vi "Digilens IPLC UI.vi"() -> ()   [LabVIEW 2022 SP3, in "TopLevel.lvclass"]
uses:
  TopLevel.lvclass
  IO/Typedefs/Pre Purge Parameters.ctl
  Motor Controller/Typedefs/API Command Cluster.ctl
  Motor Controller/Typedefs/API Command Enum.ctl
  Motor Controller/Typedefs/SetExplicitMessage API Data.ctl
  Motor Controller/Typedefs/Motor Controller Parameter-Set.ctl
  Motor Controller/Typedefs/Motor Controller Parameter-Get.ctl
  Typedefs/API Command Enum.ctl
  IO/Typedefs/ICP2-DO Channel Names.ctl
  IO/Typedefs/ICP1-D0 Channel Names.ctl
  Typedefs/API Command Cluster.ctl
  GIS Printer/Typedefs/PrintCmdParameters--Cluster.ctl
  GIS Printer/Typedefs/IdlePrintCmdParameters--Cluster.ctl
  IO/Typedefs/ICP1-AO Channel Names.ctl
  IO/Typedefs/ICP2-AO Channel Names.ctl
  IO/IO.lvclass
  GIS Printer/GIS Printer.lvclass
  Motor Controller/Motor Controller.lvclass
  Motor Controller/Typedefs/Status.ctl
  Typedefs/Motor Controller Config Data.ctl
  Motor Controller/Typedefs/Stage Move Data.ctl
  Motor Controller/Typedefs/Batch Index Speed Data.ctl
  Motor Controller/Typedefs/Move Status.ctl
  Typedefs/Digilens Config Cluster.ctl
  IO/Typedefs/IO Config Data.ctl
  IO/Typedefs/DCON_DeviceConfig--Cluster.ctl
  IO/Typedefs/Channel Data.ctl
  GIS Printer/Typedefs/PrinterConfiguration--Cluster.ctl
  DAQWFE/LV_Source/Subsystems/DAQ/DataTypes/TD DAQ Settings--cluster.ctl
  DAQWFE/LV_Source/Subsystems/DAQ/DataTypes/TD DI Instrument Settings--cluster.ctl
  DAQWFE/LV_Source/Subsystems/DAQ/DataTypes/TD AI Instrument Settings--cluster.ctl
  DAQWFE/LV_Source/Subsystems/DAQ/DataTypes/TD AI InstSettings--cluster.ctl
  DAQWFE/LV_Source/Subsystems/DAQ/Process/ProcessSupport/TD SimAI Ranges--cluster.ctl
  IO/Typedefs/Status Cluster.ctl
  IO/Typedefs/ICP2-DI Channel Names.ctl
  IO/Typedefs/ICP1-AI Channel Names.ctl
  Motor Controller/Typedefs/Status_TopLevel--Cluster.ctl
  IO/Typedefs/Device Names.ctl
  IO/Typedefs/DCON Action Engine-States.ctl
  DAQWFE/LV_Source/Subsystems/DAQ/DAQ.lvclass
panel:
  in  "Exit":bool
  in  "update":bool
  out "H 6":dbl
  out "H 5":dbl
  out "H 4":dbl
  out "H 3":dbl
  out "H 2":dbl
  out "H1":dbl
  in  "Tab Control":T1(tab)
  out "Print #":i32=1 min=1 step=1
  in  "HomeOnComplete":bool
  out "Stage Busy Printer":bool caption="Busy"
  in  "PH6-Prime":bool
  in  "PH5-Prime":bool
  in  "PH4-Prime":bool
  in  "PH3-Prime":bool
  in  "PH2-Prime":bool
  in  "PH1-Prime":bool
  in  "Abort":bool
  in  "Print Passes":i32=1 min=1 step=1
  in  "Home 2":bool
  in  "TCP Commands & Responses":i32(listbox)
  in  "Print":bool
  in  "Command File Path":path
  in  "Jog (+) 2":bool
  in  "Jog (-) 2":bool
  in  "Idle Intervals (s)":dbl=0.1
  in  "IdlePrint":bool
  in  "Head1 2":bool
  in  "Head2 2":bool
  in  "Head3 2":bool
  in  "Head4 2":bool
  in  "Head5 2":bool
  in  "Head6 2":bool
  in  "Enable PH1 Heat":bool
  in  "Enable PH2 Heat":bool
  in  "Enable PH3 Heat":bool
  in  "Enable PH4 Heat":bool
  in  "Enable PH5 Heat":bool
  in  "Enable PH6 Heat":bool
  in  "10Pass":bool
  in  "5Pass":bool
  in  "Enable Disable With DO":bool
  in  "Stage Abort":bool
  in  "ClearStageAlarm":bool
  out "Stage Busy (Stage)":bool caption="Stage Busy"
  in  "Print Speed":i32
  in  "Print (+)":bool
  in  "Print (-)":bool
  out "Status/Error :":string
  in  "Acceleration":dbl
  in  "Jog Speed":i32
  in  "Jog (+)":bool
  in  "Jog (-)":bool
  in  "Go":bool
  in  "Accel":dbl
  in  "Speed":i32
  in  "GoTo":i32
  out "Pulse/mm":dbl
  out "Position":dbl
  out "Enabled":bool
  in  "Enable Disable":bool
  in  "Head6":bool
  in  "Head5":bool
  in  "Head4":bool
  in  "Head3":bool
  in  "Head2":bool
  in  "Head1":bool
  in  "Home":bool
  in  "Laminate":bool
  in  "Load":bool
  in  "Read Status":bool
  out "Stage Busy (Moves)":bool caption="Stage Busy"
  out "Status":string
  in  "Stage Move Status":i32(listbox)
  in  "Start":bool
  in  "Stage Recipe XML File Path":path
  out "PrePrgPrint #":i32=1 min=1 step=1
  in  "PPDuration (s)":dbl=3.0
  in  "Pre Purge PH Ch-6 Parameters":T2={"GIS File Path"=path "", "Duration (s)"=0.1, "No. of Repeats"=1}
  in  "Pre Purge PH Ch-5 Parameters":T2={"GIS File Path"=path "", "Duration (s)"=0.1, "No. of Repeats"=1}
  in  "Pre Purge PH Ch-3 Parameters":T2={"GIS File Path"=path "", "Duration (s)"=0.1, "No. of Repeats"=1}
  in  "Pre Purge PH Ch-4 Parameters":T2={"GIS File Path"=path "", "Duration (s)"=0.1, "No. of Repeats"=1}
  in  "Pre Purge PH Ch-2 Parameters":T2={"GIS File Path"=path "", "Duration (s)"=0.1, "No. of Repeats"=1}
  in  "Pre Purge PH Ch-1 Parameters":T2={"GIS File Path"=path "", "Duration (s)"=0.1, "No. of Repeats"=1}
  in  "Pre Purge PH Ch-1":bool
  in  "Pre Purge PH Ch-2":bool
  in  "Pre Purge PH Ch-3":bool
  in  "Pre Purge PH Ch-4":bool
  in  "Pre Purge PH Ch-5":bool
  in  "Pre Purge PH Ch-6":bool
  out "Purge PH Ch-1":bool
  in  "Purge PH Ch-2":bool
  in  "Purge PH Ch-3":bool
  in  "Purge PH Ch-4":bool
  in  "Purge PH Ch-5":bool
  in  "Purge PH Ch-6":bool
  in  "Duration (s)":dbl=3.0
  in  "Jog (-) 3":bool
  in  "Jog (+) 3":bool
  in  "Head6 3":bool
  in  "Head5 3":bool
  in  "Head4 3":bool
  in  "Head3 3":bool
  in  "Head2 3":bool
  in  "Head1 3":bool
  in  "Home 3":bool
  in  "Spit 6":bool
  in  "Spit 5":bool
  in  "Spit 4":bool
  in  "Spit 3":bool
  in  "Spit 2":bool
  in  "Spit 1":bool
  in  "Spit 6 LOV":u16(ring)
  in  "Spit 5 LOV":u16(ring)
  in  "Spit 4 LOV":u16(ring)
  in  "Spit 3 LOV":u16(ring)
  in  "Spit 2 LOV":u16(ring)
  in  "Spit 1 LOV":u16(ring)
  out "Res 6 Meniscus":dbl
  out "Res 5 Meniscus":dbl
  out "Res 4 Meniscus":dbl
  out "Res 3 Meniscus":dbl
  out "Res 2 Meniscus":dbl
  out "Res 1 Meniscus":dbl
  in  "Res 6 Recirculate":dbl
  in  "Res 5 Recirculate":dbl
  in  "Res 4 Recirculate":dbl
  in  "Res 3 Recirculate":dbl
  in  "Res 2 Recirculate":dbl
  in  "Res 1 Recirculate":dbl
  in  "Res 6 Enabled":bool
  in  "Res 5 Enabled":bool
  in  "Res 4 Enabled":bool
  in  "Res 3 Enabled":bool
  in  "Res 2 Enabled":bool
  in  "Res 1 Enabled":bool
  in  "Head 6 Set":bool
  in  "Head 6 Set Temp":dbl
  out "Head 6 Act Temp":dbl
  in  "Head 5 Set":bool
  in  "Head 5 Set Temp":dbl
  out "Head 5 Act Temp":dbl
  in  "Head 4 Set":bool
  in  "Head 4 Set Temp":dbl
  out "Head 4 Act Temp":dbl
  in  "Head 3 Set":bool
  in  "Head 3 Set Temp":dbl
  out "Head 3 Act Temp":dbl
  in  "Head 2 Set":bool
  in  "Head 2 Set Temp":dbl
  out "Head 2 Act Temp":dbl
  in  "Head 1 Set":bool
  in  "Head 1 Set Temp":dbl
  out "Head 1 Act Temp":dbl
  in  "Head 6 Material":u16(ring) items=["none", "113A.3", "507.2-1", "109G"]
  in  "Head 5 Material":u16(ring) items=["none", "113A.3", "507.2-1", "109G"]
  in  "Head 4 Material":u16(ring) items=["none", "113A.3", "507.2-1", "109G"]
  in  "Head 3 Material":u16(ring) items=["none", "113A.3", "507.2-1", "109G"]
  in  "Head 2 Material":u16(ring) items=["none", "113A.3", "507.2-1", "109G"]
  in  "Enable Ink Ch-6":bool
  in  "Enable Ink Ch-5":bool
  in  "Enable Ink Ch-4":bool
  in  "Enable Ink Ch-3":bool
  in  "Enable Ink Ch-2":bool
  in  "Enable Ink Ch-1":bool
  in  "Head 1 Material":u16(ring) items=["none", "113A.3", "507.2-1", "109G"]
  out "SW - COVER INPUT SIDE (M)":bool
  out "SW - COVER OUTPUT SIDE (M)":bool
  out "Purge Valve Open - R6 Status":bool
  out "Purge Valve Open - R5 Status":bool
  out "Purge Valve Open - R4 Status":bool
  out "Purge Valve Open - R3 Status":bool
  out "Purge Valve Open - R2 Status":bool
  out "Purge Valve Open - R1 Status":bool
  out "Meniscus Pressure Reg PWR - R6 Status":bool
  out "Meniscus Pressure Reg PWR - R5 Status":bool
  out "Meniscus Pressure Reg PWR - R4 Status":bool
  out "Meniscus Pressure Reg PWR - R3 Status":bool
  out "Meniscus Pressure Reg PWR - R2 Status":bool
  out "Meniscus Pressure Reg PWR - R1 Status":bool
  out "Recirc Pump On - R6 Status":bool
  out "Recirc Pump On - R5 Status":bool
  out "Recirc Pump On - R4 Status":bool
  out "Recirc Pump On - R3 Status":bool
  out "Recirc Pump On - R2 Status":bool
  out "Recirc Pump On - R1 Status":bool
  out "SW_LED - Ink Valve - R6 Status":bool
  out "SW_LED - Ink Valve - R5 Status":bool
  out "SW_LED - Ink Valve - R4 Status":bool
  out "SW_LED - Ink Valve - R3 Status":bool
  out "SW_LED - Ink Valve - R2 Status":bool
  out "SW_LED - Ink Valve - R1 Status":bool
  out "Ink Flow Valve Open - R5 Status":bool
  out "Ink Flow Valve Open - R4 Status":bool
  out "Ink Flow Valve Open - R3 Status":bool
  out "Ink Flow Valve Open - R2 Status":bool
  out "Ink Flow Valve Open - R1 Status":bool
  out "Meniscus Valve Open - R6 Status":bool
  out "Meniscus Valve Open - R5 Status":bool
  out "Meniscus Valve Open - R4 Status":bool
  out "Meniscus Valve Open - R3 Status":bool
  out "Ink Flow Valve Open - R6 Status":bool
  out "Meniscus Valve Open - R2 Status":bool
  out "Meniscus Valve Open - R1 Status":bool
  in  "Purge Valve Open - R6":bool
  in  "Purge Valve Open - R5":bool
  in  "Purge Valve Open - R4":bool
  in  "Purge Valve Open - R3":bool
  in  "Purge Valve Open - R2":bool
  in  "Purge Valve Open - R1":bool
  in  "Meniscus Pressure Reg PWR - R6":bool
  in  "Meniscus Pressure Reg PWR - R5":bool
  in  "Meniscus Pressure Reg PWR - R4":bool
  in  "Meniscus Pressure Reg PWR - R3":bool
  in  "Meniscus Pressure Reg PWR - R2":bool
  in  "Meniscus Pressure Reg PWR - R1":bool
  in  "Recirc Pump On - R6":bool
  in  "Recirc Pump On - R5":bool
  in  "Recirc Pump On - R4":bool
  in  "Recirc Pump On - R3":bool
  in  "Recirc Pump On - R2":bool
  in  "Recirc Pump On - R1":bool
  in  "SW_LED - Ink Valve - R6":bool
  in  "SW_LED - Ink Valve - R5":bool
  in  "SW_LED - Ink Valve - R4":bool
  in  "SW_LED - Ink Valve - R3":bool
  in  "SW_LED - Ink Valve - R2":bool
  in  "SW_LED - Ink Valve - R1":bool
  in  "Ink Flow Valve Open - R6":bool
  in  "Ink Flow Valve Open - R5":bool
  in  "Ink Flow Valve Open - R4":bool
  in  "Ink Flow Valve Open - R3":bool
  in  "Ink Flow Valve Open - R2":bool
  in  "Ink Flow Valve Open - R1":bool
  in  "Meniscus Valve Open - R6":bool
  in  "Meniscus Valve Open - R5":bool
  in  "Meniscus Valve Open - R4":bool
  in  "Meniscus Valve Open - R3":bool
  in  "Meniscus Valve Open - R2":bool
  out "SW - Purge - R6":bool
  out "SW - Purge - R5":bool
  out "SW - Purge - R4":bool
  out "SW - Purge - R3":bool
  out "SW - Purge - R1":bool
  out "SW - Purge - R2":bool
  out "SW - COVER OUTPUT SIDE":bool
  out "SW - COVER INPUT SIDE":bool
  out "SW - Ink Valve - R6":bool
  out "SW - Ink Valve - R5":bool
  out "SW - Ink Valve - R4":bool
  out "SW - Ink Valve - R3":bool
  out "SW - Ink Valve - R1":bool
  out "SW - Ink Valve - R2":bool
  in  "Meniscus Valve Open - R1":bool
  out "Recirc Pump Flow Set - R6 Status":dbl
  out "Recirc Pump Flow Set - R5 Status":dbl
  out "Recirc Pump Flow Set - R4 Status":dbl
  out "Recirc Pump Flow Set - R3 Status":dbl
  out "Recirc Pump Flow Set - R2 Status":dbl
  out "Recirc Pump Flow Set - R1 Status":dbl
  out "Meniscus Pressure Set - R6 Status":dbl
  out "Meniscus Pressure Set - R5 Status":dbl
  out "Meniscus Pressure Set - R4 Status":dbl
  out "Meniscus Pressure Set - R3 Status":dbl
  out "Meniscus Pressure Set - R2 Status":dbl
  out "Meniscus Pressure Set - R1 Status":dbl
  in  "Recirc Pump Flow Set - R6 Set":bool
  in  "Recirc Pump Flow Set - R5 Set":bool
  in  "Recirc Pump Flow Set - R4 Set":bool
  in  "Recirc Pump Flow Set - R3 Set":bool
  in  "Recirc Pump Flow Set - R2 Set":bool
  in  "Recirc Pump Flow Set - R1 Set":bool
  in  "Recirc Pump Flow Set - R6":dbl
  in  "Recirc Pump Flow Set - R5":dbl
  in  "Recirc Pump Flow Set - R4":dbl
  in  "Recirc Pump Flow Set - R3":dbl
  in  "Recirc Pump Flow Set - R2":dbl
  in  "Recirc Pump Flow Set - R1":dbl
  in  "Meniscus Pressure Set - R6-Set":bool
  in  "Meniscus Pressure Set - R5-Set":bool
  in  "Meniscus Pressure Set - R4-Set":bool
  in  "Meniscus Pressure Set - R3-Set":bool
  in  "Meniscus Pressure Set - R2-Set":bool
  in  "Meniscus Pressure Set - R1-Set":bool
  in  "Meniscus Pressure Set - R6":dbl
  in  "Meniscus Pressure Set - R5":dbl
  in  "Meniscus Pressure Set - R4":dbl
  in  "Meniscus Pressure Set - R3":dbl
  in  "Meniscus Pressure Set - R2":dbl
  in  "Meniscus Pressure Set - R1":dbl
  out "Meniscus Pressure Read - R6":dbl
  out "Meniscus Pressure Read - R5":dbl
  out "Meniscus Pressure Read - R4":dbl
  out "Meniscus Pressure Read - R3":dbl
  out "Meniscus Pressure Read - R2":dbl
  out "Meniscus Pressure Read - R1":dbl
  out "TopLevel Out":refnum<class "TopLevel.lvclass">
  in  "TopLevel In":refnum<class "TopLevel.lvclass">
  # "PrePrint"
  # "Move to Position"
  # "Prepurge Script File Path"
  # "Repeat Interval (s)"
  # "Repeats"
  # "Purge"
  # "1"
  # "2"
  # "3"
  # "4"
  # "5"
  # "6"
  # "Covered"
  # "Head Temp"
  # "Reservoir"
  # "Head"
  # "En"
  # "Material"
  # "Actual"
  # "Set"
  # "Recirculate"
  # "Meniscus"
  # "Spit"
  # "1"
  # "1"
  # "1"
  # "1"
  # "1"
  # "2"
  # "2"
  # "2"
  # "2"
  # "2"
  # "3"
  # "3"
  # "3"
  # "3"
  # "3"
  # "4"
  # "4"
  # "4"
  # "4"
  # "4"
  # "5"
  # "5"
  # "5"
  # "5"
  # "5"
  # "6"
  # "6"
  # "6"
  # "6"
  # "6"
  # "ICP2-DI"
  # "ICP2-DO"
  # "ICP1-DO"
  # "ICP1-AI"
  # "ICP1-AO"
  # "ICP2-AO"
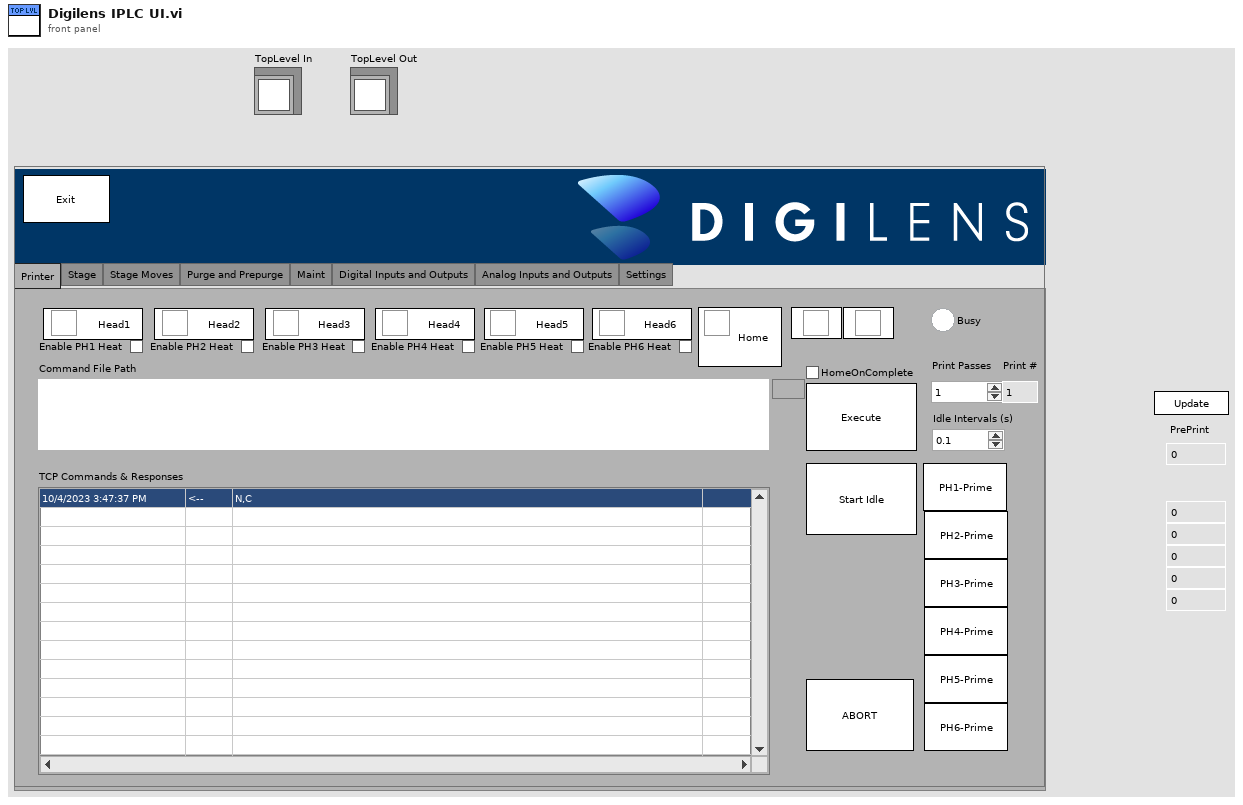
[diagram p1: front panel]
types:
  T1 = enum32{"Printer", "Stage", "Stage Moves", "Purge and Prepurge", "Maint", "Digital Inputs and Outputs", "Analog Inputs and Outputs", "Settings"}
  T2 = typedef "TopLevel.lvclass/Pre Purge Parameters.ctl" = cluster{"GIS File Path":path, "Duration (s)":dbl, "No. of Repeats":i32}
  T3 = typedef "Motor Controller.lvclass/SetExplicitMessage API Data.ctl" = cluster{"Motor Controller Parameter":T4, "value":i32}
  T4 = typedef "Motor Controller.lvclass/Motor Controller Parameter-Set.ctl" = enum16{"Print Speed", "Jog Speed", "PR Path", "Enable Servo", "Disable Servo", "Move Stage to Under PH1", "Move Stage to Under PH2", "Move Stage to Under PH3", "Move Stage to Under PH4", "Move Stage to Under PH5", "Move Stage to Under PH6", "Home Stage", "Return Stage to 0", "Print Stage", "Write Speed", "Write Index", "Stop Stage"}
  T5 = typedef "Motor Controller.lvclass/API Command Enum.ctl" = enum16{"GetExplicitMessage", "SetExplicitMessage", "Execute Stage Move Recipe", "Read Stage Move Recipe", "Abort"}
  T6 = typedef "Motor Controller.lvclass/API Command Cluster.ctl" = cluster{"Command":T5, "Arguments":string, "Data":variant}
  T7 = typedef "Motor Controller.lvclass/Motor Controller Parameter-Get.ctl" = enum16{"Print Speed", "Jog Speed", "PR Path", "Servo Enabled?", "AlarmCodes"}
  T8 = typedef "TopLevel.lvclass/API Command Enum.ctl" = enum16{"Execute Printer Commands", "Pre Purge", "Enable Ink Ch-1", "Enable Ink Ch-2", "Enable Ink Ch-3", "Enable Ink Ch-4", "Enable Ink Ch-5", "Enable Ink Ch-6", "Disable Ink Ch-1", "Disable Ink Ch-2", "Disable Ink Ch-3", "Disable Ink Ch-4", "Disable Ink Ch-5", "Disable Ink Ch-6", "ExecuteIdlePrintCycle", "StopIdlePrintCycle", "Abort", "LoadDLP2GUIConfig", "SaveDLP2GUIConfig", "PrimingMode", "SetHeadTemperature", "EnableHead", "EnableHeadHeat", "SetSystemMode", "HeadPrint", "AbortAll", "Send Printer String", "WriteInitXML"}
  T9 = typedef "IO.lvclass/ICP2-DO Channel Names.ctl" = enum16{"None", "Meniscus Valve Open - R1", "Meniscus Valve Open - R2", "Meniscus Valve Open - R3", "Meniscus Valve Open - R4", "Meniscus Valve Open - R5", "Meniscus Valve Open - R6", "Ink Flow Valve Open - R1", "Ink Flow Valve Open - R2", "Ink Flow Valve Open - R3", "Ink Flow Valve Open - R4", "Ink Flow Valve Open - R5", "Ink Flow Valve Open - R6", "SW_LED - Ink Valve - R1", "SW_LED - Ink Valve - R2", "SW_LED - Ink Valve - R3", "Recirc Pump On - R1", "Recirc Pump On - R2", "Recirc Pump On - R3", "Recirc Pump On - R4", "Recirc Pump On - R5", "Recirc Pump On - R6", "SW_LED - Ink Valve - R4", "SW_LED - Ink Valve - R5", "SW_LED - Ink Valve - R6"}
  T10 = typedef "IO.lvclass/ICP1-D0 Channel Names.ctl" = enum16{"None", "Meniscus Pressure Reg PWR - R1", "Meniscus Pressure Reg PWR - R2", "Meniscus Pressure Reg PWR - R3", "Meniscus Pressure Reg PWR - R4", "Meniscus Pressure Reg PWR - R5", "Meniscus Pressure Reg PWR - R6", "Clear Stage Alarm", "Servo ON", "Purge Valve Open - R1", "Purge Valve Open - R2", "Purge Valve Open - R3", "Purge Valve Open - R4", "Purge Valve Open - R5", "Purge Valve Open - R6"}
  T11 = typedef "PrintCmdParameters--Cluster.ctl" = cluster{"Command File Path":path, "No. of Print Repeats":i32, "HomeOnComplete":bool}
  T12 = typedef "TopLevel.lvclass/API Command Cluster.ctl" = cluster{"Command":T8, "Arguments":string, "Data":variant}
  T13 = typedef "IdlePrintCmdParameters--Cluster.ctl" = cluster{"Command File Path":path, "IdleMode":bool, "IdleCycleInterval(s)":dbl}
  T14 = typedef "IO.lvclass/ICP1-AO Channel Names.ctl" = enum16{"None", "Meniscus Pressure Set - R1", "Meniscus Pressure Set - R2", "Meniscus Pressure Set - R3", "Meniscus Pressure Set - R4", "Meniscus Pressure Set - R5", "Meniscus Pressure Set - R6", "Meniscus Vac Pump Speed"}
  T15 = typedef "IO.lvclass/ICP2-AO Channel Names.ctl" = enum16{"None", "Recirc Pump Flow Set - R1", "Recirc Pump Flow Set - R2", "Recirc Pump Flow Set - R3", "Recirc Pump Flow Set - R4", "Recirc Pump Flow Set - R5", "Recirc Pump Flow Set - R6"}
  T16 = enum32{"invalid app kind", "Development System", "Run Time System", "Student Edition", "Embedded LabVIEW", "Evaluation", "Custom"}
  T17 = typedef "Motor Controller.lvclass/Status.ctl" = cluster{"Motor Controller Config Data":T18, "Motor Controller Data":cluster{"Enabled?":bool}, "Stage Move":T19, "Stage Busy?":bool}
  T18 = typedef "Motor Controller.lvclass/Motor Controller Config Data.ctl" = cluster{"Motor IP Addresss":string, "Current Position":i32, "Pulse_Per_mm":i32, "PrePrint":dbl[], "Load Position_mm":i32, "Laminate Position_mm":i32}
  T19 = typedef "Motor Controller.lvclass/Stage Move Data.ctl" = cluster{"Current Step":string, "Move Data":T20[]}
  T20 = typedef "Motor Controller.lvclass/Batch Index Speed Data.ctl" = cluster{"Batch & Cycle":string, "Move":cluster{"Index_mm":i32, "Speed_mm_s":i32}, "Status":T21}
  T21 = typedef "Motor Controller.lvclass/Move Status.ctl" = enum16{"Pending", "In Progress", "Completed"}
  T22 = enum8{"Enabled", "Disabled", "Disabled and Grayed Out"}
  T23 = enum32{"Invalid", "Standard", "Closed", "Hidden", "Minimized", "Maximized"}
  T24 = typedef "DCON Action Engine-States.ctl" = enum16{"Open", "Close", "Set DO Value", "Get Digital Status", "Get Data", "Get AI Status", "Set AO Value", "Get AO Status"}
  T25 = typedef "IO.lvclass/Device Names.ctl" = enum16{"ICP1-DO", "ICP2-DI", "ICP2-DO", "ICP1-AI", "ICP1-AO", "ICP2-AO"}
  T26 = typedef "TopLevel.lvclass/Digilens Config Cluster.ctl" = cluster{"Motion Controller":T18, "IO Config":T27, "PrinterConfiguration":T30, "DAQ Settings":T31}
  T27 = typedef "IO.lvclass/IO Config Data.ctl" = cluster{"DAQDevices":T28[], "DI Channels":T29[], "DO Channels":T29[], "Material Names":string[], "AI Channels":T29[], "AO Channels":T29[]}
  T28 = typedef "IO.lvclass/DCON_DeviceConfig--Cluster.ctl" = cluster{"COM":string, "DeviceName":string, "BaudRate":u32, "Number of Channels":i32, "DeviceAddress":i32, "Enable":bool}
  T29 = typedef "IO.lvclass/Channel Data.ctl" = cluster{"Channel Name":string, "Device Name":string, "Channel No":string}
  T30 = typedef "GIS Printer.lvclass/PrinterConfiguration--Cluster.ctl" = cluster{"IPAddress":string, "Move Stage on RTP Command?":bool, "Stage Move Position":string, "PH1-Prime Path":path, "PH2-Prime Path":path, "PH3-Prime Path":path, "PH4-Prime Path":path, "PH5-Prime Path":path, "PH6-Prime Path":path, "PrintScriptsFolder":path, "PurgeScriptsFolder":path, "StageScriptsFolder":path, "PH1-HeatOn Path":path, "PH2-HeatOn Path":path, "PH3-HeatOn Path":path, "PH4-HeatOn Path":path, "PH5-HeatOn Path":path, "PH6-HeatOn Path":path, "PH1-HeatOff Path":path, "PH2-HeatOff Path":path, "PH3-HeatOff Path":path, "PH4-HeatOff Path":path, "PH5-HeatOff Path":path, "PH6-HeatOff Path":path}
  T31 = typedef "DAQ.lvclass/TD DAQ Settings--cluster.ctl" = cluster{"Simulate DAQ":bool, "DI Settings":T32[], "AI Settings":T33[], "Relay IONames":string[], "AO IONames":string[], "AO NChan SingleTask":bool}
  T32 = typedef "DAQ.lvclass/TD DI Instrument Settings--cluster.ctl" = cluster{"Disable":bool, "DI TaskName":string, "DI RefreshIntv":i32}
  T33 = typedef "DAQ.lvclass/TD AI Instrument Settings--cluster.ctl" = cluster{"Disable":bool, "AI TaskName":string, "AI InstSettings":T34, "SimAI Ranges":T35}
  T34 = typedef "DAQ.lvclass/TD AI InstSettings--cluster.ctl" = cluster{"DaqRate":dbl, "NumSamples":i32}
  T35 = typedef "DAQ.lvclass/TD SimAI Ranges--cluster.ctl" = cluster{"lo":dbl, "hi":dbl}
  T36 = cluster{"Core":cluster{"Current VI Reference":refnum<vi>, "Close Panel on Exit?":bool}, "IO":refnum<class "IO.lvclass">, "GIS Printer":refnum<class "GIS Printer.lvclass">, "Motor Controller":refnum<class "Motor Controller.lvclass">, "Methods:Accessors:Digilens Config":T26, "Status":T17, "Exit Event":refnum<user-event>, "Purge\\PrePurge Channel Name":T10, "Pre Purge Parameters":T2, "API Command":T8, "TopLevel out":refnum<class "TopLevel.lvclass">}
  T37 = cluster{"Current VI Reference":refnum<vi>, "Close Panel on Exit?":bool}
  T38 = typedef "TopLevel.lvclass/UserEvents.ctl" = cluster{"API Incoming Event":refnum<user-event>, "API Executed Event":refnum<user-event>, "API Return Event":refnum<user-event>, "Exit Event":refnum<user-event>, "StatusChanged":refnum<user-event>, "DLP GUI Config Changed":refnum<user-event>, "AppEvent":refnum<user-event>, "Login Event":refnum<user-event>, "HeadPrimeStatusEvent":refnum<user-event>}
  T39 = typedef "Motor Controller.lvclass/UserEvents.ctl" = cluster{"API Incoming Event":refnum<user-event>, "API Executed Event":refnum<user-event>, "API Return Event":refnum<user-event>, "Status Changed Event":refnum<user-event>, "StopEvent":refnum<user-event>}
  T40 = typedef "IO.lvclass/UserEvents.ctl" = cluster{"API Incoming Event":refnum<user-event>, "API Executed Event":refnum<user-event>, "API Return Event":refnum<user-event>, "Status Changed Event":refnum<user-event>}
  T41 = typedef "GIS Printer.lvclass/UserEvents.ctl" = cluster{"API Incoming Event":refnum<user-event>, "API Executed Event":refnum<user-event>, "API Return Event":refnum<user-event>, "Status Changed Event":refnum<user-event>, "Abort":refnum<user-event>, "stop process":refnum<user-event>, "GISPollStatus":refnum<user-event>, "GISHeadStatus":refnum<user-event>, "Error Event":refnum<user-event>}
  T42 = typedef "IO.lvclass/DCON Private Data.ctl" = cluster{"DeviceName":string, "Number of Channels":i32, "COM":refnum<visa-resource-name>, "Status String":string, "Input String":string, "Value ":i32, "Digital Bits Value":bool[], "Analog Values":dbl[], "DeviceAddress":i32, "Enable":bool}
  T43 = typedef "IO.lvclass/ICP2-DI Channel Names.ctl" = enum16{"None", "SW - Ink Valve - R1", "SW - Ink Valve - R2", "SW - Ink Valve - R3", "SW - Ink Valve - R4", "SW - Ink Valve - R5", "SW - Ink Valve - R6", "SW - COVER INPUT SIDE", "SW - COVER OUTPUT SIDE", "SW - Purge - R1", "SW - Purge - R2", "SW - Purge - R3", "SW - Purge - R4", "SW - Purge - R5", "SW - Purge - R6"}
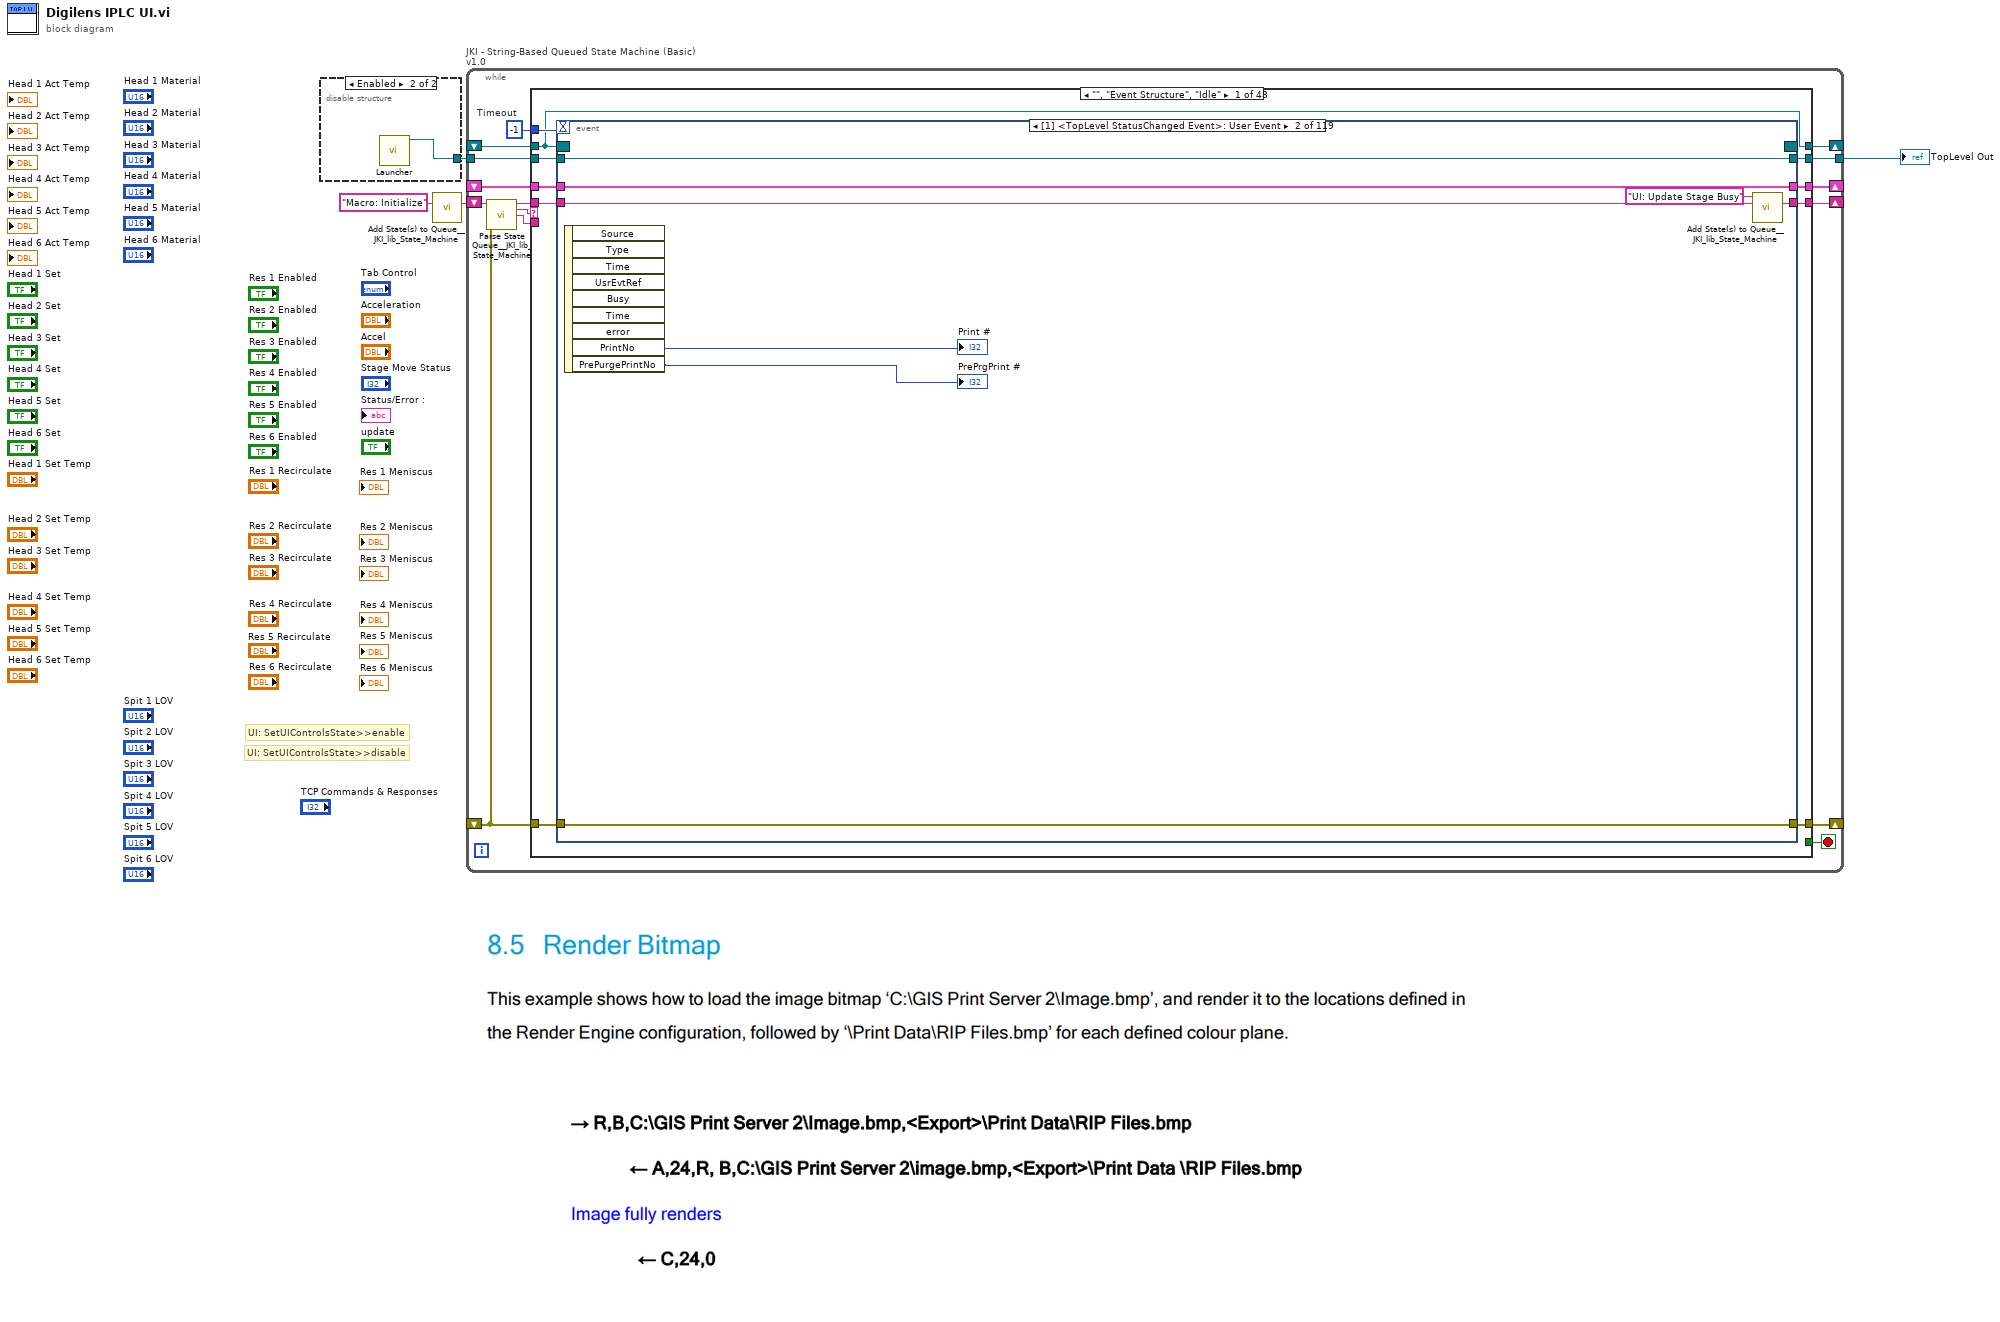
[diagram p0: block diagram]
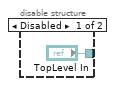
[diagram p2: hidden frame]
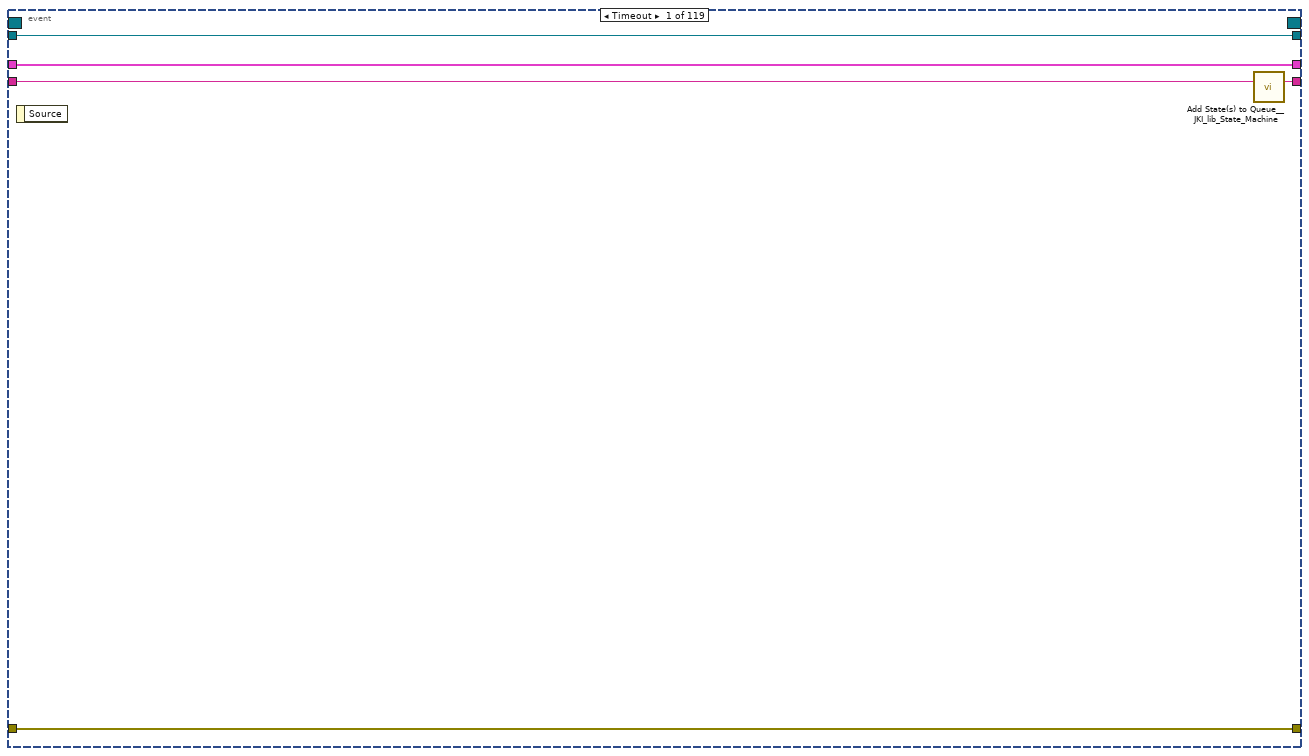
[diagram p3: hidden frame]
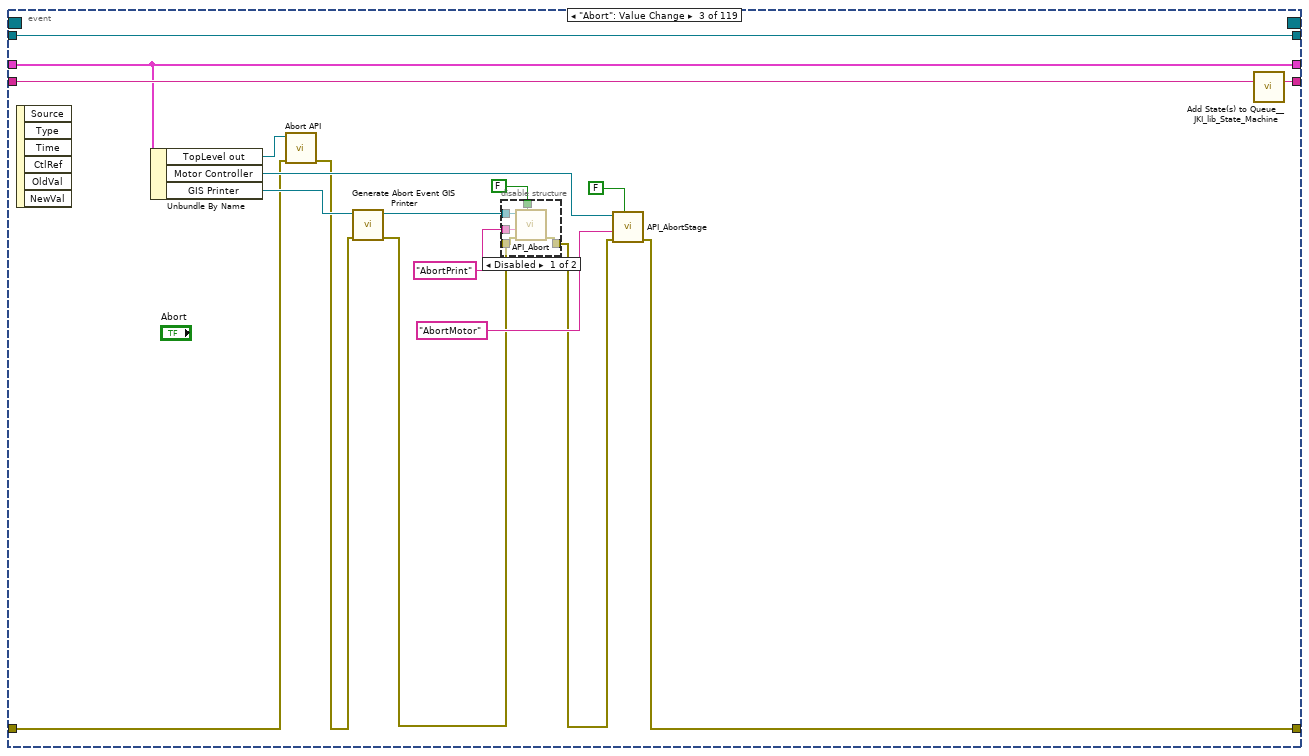
[diagram p4: hidden frame]
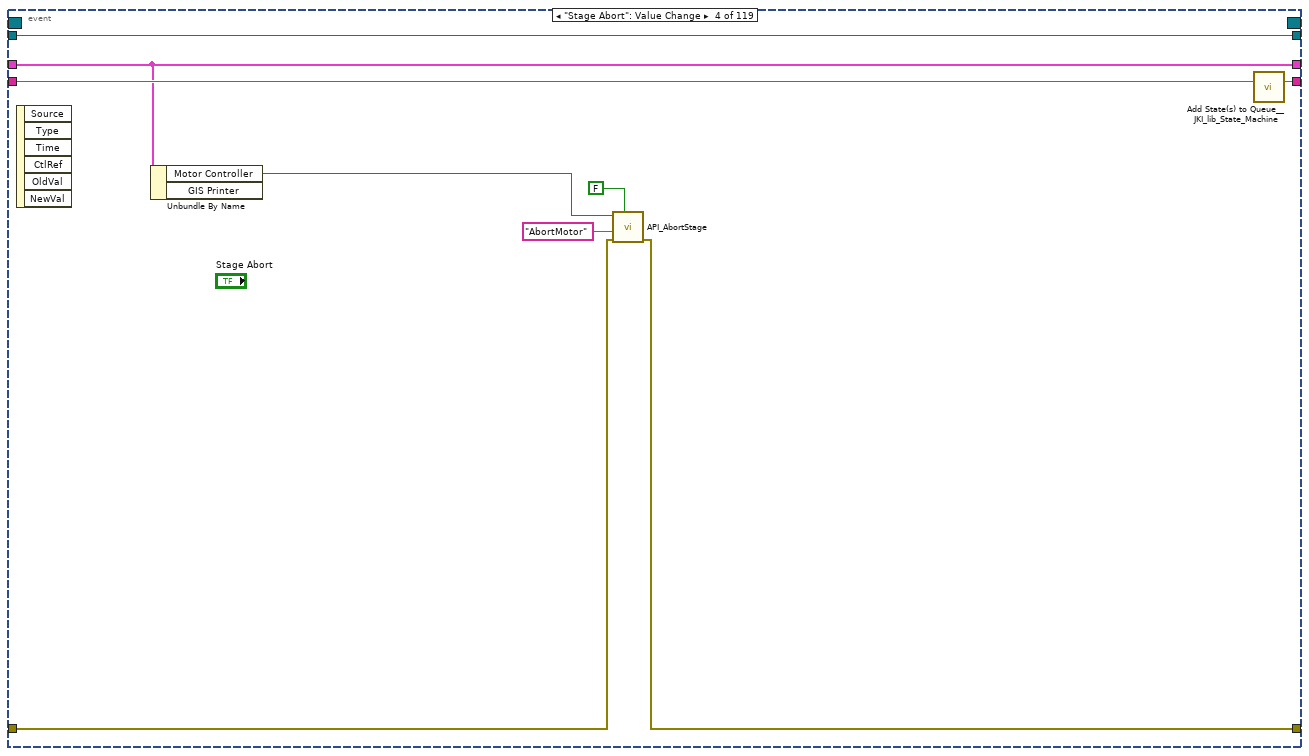
[diagram p6: hidden frame]
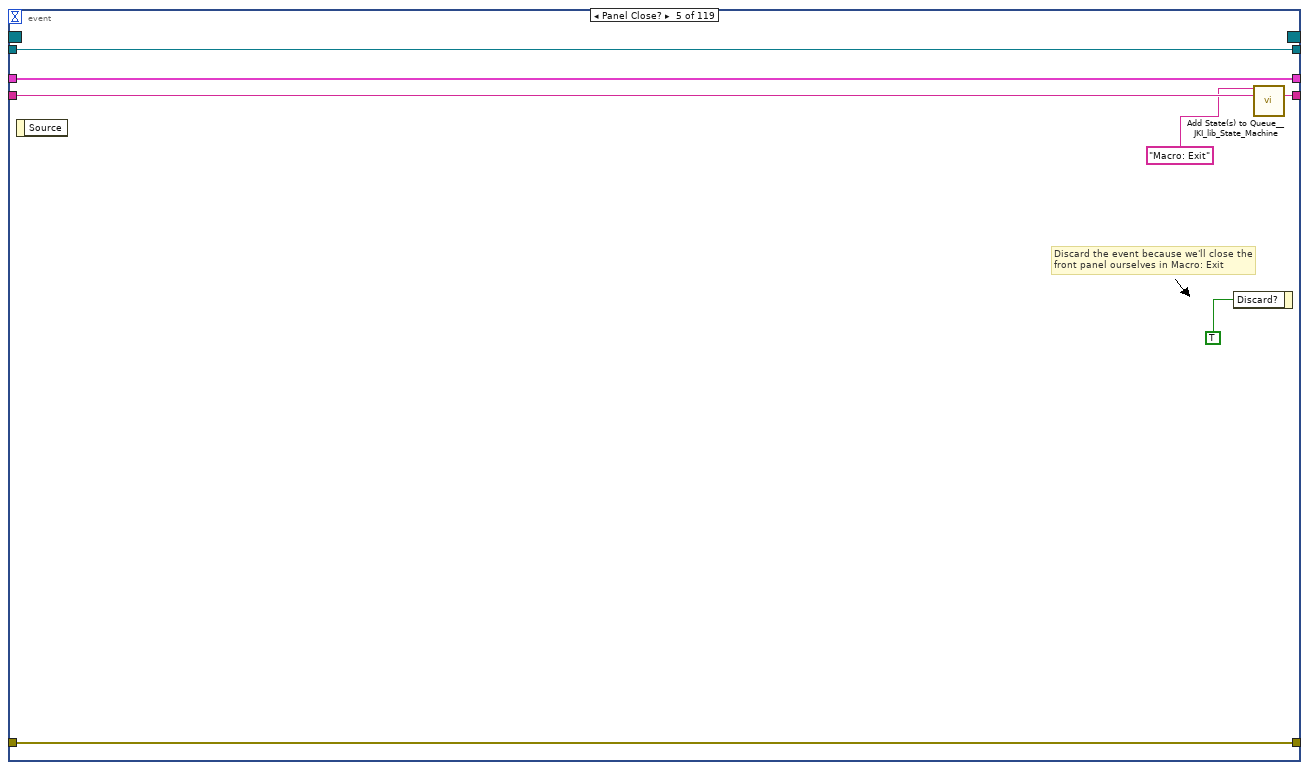
[diagram p7: hidden frame]
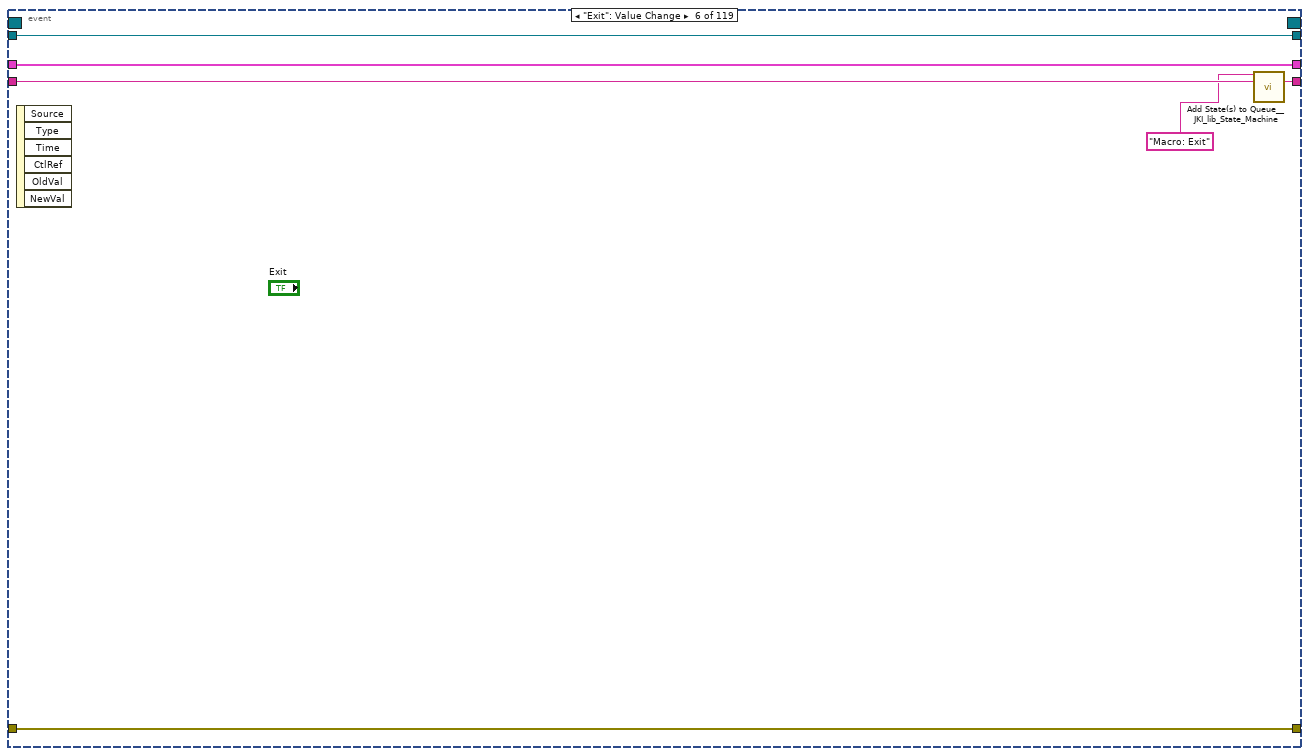
[diagram p8: hidden frame]
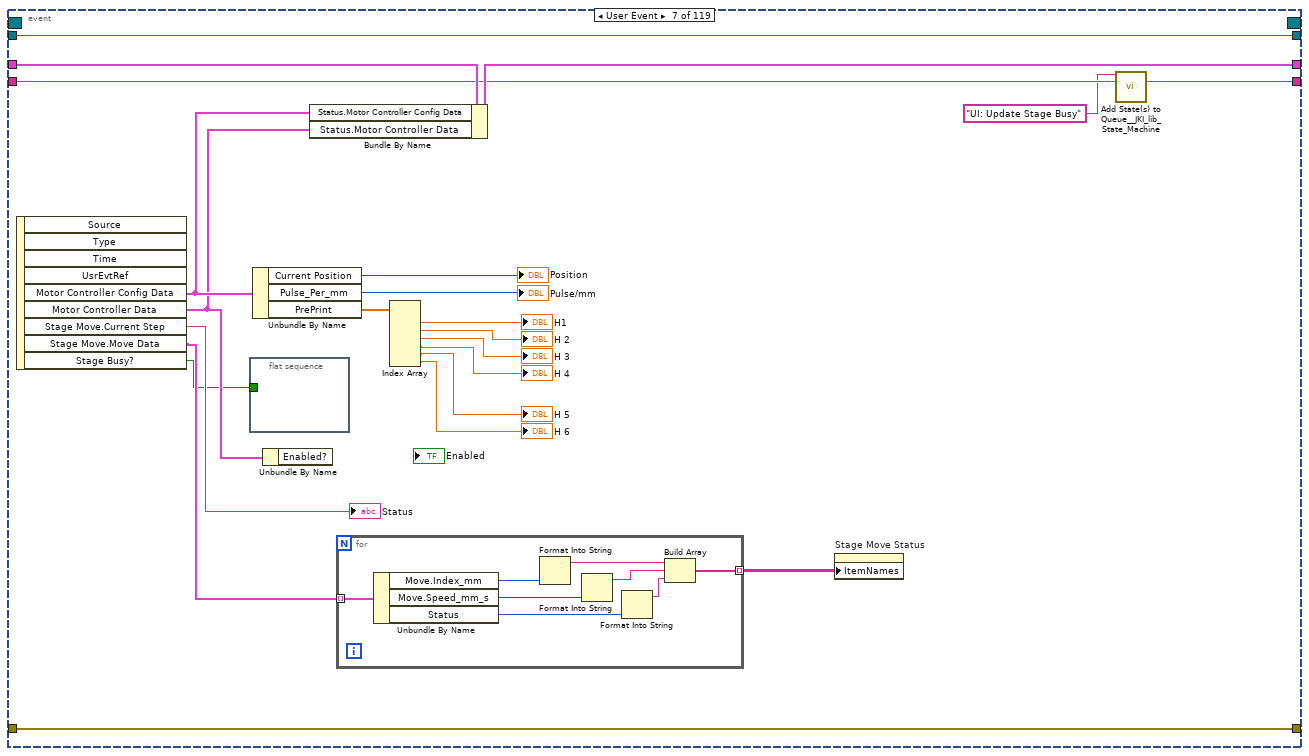
[diagram p9: hidden frame]
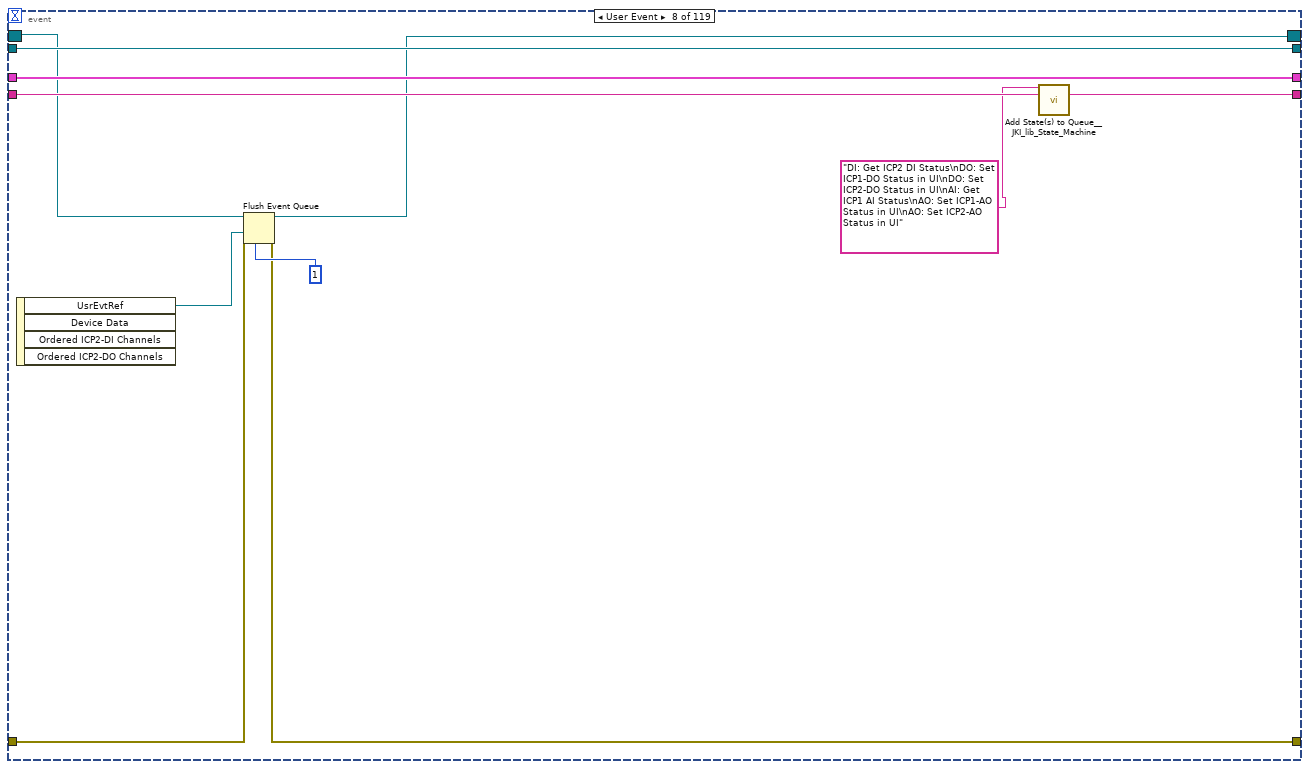
[diagram p10: hidden frame]
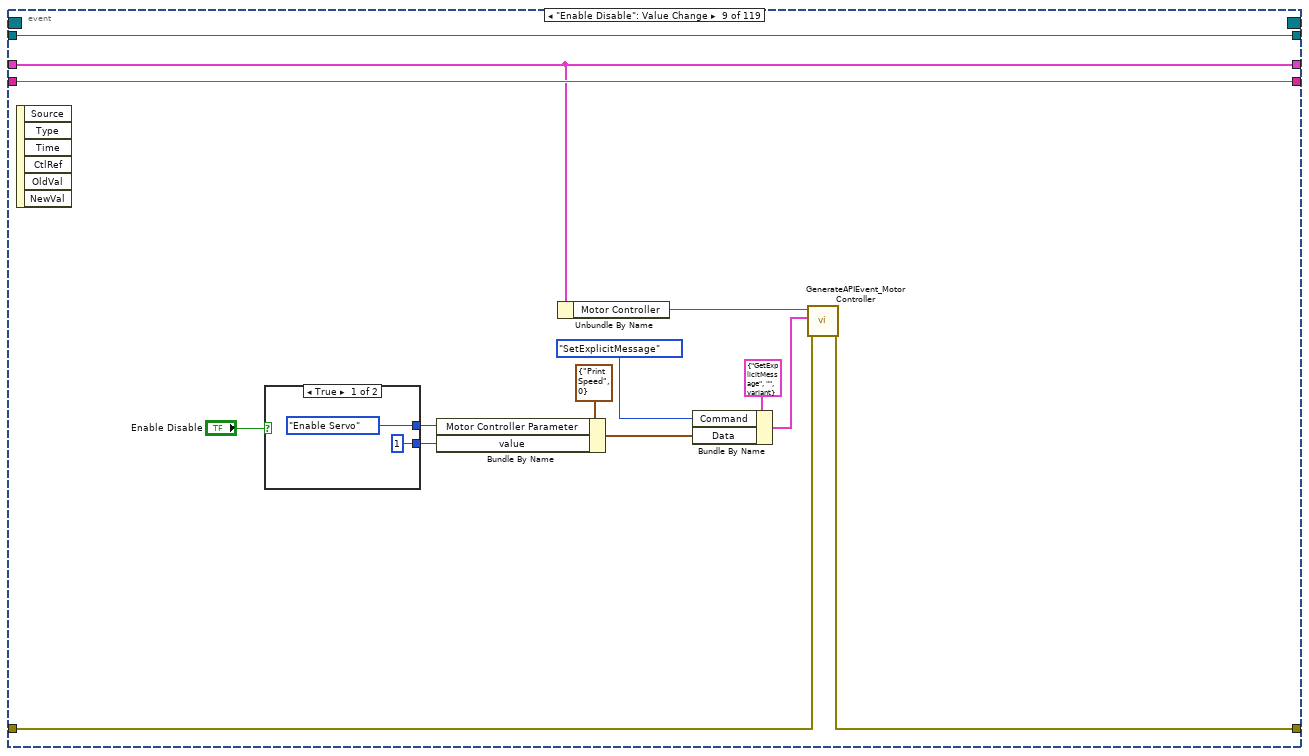
[diagram p11: hidden frame]
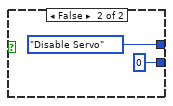
[diagram p12: hidden frame]
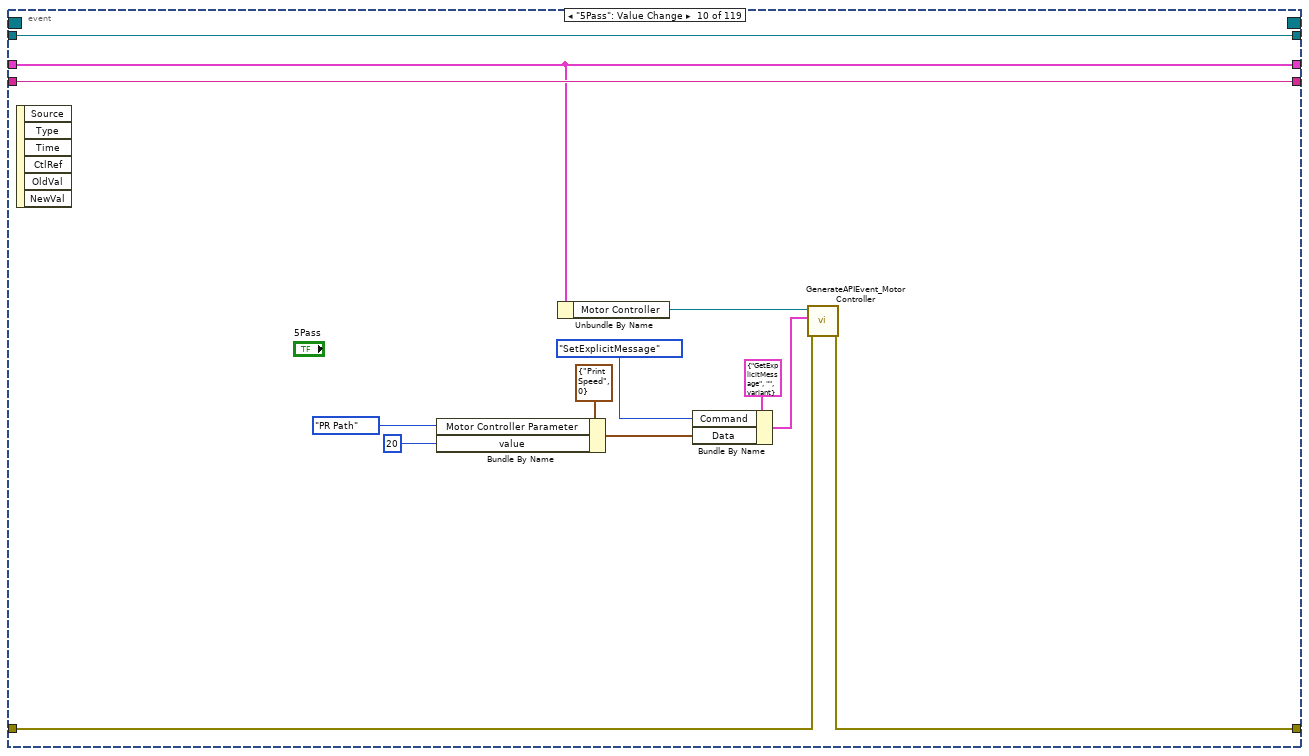
[diagram p13: hidden frame]
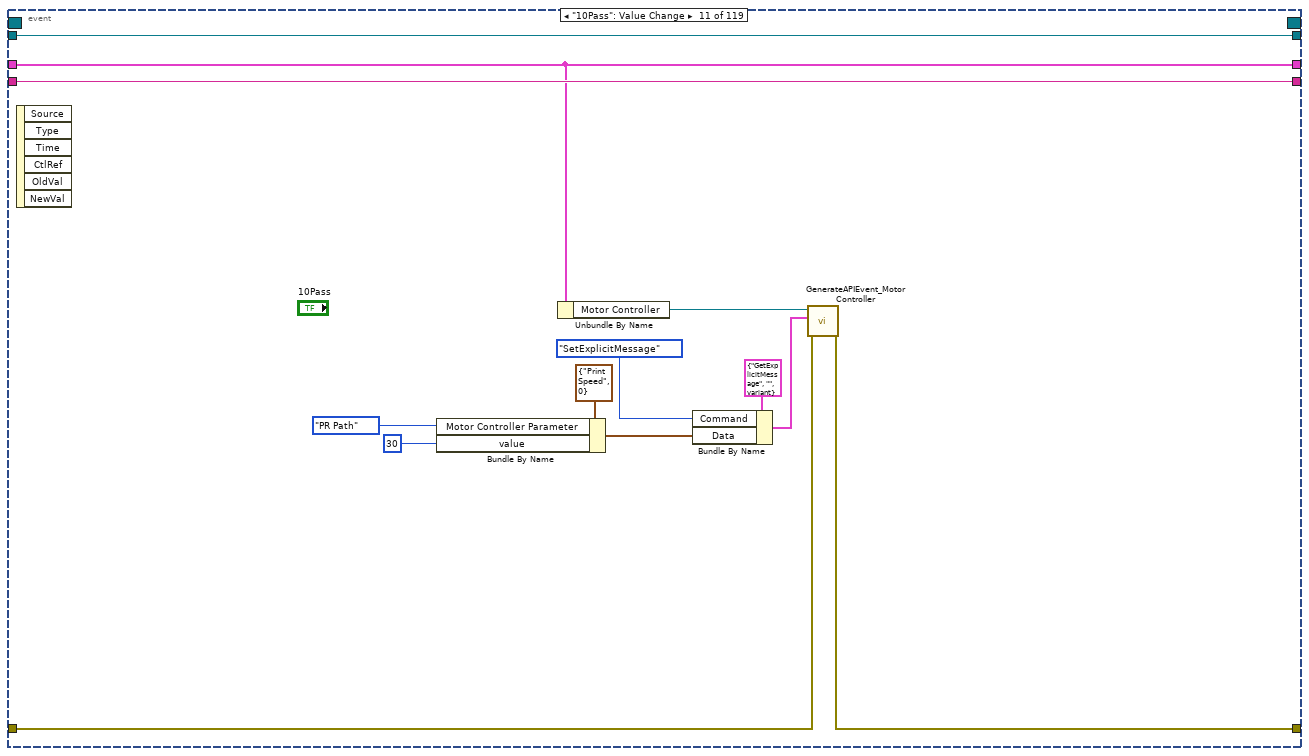
[diagram p14: hidden frame]
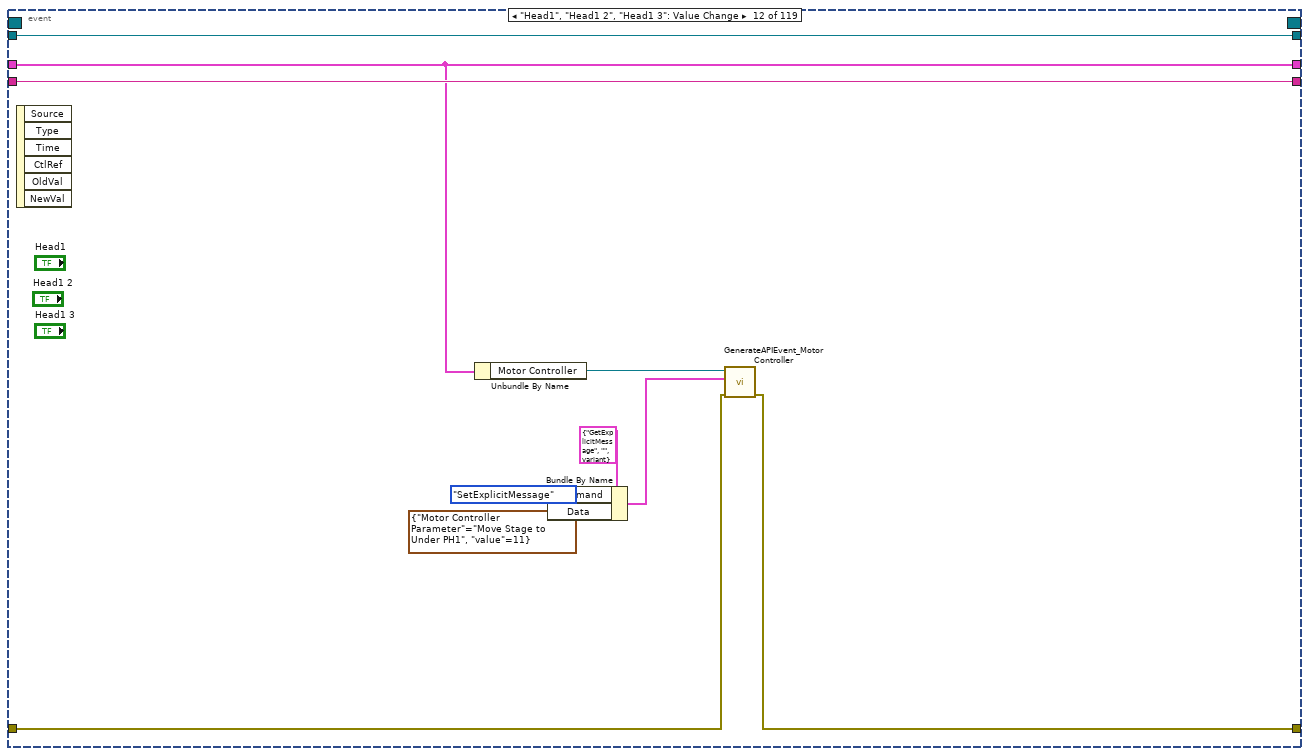
[diagram p15: hidden frame]
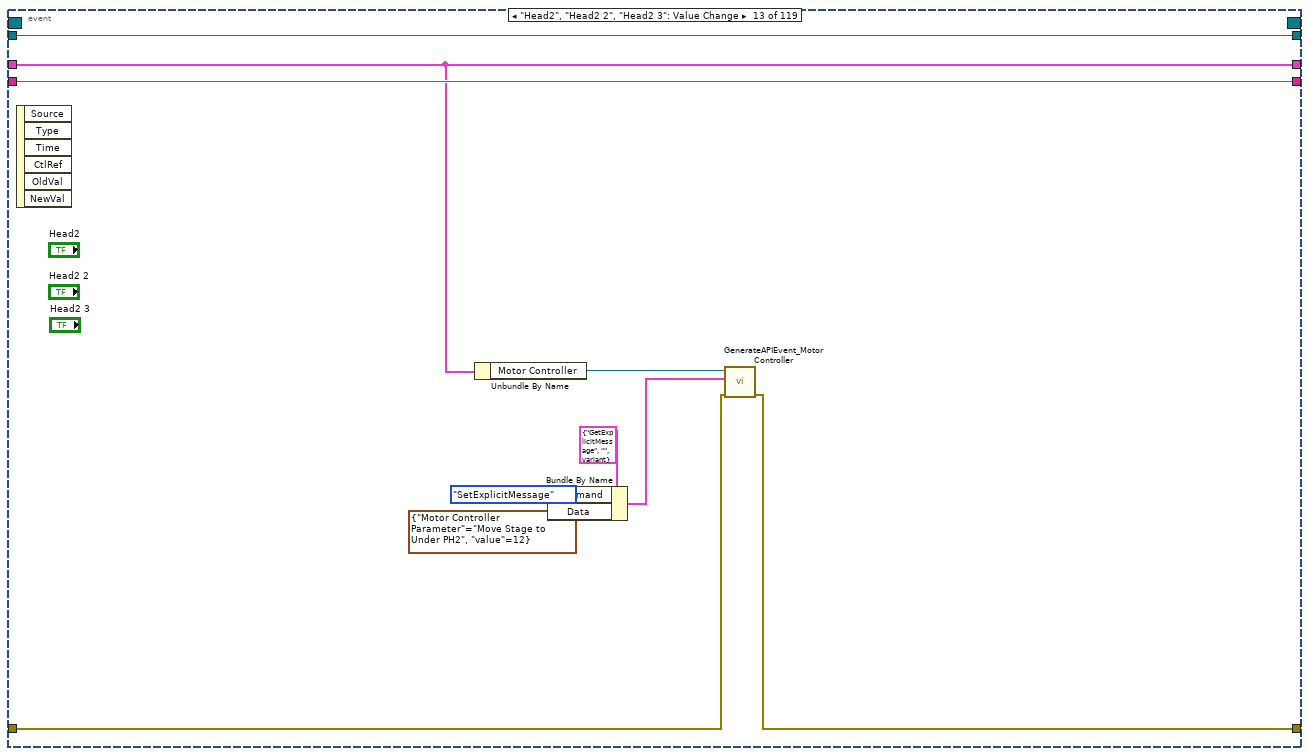
[diagram p16: hidden frame]
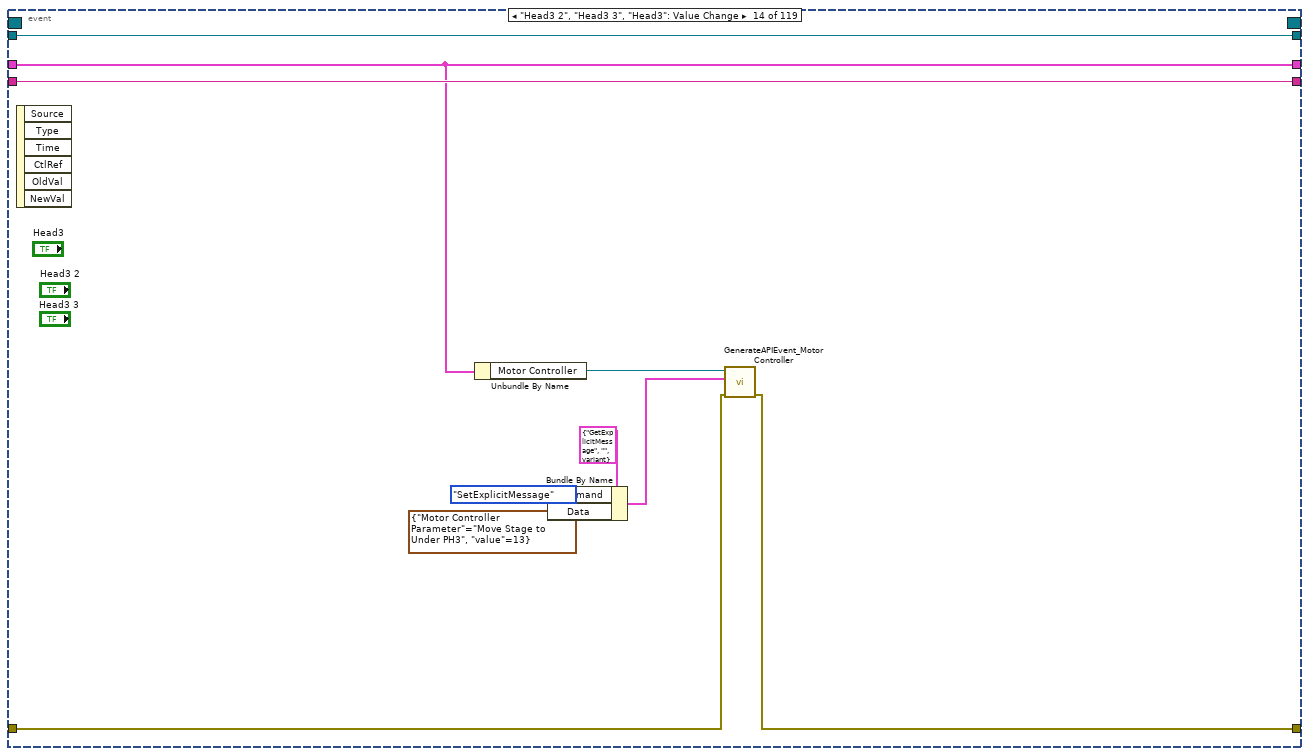
[diagram p17: hidden frame]
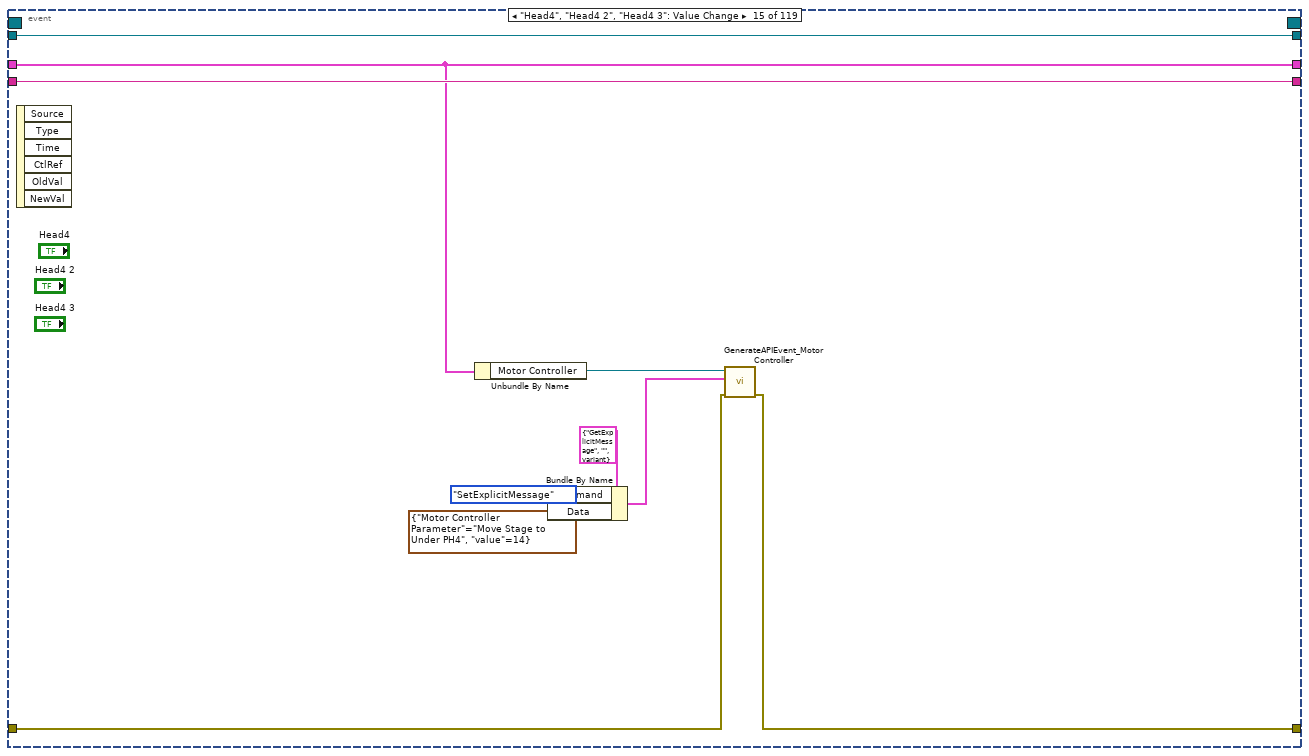
[diagram p18: hidden frame]
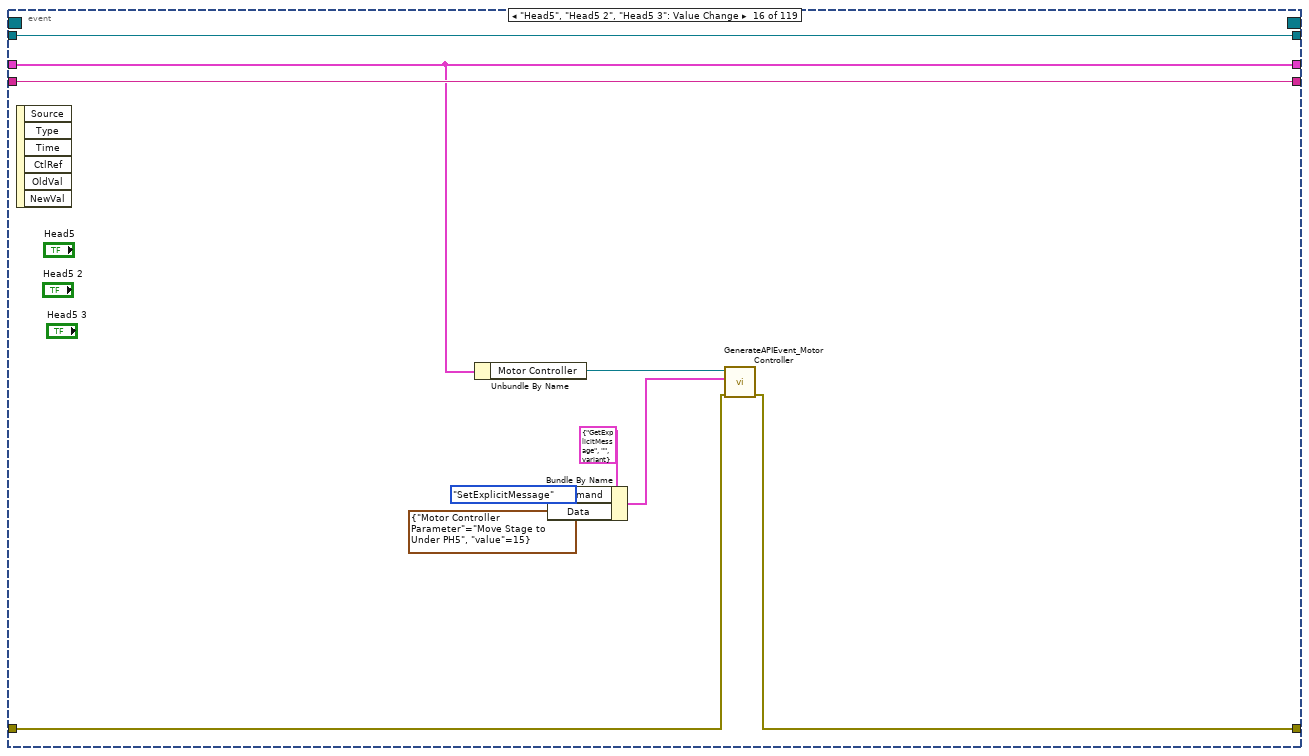
[diagram p19: hidden frame]
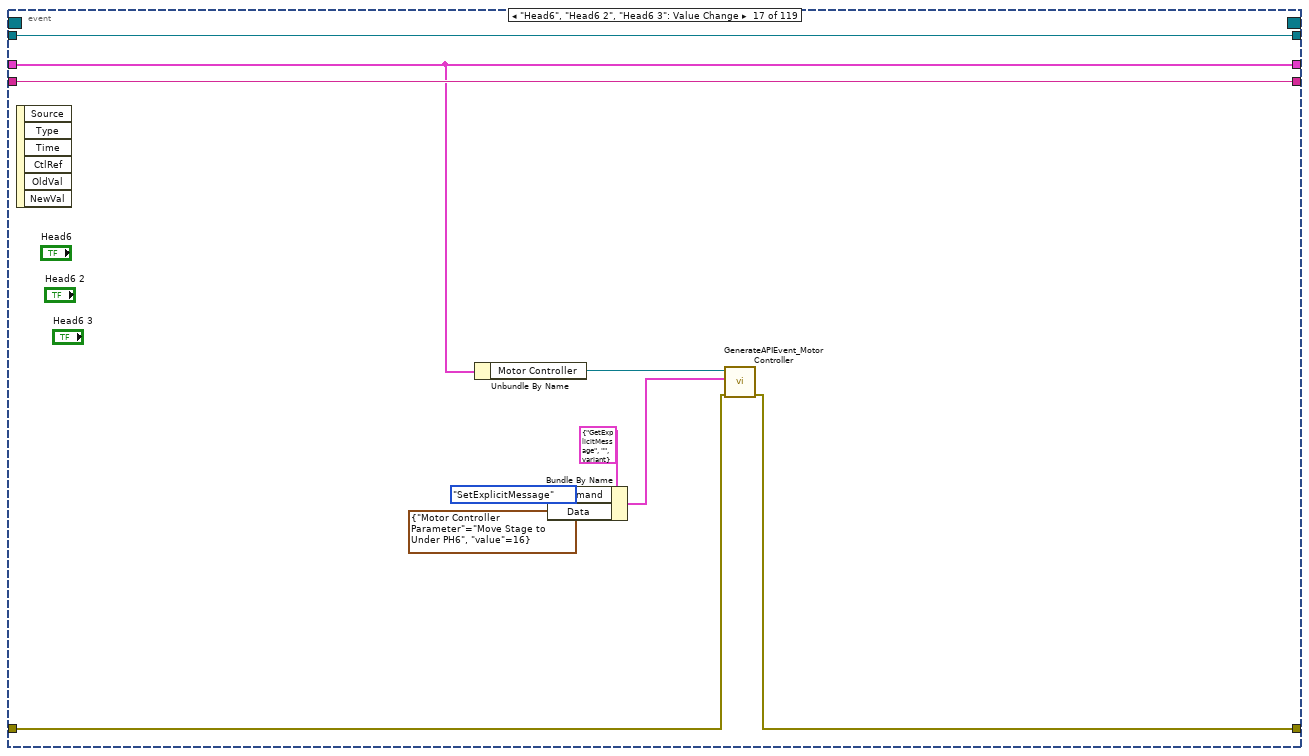
[diagram p20: hidden frame]
diagram:
  # "UI: SetUIControlsState>>disable"
  # "UI: SetUIControlsState>>enable"
  n1 = disable-structure shown="Enabled" {
    disable-tunnel: ["TopLevel In" w6] -> w2
    frame Disabled {
    }
    frame Enabled {
      n2 = call "Launcher.vi"() -> ("TopLevel out"=w6:refnum<class "TopLevel.lvclass">)  [unwired: 10 in, 1 out]
    }
  }
  n3 = call <vilib>:"Add State(s) to Queue__JKI_lib_State_Machine.vi"("State(s) in (\"\")"="Macro: Initialize") -> ("States Out"=w4:string)  [unwired: 14 in]
  n4 = while "JKI - String-Based Queued State Machine (Basic) v1.0" {
    shift-right: [w14] -> _
    shift-left: _ -> [w13]
    shift-right: [w17] -> _
    shift-left: _ -> [w11]
    shift-right: [w16] -> _
    shift-left: w4 -> [w18]
    tunnel: w2 -> [w10]
    tunnel: [w9] -> w1
    shift-right: [w8] -> _
    shift-left: _ -> [w7]
    stop <- w15 stop-if-true
    w12 = -1  # Timeout
    n5 = call <vilib>:"Parse State Queue__JKI_lib_State_Machine.vi"("State Queue"=w18, "Error In (no error)"=w11) -> ("Remaining States"=w20:string, "Current State"=w21:string, "Arguments"=w19:string)  [unwired: 11 in]
    n6 = case shown="\"\", \"Event Structure\", \"Idle\"" w21 {
      selector: w21 -> [_ _ w1324 _ _ _ _ _ _ _ _ _ _ _ _ _ _ _ _ _ _ _ _ _ _ _ _ _ _ _ _ _ _ _ _ _ _ _ _ _ _ _ _]
      tunnel: w20 -> [w31 w1321 w1328 w1348 w1356 w1363 w1369 w1395 w1403 w1409 w1431 w1457 w1465 w1478 w1515 w1521 w1528 w1544 w1549 w1576 w1582 w1587 w1601 w1603 w1618 w1630 w1658 w1687 w1722 w1733 w1755 w1777 w1793 w1804 w1832 w1872 w1894 w1910 w1921 w1925 w1938 w1942 w1953]
      tunnel: w19 -> [_ _ _ _ _ _ _ _ _ _ w1423 _ w1460 w1472 _ _ _ _ _ _ _ _ _ _ _ _ _ _ _ _ _ _ _ _ _ _ _ _ _ _ _ _ _]
      tunnel: w13 -> [w29 w1318 w1326 w1339 w1353 w1361 w1366 _ w1398 w1406 w1426 w1448 w1463 w1474 w1512 w1518 w1525 w1532 w1547 w1572 w1581 w1585 w1589 w1607 w1612 w1632 w1660 w1690 w1721 w1735 w1757 w1779 w1792 w1806 w1834 w1874 w1896 w1909 w1918 w1924 w1936 w1941 w1945]
      tunnel: [w28 w1319 w1330 w1345 errorcluster {"status"=FALSE, "code"=0, "source"=""} ("error out") w1360 w1367 w1377 w1399 w1407 w1429 w1453 w1461 w1475 w1508 w1519 w1526 w1531 w1548 w1554 w1578 w1586 w1588 w1604 w1609 w1631 w1659 w1689 w1723 w1734 w1756 w1778 w1794 w1805 w1833 w1873 w1895 w1911 w1916 w1926 w1933 w1943 w1949] -> w17
      tunnel: w11 -> [w27 w1319 w1329 w1345 w1352 w1360 w1367 w1376 w1400 w1407 w1429 w1452 w1462 w1476 w1502 w1519 w1526 w1530 w1548 w1571 w1577 w1586 w1591 w1604 w1608 w1624 w1655 w1681 w1723 w1730 w1749 w1771 w1794 w1799 w1827 w1867 w1889 w1911 w1915 w1926 w1932 w1943 w1948]
      tunnel: [w30 w1320 w1327 w1347 w1355 w1362 w1368 w1394 w1402 w1408 w1430 w1457 w1464 w1477 w1515 w1520 w1527 w1543 w1549 w1576 w1582 w1587 w1601 w1603 w1618 w1630 w1658 w1687 w1722 w1733 w1755 w1777 w1793 w1804 w1832 w1872 w1894 w1910 w1921 w1925 w1938 w1942 w1953] -> w16
      tunnel: [_ _ _ _ _ TRUE _ _ _ _ _ _ _ _ _ _ _ _ _ _ _ _ _ _ _ _ _ _ _ _ _ _ _ _ _ _ _ _ _ _ _ _ _] -> w15
      tunnel: [w26 w1318 w1326 w1346 w1353 w1361 w1366 w1393 w1398 w1406 w1426 w1448 w1463 w1474 w1512 w1518 w1525 w1532 w1547 w1572 w1581 w1585 w1589 w1607 w1612 w1632 w1660 w1690 w1721 w1735 w1757 w1779 w1792 w1806 w1834 w1874 w1896 w1909 w1918 w1924 w1936 w1941 w1945] -> w14
      tunnel: w12 -> [w25 _ _ _ _ _ _ _ _ _ _ _ _ _ _ _ _ _ _ _ _ _ _ _ _ _ _ _ _ _ _ _ _ _ _ _ _ _ _ _ _ _ _]
      tunnel: w10 -> [w24 w1317 w1323 w1336 w1350 w1358 w1365 w1391 w1397 w1405 w1428 w1456 w1459 w1471 w1514 w1517 w1523 w1535 w1546 w1575 w1580 w1584 w1592 w1606 w1620 w1634 w1662 w1692 w1720 w1737 w1759 w1781 w1791 w1808 w1836 w1876 w1898 w1908 w1920 w1923 w1934 w1940 w1950]
      tunnel: [w23 w1317 w1323 w1336 w1350 w1358 w1365 w1391 w1397 w1405 w1428 w1456 w1459 w1471 w1514 w1517 w1523 w1535 w1546 w1575 w1580 w1584 w1592 w1606 w1620 w1634 w1662 w1692 w1720 w1737 w1759 w1781 w1791 w1808 w1836 w1876 w1898 w1908 w1920 w1923 w1935 w1940 w1951] -> w9
      tunnel: [w22 w1316 w1322 w1335 w1349 w1357 w1364 w1381 w1396 w1404 w1427 w1455 w1458 w1470 w1513 w1516 w1522 w1536 w1545 w1570 w1579 w1583 w1600 w1605 w1619 w1633 w1661 w1691 w1719 w1736 w1758 w1780 w1790 w1807 w1835 w1875 w1897 w1907 w1919 w1922 w1937 w1939 w1952] -> w8
      tunnel: w7 -> [w22 w1316 w1322 w1335 w1349 w1357 w1364 w1381 w1396 w1404 w1427 w1455 w1458 w1470 w1513 w1516 w1522 w1536 w1545 _ w1579 w1583 w1600 w1605 w1619 w1633 w1661 w1691 w1719 w1736 w1758 w1780 w1790 w1807 w1835 w1875 w1897 w1907 w1919 w1922 w1937 w1939 w1952]
      frame "", "Event Structure", "Idle" {
        n7 = event shown="[1] <TopLevel StatusChanged Event>: User Event" {
          selector: w22 -> [_ _ _ _ _ _ _ w126 _ _ _ _ _ _ _ _ _ _ _ _ _ _ _ _ _ _ _ _ _ _ _ _ _ _ _ _ _ _ _ _ _ _ _ _ _ _ _ _ _ _ _ _ _ _ _ _ _ _ _ _ _ _ _ _ _ _ _ _ _ _ _ _ _ _ _ _ _ _ _ _ _ _ _ _ _ _ _ _ _ _ _ _ _ _ _ _ _ _ _ _ _ _ _ _ _ _ _ _ _ _ _ _ _ _ _ _ _ _ _]
          dyn-events: [_ _ _ _ _ _ _ w123 _ _ _ _ _ _ _ _ _ _ _ _ _ _ _ _ _ _ _ _ _ _ _ _ _ _ _ _ _ _ _ _ _ _ _ _ _ _ _ _ _ _ _ _ _ _ _ _ _ _ _ _ _ _ _ _ _ _ _ _ _ _ _ _ _ _ _ _ _ _ _ _ _ _ _ _ _ _ _ _ _ _ _ _ _ _ _ _ _ _ _ _ _ _ _ _ _ _ _ _ _ _ _ _ _ _ _ _ _ _ _] -> _
          timeout: w25 -> [_ _ _ _ _ _ _ _ _ _ _ _ _ _ _ _ _ _ _ _ _ _ _ _ _ _ _ _ _ _ _ _ _ _ _ _ _ _ _ _ _ _ _ _ _ _ _ _ _ _ _ _ _ _ _ _ _ _ _ _ _ _ _ _ _ _ _ _ _ _ _ _ _ _ _ _ _ _ _ _ _ _ _ _ _ _ _ _ _ _ _ _ _ _ _ _ _ _ _ _ _ _ _ _ _ _ _ _ _ _ _ _ _ _ _ _ _ _ _]
          tunnel: w31 -> [w36 w44 w61 w76 w83 w89 w92 w127 w143 w160 w173 w184 w194 w204 w214 w224 w234 w242 w255 w261 w295 w330 w346 w353 w366 w387 w403 w413 w423 w441 w447 w458 w469 w480 w491 w502 w515 w523 w531 w539 w547 w555 w559 w567 w575 w583 w591 w599 w608 w617 w626 w635 w644 w653 w672 w674 w711 w727 w743 w759 w775 w791 w807 w820 w833 w846 w859 w872 w874 w889 w897 w905 w913 w921 w929 w937 w945 w953 w961 w969 w977 w985 w993 w1001 w1009 w1017 w1025 w1033 w1041 w1049 w1057 w1065 w1073 w1081 w1089 w1097 w1105 w1113 w1121 w1149 w1171 w1179 w1187 w1195 w1203 w1211 w1219 w1227 w1235 w1243 w1251 w1259 w1267 w1275 w1283 w1291 w1299 w1307 w1315]
          tunnel: [w35 w43 w60 w75 w82 w88 w93 w128 w143 w160 w173 w184 w194 w204 w214 w224 w234 w242 w255 w261 w295 w330 w346 w353 w366 w387 w403 w413 w423 w441 w448 w459 w470 w481 w492 w503 w515 w523 w531 w539 w547 w555 w560 w568 w576 w584 w592 w600 w609 w618 w627 w636 w645 w654 w672 w675 w711 w727 w743 w759 w775 w791 w807 w820 w833 w846 w859 w872 w875 w889 w897 w905 w913 w921 w929 w937 w945 w953 w961 w969 w977 w985 w993 w1001 w1009 w1017 w1025 w1033 w1041 w1049 w1057 w1065 w1073 w1081 w1089 w1097 w1105 w1113 w1121 w1149 w1171 w1179 w1187 w1195 w1203 w1211 w1219 w1227 w1235 w1243 w1251 w1259 w1267 w1275 w1283 w1291 w1299 w1307 w1315] -> w30
          tunnel: w29 -> [w33 w41 w58 w73 w78 w85 w110 w130 w142 w159 w172 w178 w188 w198 w208 w218 w228 w239 w249 w258 w290 w328 w344 w351 w364 w385 w401 w411 w421 w435 w451 w462 w473 w484 w495 w506 w513 w521 w529 w537 w545 w553 w562 w570 w578 w586 w594 w602 w612 w621 w630 w639 w648 w657 w660 w677 w700 w716 w732 w748 w764 w780 w796 w809 w822 w835 w848 w861 w880 w886 w894 w902 w910 w918 w926 w934 w942 w950 w958 w966 w974 w982 w990 w998 w1006 w1014 w1022 w1030 w1038 w1046 w1054 w1062 w1070 w1078 w1086 w1094 w1102 w1110 w1118 w1146 w1169 w1176 w1184 w1192 w1200 w1208 w1216 w1225 w1233 w1241 w1249 w1257 w1265 w1273 w1281 w1289 w1297 w1305 w1313]
          tunnel: [w34 w42 w51 w69 w77 w84 w111 w122 w140 w157 w170 w176 w186 w196 w206 w216 w226 w238 w248 w257 w262 w318 w332 w348 w355 w375 w389 w409 w419 w428 w450 w461 w472 w483 w494 w505 w510 w518 w526 w534 w542 w550 w561 w569 w577 w585 w593 w601 w610 w619 w628 w637 w646 w655 w669 w684 w708 w724 w740 w756 w772 w788 w804 w817 w830 w843 w856 w869 w878 w883 w892 w900 w908 w916 w924 w932 w940 w948 w956 w964 w972 w980 w988 w996 w1004 w1012 w1020 w1028 w1036 w1044 w1052 w1060 w1068 w1076 w1084 w1092 w1100 w1108 w1116 w1133 w1166 w1174 w1182 w1190 w1198 w1206 w1214 w1223 w1231 w1239 w1247 w1255 w1263 w1271 w1279 w1287 w1295 w1303 w1311] -> w28
          tunnel: w27 -> [w34 w42 w45 w68 w77 w84 w111 w121 w139 w156 w169 w175 w185 w195 w205 w215 w225 w237 w247 w256 w277 w312 w336 w349 w356 w368 w393 w408 w418 w434 w450 w461 w472 w483 w494 w505 w509 w517 w525 w533 w541 w549 w561 w569 w577 w585 w593 w601 w610 w619 w628 w637 w646 w655 w668 w683 w707 w723 w739 w755 w771 w787 w803 w816 w829 w842 w855 w868 w877 w882 w891 w899 w907 w915 w923 w931 w939 w947 w955 w963 w971 w979 w987 w995 w1003 w1011 w1019 w1027 w1035 w1043 w1051 w1059 w1067 w1075 w1083 w1091 w1099 w1107 w1115 w1123 w1165 w1173 w1181 w1189 w1197 w1205 w1213 w1222 w1230 w1238 w1246 w1254 w1262 w1270 w1278 w1286 w1294 w1302 w1310]
          tunnel: [w33 w41 w58 w73 w78 w85 w99 w130 w142 w159 w172 w178 w188 w198 w208 w218 w228 w239 w249 w258 w290 w328 w344 w351 w364 w385 w401 w411 w421 w435 w449 w460 w471 w482 w493 w504 w513 w521 w529 w537 w545 w553 w557 w565 w573 w581 w589 w597 w606 w615 w624 w633 w642 w651 w660 w677 w700 w716 w732 w748 w764 w780 w796 w809 w822 w835 w848 w861 w880 w886 w894 w902 w910 w918 w926 w934 w942 w950 w958 w966 w974 w982 w990 w998 w1006 w1014 w1022 w1030 w1038 w1046 w1054 w1062 w1070 w1078 w1086 w1094 w1102 w1110 w1118 w1146 w1169 w1176 w1184 w1192 w1200 w1208 w1216 w1225 w1233 w1241 w1249 w1257 w1265 w1273 w1281 w1289 w1297 w1305 w1313] -> w26
          tunnel: w24 -> [w32 w40 w59 w74 w79 w86 w109 w129 w144 w161 w174 w183 w193 w203 w213 w223 w233 w241 w254 w260 w294 w329 w345 w352 w365 w386 w402 w412 w422 w440 w452 w463 w474 w485 w496 w507 w514 w522 w530 w538 w546 w554 w563 w571 w579 w587 w595 w603 w611 w620 w629 w638 w647 w656 w670 w685 w709 w725 w741 w757 w773 w789 w805 w818 w831 w844 w857 w870 w881 w887 w895 w903 w911 w919 w927 w935 w943 w951 w959 w967 w975 w983 w991 w999 w1007 w1015 w1023 w1031 w1039 w1047 w1055 w1063 w1071 w1079 w1087 w1095 w1103 w1111 w1119 w1147 w1170 w1177 w1185 w1193 w1201 w1209 w1217 w1226 w1234 w1242 w1250 w1258 w1266 w1274 w1282 w1290 w1298 w1306 w1314]
          tunnel: [w32 w40 w59 w74 w79 w86 w109 w129 w144 w161 w174 w183 w193 w203 w213 w223 w233 w241 w254 w260 w294 w329 w345 w352 w365 w386 w402 w412 w422 w440 w452 w463 w474 w485 w496 w507 w514 w522 w530 w538 w546 w554 w563 w571 w579 w587 w595 w603 w611 w620 w629 w638 w647 w656 w671 w686 w710 w726 w742 w758 w774 w790 w806 w819 w832 w845 w858 w871 w881 w887 w895 w903 w911 w919 w927 w935 w943 w951 w959 w967 w975 w983 w991 w999 w1007 w1015 w1023 w1031 w1039 w1047 w1055 w1063 w1071 w1079 w1087 w1095 w1103 w1111 w1119 w1147 w1170 w1177 w1185 w1193 w1201 w1209 w1217 w1226 w1234 w1242 w1250 w1258 w1266 w1274 w1282 w1290 w1298 w1306 w1314] -> w23
          event Timeout {
            n8 = event-data() -> ()  [unwired: 1 in, 1 out]
            n9 = call <vilib>:"Add State(s) to Queue__JKI_lib_State_Machine.vi"("State(s) in (\"\")"=w36) -> ("States Out"=w35:string)  [unwired: 14 in]
          }
          event User Event {
            n10 = event-data() -> ("PrintNo"=→"Print #":i32, "PrePurgePrintNo"=→"PrePrgPrint #":i32)  [unwired: 1 in, 7 out]
            n11 = call <vilib>:"Add State(s) to Queue__JKI_lib_State_Machine.vi"("State(s) in Front (\"\")"="UI: Update Stage Busy" ("State(s) in Front (\"\")"), "State(s) in (\"\")"=w44) -> ("States Out"=w43:string)  [unwired: 13 in]
          }
          event "Abort": Value Change {
            n12 = event-data() -> ()  [unwired: 1 in, 6 out]
            n13 = Unbundle By Name(w58) -> ("TopLevel out"=w47:refnum<class "TopLevel.lvclass">, "Motor Controller"=w55:refnum<class "Motor Controller.lvclass">, "GIS Printer"=w49:refnum<class "GIS Printer.lvclass">)
            n14 = call-dynamic "Abort API.vi"("error in (no error)"=w45, "TopLevel in"=w47) -> ("error out"=w46:errorcluster)  [unwired: 8 in, 1 out]
            n15 = call "Generate Abort Event GIS Printer.vi"("error in (no error)"=w46, "GIS Printer in"=w49) -> ("error out"=w50:errorcluster, "GIS Printer out"=w48:refnum<class "GIS Printer.lvclass">)  [unwired: 8 in]
            n16 = disable-structure shown="Disabled" {
              disable-tunnel: "AbortPrint" ("Task ID") -> [w66 _]
              disable-tunnel: FALSE ("Wait (F)") -> [w65 _]
              disable-tunnel: [w64 w67] -> w52
              disable-tunnel: w48 -> [w63 _]
              disable-tunnel: w50 -> [w62 w67]
              frame Disabled {
                n17 = call "API_Abort.vi"("Wait (F)"=w65, "error in (no error)"=w62, "Task ID"=w66, "GIS Printer in"=w63) -> ("error out"=w64:errorcluster)  [unwired: 5 in, 2 out]
              }
              frame Enabled {
              }
            }
            n18 = call "API_AbortStage.vi"("Wait (F)"=FALSE, "error in (no error)"=w52, "Task ID"="AbortMotor", "Motor Controller in"=w55) -> ("error out"=w51:errorcluster)  [unwired: 5 in, 2 out]
            n19 = call <vilib>:"Add State(s) to Queue__JKI_lib_State_Machine.vi"("State(s) in (\"\")"=w61) -> ("States Out"=w60:string)  [unwired: 14 in]
          }
          event "Stage Abort": Value Change {
            n20 = event-data() -> ()  [unwired: 1 in, 6 out]
            n21 = Unbundle By Name(w73) -> ("Motor Controller"=w72:refnum<class "Motor Controller.lvclass">)  [unwired: 1 out]
            n22 = call "API_AbortStage.vi"("Wait (F)"=FALSE, "error in (no error)"=w68, "Task ID"="AbortMotor", "Motor Controller in"=w72) -> ("error out"=w69:errorcluster)  [unwired: 5 in, 2 out]
            n23 = call <vilib>:"Add State(s) to Queue__JKI_lib_State_Machine.vi"("State(s) in (\"\")"=w76) -> ("States Out"=w75:string)  [unwired: 14 in]
          }
          event Panel Close? {
            # "Discard the event because we'll close the front panel ourselves in Macro: Exit"
            n24 = event-data() -> ()  [unwired: 1 in, 1 out]
            n25 = event-data("Discard?"=TRUE) -> ()  [unwired: 1 in, 1 out]
            n26 = call <vilib>:"Add State(s) to Queue__JKI_lib_State_Machine.vi"("State(s) in Front (\"\")"="Macro: Exit", "State(s) in (\"\")"=w83) -> ("States Out"=w82:string)  [unwired: 13 in]
          }
          event "Exit": Value Change {
            n27 = event-data() -> ()  [unwired: 1 in, 6 out]
            n28 = call <vilib>:"Add State(s) to Queue__JKI_lib_State_Machine.vi"("State(s) in Front (\"\")"="Macro: Exit", "State(s) in (\"\")"=w89) -> ("States Out"=w88:string)  [unwired: 13 in]
          }
          event User Event {
            n29 = event-data() -> ("Motor Controller Config Data"=w98:T18, "Motor Controller Data"=w97:cluster{"Enabled?":bool}, "Stage Move.Current Step"=→"Status":string, "Stage Move.Move Data"=w96:T20[], "Stage Busy?"=w90:bool)  [unwired: 1 in, 4 out]
            n30 = flat-sequence {
              tunnel: w90 -> [_]
              frame #0 {
              }
            }
            n31 = Unbundle By Name(w98) -> ("Current Position"=→"Position":i32, "Pulse_Per_mm"=→"Pulse/mm":i32, "PrePrint"=w106:dbl[])
            n32 = Unbundle By Name(w97) -> ()  [unwired: 1 out]
            n33 = Bundle By Name(cluster=w110, "Status.Motor Controller Config Data"=w98, "Status.Motor Controller Data"=w97) -> (w99:T36)
            n34 = for {
              tunnel: w96 -> [w119] mode=indexing
              tunnel: [w112] -> w94 mode=indexing
              n35 = Unbundle By Name(w119) -> ("Move.Index_mm"=w118:i32, "Move.Speed_mm_s"=w117:i32, "Status"=w114:T21)
              n36 = Format Into String(w118) -> (resulting string=w116:string)  [unwired: 3 in, 1 out]
              n37 = Format Into String(w117) -> (resulting string=w115:string)  [unwired: 3 in, 1 out]
              n38 = Format Into String(w114) -> (resulting string=w113:string)  [unwired: 3 in, 1 out]
              n39 = Build Array(w116, w115, w113) -> (w112:string[])
            }
            n40 = Index Array(array=w106) -> (element #1=→"H1":dbl, element #2=→"H 2":dbl, element #3=→"H 3":dbl, element #4=→"H 4":dbl, element #5=→"H 5":dbl, element #6=→"H 6":dbl)  [unwired: 6 in]
            n41 = property on="Stage Move Status" class="MCListbox (strict)"("ItemNames"=w94) -> ()  [unwired: 2 in, 2 out]
            n42 = call <vilib>:"Add State(s) to Queue__JKI_lib_State_Machine.vi"("State(s) in Front (\"\")"="UI: Update Stage Busy", "State(s) in (\"\")"=w92) -> ("States Out"=w93:string)  [unwired: 13 in]
          }
          event User Event {
            n43 = event-data() -> ("UsrEvtRef"=w125:refnum<user-event>)  [unwired: 1 in, 3 out]
            n44 = Flush Event Queue(0:w126, 2:w125, 3:w121, 5:1 ("keep most recent")) -> (8:w123:refnum<event-registration>, 11:w122:errorcluster)  [unwired: 2 in, 1 out]
            n45 = call <vilib>:"Add State(s) to Queue__JKI_lib_State_Machine.vi"("State(s) in Front (\"\")"="DI: Get ICP2 DI Status\nDO: Set ICP1-DO Status in UI\nDO: Set ICP2-DO Status in UI\nAI: Get ICP1 AI Status\nAO: Set ICP1-AO Status in UI\nAO: Set ICP2-AO Status in UI" ("State(s) in Front (\"\")"), "State(s) in (\"\")"=w127) -> ("States Out"=w128:string)  [unwired: 13 in]
          }
          event "Enable Disable": Value Change {
            n46 = event-data() -> ()  [unwired: 1 in, 6 out]
            n47 = case shown="True" "Enable Disable" {
              tunnel: [Motor_Controller_Parameter-Set."Enable Servo" ("Motor Controller Parameter") Motor_Controller_Parameter-Set."Disable Servo" ("Motor Controller Parameter")] -> w134
              tunnel: [1 ("value") 0 ("value")] -> w131
              frame True {
              }
              frame False {
              }
            }
            n48 = Bundle By Name(cluster=T3 {"Motor Controller Parameter"=enum."Print Speed", "value"=0} ("SetExplicitMessage API Data"), "Motor Controller Parameter"=w134, "value"=w131) -> (w133:T3)
            n49 = Unbundle By Name(w142) -> ("Motor Controller"=w141:refnum<class "Motor Controller.lvclass">)
            n50 = Bundle By Name(cluster=T6 {"Command"=enum."GetExplicitMessage", "Arguments"="", "Data"=variant} ("API Command Cluster"), "Command"=API_Command_Enum."SetExplicitMessage", "Data"=w133) -> (w132:T6)
            n51 = call-dynamic "GenerateAPIEvent_Motor Controller.vi"("error in (no error)"=w139, "API Command Cluster"=w132, "Motor Controller In"=w141) -> ("error out"=w140:errorcluster)  [unwired: 6 in, 2 out]
          }
          event "5Pass": Value Change {
            n52 = event-data() -> ()  [unwired: 1 in, 6 out]
            n53 = Bundle By Name(cluster=T3 {"Motor Controller Parameter"=enum."Print Speed", "value"=0} ("SetExplicitMessage API Data"), "Motor Controller Parameter"=Motor_Controller_Parameter-Set."PR Path", "value"=20) -> (w151:T3)
            n54 = Unbundle By Name(w159) -> ("Motor Controller"=w158:refnum<class "Motor Controller.lvclass">)
            n55 = Bundle By Name(cluster=T6 {"Command"=enum."GetExplicitMessage", "Arguments"="", "Data"=variant} ("API Command Cluster"), "Command"=API_Command_Enum."SetExplicitMessage", "Data"=w151) -> (w150:T6)
            n56 = call-dynamic "GenerateAPIEvent_Motor Controller.vi"("error in (no error)"=w156, "API Command Cluster"=w150, "Motor Controller In"=w158) -> ("error out"=w157:errorcluster)  [unwired: 6 in, 2 out]
          }
          event "10Pass": Value Change {
            n57 = event-data() -> ()  [unwired: 1 in, 6 out]
            n58 = Bundle By Name(cluster=T3 {"Motor Controller Parameter"=enum."Print Speed", "value"=0} ("SetExplicitMessage API Data"), "Motor Controller Parameter"=Motor_Controller_Parameter-Set."PR Path", "value"=30) -> (w164:T3)
            n59 = Unbundle By Name(w172) -> ("Motor Controller"=w171:refnum<class "Motor Controller.lvclass">)
            n60 = Bundle By Name(cluster=T6 {"Command"=enum."GetExplicitMessage", "Arguments"="", "Data"=variant} ("API Command Cluster"), "Command"=API_Command_Enum."SetExplicitMessage", "Data"=w164) -> (w163:T6)
            n61 = call-dynamic "GenerateAPIEvent_Motor Controller.vi"("error in (no error)"=w169, "API Command Cluster"=w163, "Motor Controller In"=w171) -> ("error out"=w170:errorcluster)  [unwired: 6 in, 2 out]
          }
          event "Head1", "Head1 2", "Head1 3": Value Change {
            n62 = event-data() -> ()  [unwired: 1 in, 6 out]
            n63 = Unbundle By Name(w178) -> ("Motor Controller"=w182:refnum<class "Motor Controller.lvclass">)
            n64 = Bundle By Name(cluster=T6 {"Command"=enum."GetExplicitMessage", "Arguments"="", "Data"=variant} ("API Command Cluster"), "Command"=API_Command_Enum."SetExplicitMessage", "Data"=T3 {"Motor Controller Parameter"=enum."Move Stage to Under PH1", "value"=11} ("SetExplicitMessage API Data")) -> (w179:T6)
            n65 = call-dynamic "GenerateAPIEvent_Motor Controller.vi"("error in (no error)"=w175, "API Command Cluster"=w179, "Motor Controller In"=w182) -> ("error out"=w176:errorcluster)  [unwired: 6 in, 2 out]
          }
          event "Head2", "Head2 2", "Head2 3": Value Change {
            n66 = event-data() -> ()  [unwired: 1 in, 6 out]
            n67 = Unbundle By Name(w188) -> ("Motor Controller"=w192:refnum<class "Motor Controller.lvclass">)
            n68 = Bundle By Name(cluster=T6 {"Command"=enum."GetExplicitMessage", "Arguments"="", "Data"=variant} ("API Command Cluster"), "Command"=API_Command_Enum."SetExplicitMessage", "Data"=T3 {"Motor Controller Parameter"=enum."Move Stage to Under PH2", "value"=12} ("SetExplicitMessage API Data")) -> (w189:T6)
            n69 = call-dynamic "GenerateAPIEvent_Motor Controller.vi"("error in (no error)"=w185, "API Command Cluster"=w189, "Motor Controller In"=w192) -> ("error out"=w186:errorcluster)  [unwired: 6 in, 2 out]
          }
          event "Head3 2", "Head3 3", "Head3": Value Change {
            n70 = event-data() -> ()  [unwired: 1 in, 6 out]
            n71 = Unbundle By Name(w198) -> ("Motor Controller"=w202:refnum<class "Motor Controller.lvclass">)
            n72 = Bundle By Name(cluster=T6 {"Command"=enum."GetExplicitMessage", "Arguments"="", "Data"=variant} ("API Command Cluster"), "Command"=API_Command_Enum."SetExplicitMessage", "Data"=T3 {"Motor Controller Parameter"=enum."Move Stage to Under PH3", "value"=13} ("SetExplicitMessage API Data")) -> (w199:T6)
            n73 = call-dynamic "GenerateAPIEvent_Motor Controller.vi"("error in (no error)"=w195, "API Command Cluster"=w199, "Motor Controller In"=w202) -> ("error out"=w196:errorcluster)  [unwired: 6 in, 2 out]
          }
          event "Head4", "Head4 2", "Head4 3": Value Change {
            n74 = event-data() -> ()  [unwired: 1 in, 6 out]
            n75 = Unbundle By Name(w208) -> ("Motor Controller"=w212:refnum<class "Motor Controller.lvclass">)
            n76 = Bundle By Name(cluster=T6 {"Command"=enum."GetExplicitMessage", "Arguments"="", "Data"=variant} ("API Command Cluster"), "Command"=API_Command_Enum."SetExplicitMessage", "Data"=T3 {"Motor Controller Parameter"=enum."Move Stage to Under PH4", "value"=14} ("SetExplicitMessage API Data")) -> (w209:T6)
            n77 = call-dynamic "GenerateAPIEvent_Motor Controller.vi"("error in (no error)"=w205, "API Command Cluster"=w209, "Motor Controller In"=w212) -> ("error out"=w206:errorcluster)  [unwired: 6 in, 2 out]
          }
          event "Head5", "Head5 2", "Head5 3": Value Change {
            n78 = event-data() -> ()  [unwired: 1 in, 6 out]
            n79 = Unbundle By Name(w218) -> ("Motor Controller"=w222:refnum<class "Motor Controller.lvclass">)
            n80 = Bundle By Name(cluster=T6 {"Command"=enum."GetExplicitMessage", "Arguments"="", "Data"=variant} ("API Command Cluster"), "Command"=API_Command_Enum."SetExplicitMessage", "Data"=T3 {"Motor Controller Parameter"=enum."Move Stage to Under PH5", "value"=15} ("SetExplicitMessage API Data")) -> (w219:T6)
            n81 = call-dynamic "GenerateAPIEvent_Motor Controller.vi"("error in (no error)"=w215, "API Command Cluster"=w219, "Motor Controller In"=w222) -> ("error out"=w216:errorcluster)  [unwired: 6 in, 2 out]
          }
          event "Head6", "Head6 2", "Head6 3": Value Change {
            n82 = event-data() -> ()  [unwired: 1 in, 6 out]
            n83 = Unbundle By Name(w228) -> ("Motor Controller"=w232:refnum<class "Motor Controller.lvclass">)
            n84 = Bundle By Name(cluster=T6 {"Command"=enum."GetExplicitMessage", "Arguments"="", "Data"=variant} ("API Command Cluster"), "Command"=API_Command_Enum."SetExplicitMessage", "Data"=T3 {"Motor Controller Parameter"=enum."Move Stage to Under PH6", "value"=16} ("SetExplicitMessage API Data")) -> (w229:T6)
            n85 = call-dynamic "GenerateAPIEvent_Motor Controller.vi"("error in (no error)"=w225, "API Command Cluster"=w229, "Motor Controller In"=w232) -> ("error out"=w226:errorcluster)  [unwired: 6 in, 2 out]
          }
          event "Home", "Home 2", "Home 3": Value Change {
            n86 = event-data() -> ()  [unwired: 1 in, 6 out]
            n87 = Unbundle By Name(w239) -> ("Motor Controller"=w240:refnum<class "Motor Controller.lvclass">)
            n88 = call "API_HomeStage.vi"("Timeout (ms)"=u32 600000, "Wait (F)"=FALSE, "error in (no error)"=w237, "Motor Controller in"=w240) -> ("error out"=w238:errorcluster)  [unwired: 5 in, 2 out]
          }
          event "Load": Value Change {
            n89 = event-data() -> ()  [unwired: 1 in, 6 out]
            n90 = Unbundle By Name(w249) -> ("Motor Controller"=w253:refnum<class "Motor Controller.lvclass">)  [unwired: 1 out]
            n91 = Bundle By Name(cluster=T3 {"Motor Controller Parameter"=enum."Write Speed", "value"=0} ("SetExplicitMessage API Data"), "Motor Controller Parameter"=Motor_Controller_Parameter-Set."Return Stage to 0", "value"=0) -> (w244:T3)
            n92 = Bundle By Name(cluster=T6 {"Command"=enum."GetExplicitMessage", "Arguments"="", "Data"=variant} ("API Command Cluster"), "Command"=API_Command_Enum."SetExplicitMessage", "Data"=w244) -> (w250:T6)
            n93 = call-dynamic "GenerateAPIEvent_Motor Controller.vi"("error in (no error)"=w247, "API Command Cluster"=w250, "Motor Controller In"=w253) -> ("error out"=w248:errorcluster)  [unwired: 6 in, 2 out]
          }
          event "Laminate": Value Change {
            n94 = event-data() -> ()  [unwired: 1 in, 6 out]
            n95 = Unbundle By Name(w258) -> ("Motor Controller"=w259:refnum<class "Motor Controller.lvclass">)  [unwired: 1 out]
            n96 = call "Laminate API.vi"("error in (no error)"=w256, "Motor Controller in"=w259) -> ("error out"=w257:errorcluster)  [unwired: 7 in, 2 out]
          }
          event "Go": Value Change {
            # "Conversion done in SendLVEthIP_ExplicitMessage.vi"
            n97 = event-data() -> ()  [unwired: 1 in, 6 out]
            n98 = Unbundle By Name(w290) -> ("Motor Controller"=w280:refnum<class "Motor Controller.lvclass">)
            n99 = disable-structure shown="Enabled" {
              disable-tunnel: "Speed" -> [w304 w309]
              disable-tunnel: [w303 w309] -> w274
              frame Disabled {
                n100 = Multiply(x=w304, y=60 ("x")) -> (x*y=w308:i32)
                n101 = Divide(x=w308, y=12.7) -> (x/y=w306:dbl)
                n102 = To Long Integer(number=w306) -> (32bit integer=w303:i32)
              }
              frame Enabled {
              }
            }
            n103 = local write "Go"(FALSE ("Go To")) -> ()
            n104 = Bundle By Name(cluster=T3 {"Motor Controller Parameter"=enum."Write Speed", "value"=0} ("SetExplicitMessage API Data"), "Motor Controller Parameter"=Motor_Controller_Parameter-Set."Write Speed", "value"=w274) -> (w286:T3)
            n105 = Bundle By Name(cluster=T6 {"Command"=enum."GetExplicitMessage", "Arguments"="", "Data"=variant} ("API Command Cluster"), "Command"=API_Command_Enum."SetExplicitMessage", "Data"=w286) -> (w283:T6)
            n106 = disable-structure shown="Disabled" {
              disable-tunnel: [w298 w302] -> w273
              disable-tunnel: "GoTo" -> [w296 w302]
              frame Disabled {
                n107 = Divide(x=w296, y=12.7) -> (x/y=w301:dbl)
                n108 = Multiply(x=w301, y=100000.0 ("x")) -> (x*y=w299:dbl)
                n109 = To Long Integer(number=w299) -> (32bit integer=w298:i32)
              }
              frame Enabled {
              }
            }
            n110 = call-dynamic "GenerateAPIEvent_Motor Controller.vi"("error in (no error)"=w277, "API Command Cluster"=w283, "Motor Controller In"=w280) -> ("error out"=w278:errorcluster, "Motor Controller out"=w279:refnum<class "Motor Controller.lvclass">)  [unwired: 6 in, 1 out]
            n111 = Bundle By Name(cluster=T3 {"Motor Controller Parameter"=enum."Write Speed", "value"=0} ("SetExplicitMessage API Data"), "Motor Controller Parameter"=Motor_Controller_Parameter-Set."Write Index", "value"=w273) -> (w287:T3)
            n112 = Bundle By Name(cluster=T3 {"Motor Controller Parameter"=enum."Write Speed", "value"=0} ("SetExplicitMessage API Data"), "Motor Controller Parameter"=Motor_Controller_Parameter-Set."PR Path", "value"=10) -> (w271:T3)
            n113 = Bundle By Name(cluster=T6 {"Command"=enum."GetExplicitMessage", "Arguments"="", "Data"=variant} ("API Command Cluster"), "Command"=API_Command_Enum."SetExplicitMessage", "Data"=w287) -> (w291:T6)
            n114 = call-dynamic "GenerateAPIEvent_Motor Controller.vi"("error in (no error)"=w278, "API Command Cluster"=w291, "Motor Controller In"=w279) -> ("error out"=w263:errorcluster, "Motor Controller out"=w264:refnum<class "Motor Controller.lvclass">)  [unwired: 6 in, 1 out]
            n115 = Bundle By Name(cluster=T6 {"Command"=enum."GetExplicitMessage", "Arguments"="", "Data"=variant} ("API Command Cluster"), "Command"=API_Command_Enum."SetExplicitMessage", "Data"=w271) -> (w268:T6)
            n116 = call-dynamic "GenerateAPIEvent_Motor Controller.vi"("error in (no error)"=w263, "API Command Cluster"=w268, "Motor Controller In"=w264) -> ("error out"=w262:errorcluster)  [unwired: 6 in, 2 out]
          }
          event "Jog (+)", "Jog (+) 2", "Jog (+) 3": Value Change {
            n117 = event-data() -> ("NewVal"=w310:bool)  [unwired: 1 in, 5 out]
            n118 = Unbundle By Name(w328) -> ("Motor Controller"=w317:refnum<class "Motor Controller.lvclass">)
            n119 = property on="Jog Speed" class="DigNum (strict)"(error in=w312) -> (error out=w313:errorcluster, "Value"=w311:i32)  [unwired: 1 in, 1 out]
            n120 = Select(t=4998, s=w310, f=0) -> (s? t:f=w319:i32)
            n121 = call "SetJogSpeed.vi"("Timeout (ms)"=u32 1000, "error in (no error)"=w313, "Jog Speed"=w311, "Motor Controller in"=w317) -> ("error out"=w314:errorcluster, "Motor Controller out"=w316:refnum<class "Motor Controller.lvclass">)  [unwired: 6 in]
            n122 = Bundle By Name(cluster=T3 {"Motor Controller Parameter"=enum."Write Speed", "value"=0} ("SetExplicitMessage API Data"), "Motor Controller Parameter"=Motor_Controller_Parameter-Set."Jog Speed", "value"=w319) -> (w327:T3)
            n123 = Bundle By Name(cluster=T6 {"Command"=enum."GetExplicitMessage", "Arguments"="", "Data"=variant} ("API Command Cluster"), "Command"=API_Command_Enum."SetExplicitMessage", "Data"=w327) -> (w324:T6)
            n124 = call-dynamic "GenerateAPIEvent_Motor Controller.vi"("error in (no error)"=w314, "API Command Cluster"=w324, "Motor Controller In"=w316) -> ("error out"=w318:errorcluster)  [unwired: 6 in, 2 out]
          }
          event "Print (+)": Value Change {
            n125 = event-data() -> ()  [unwired: 1 in, 6 out]
            n126 = Select(t=4998, s="Print (+)", f=0) -> (s? t:f=w333:i32)
            n127 = Unbundle By Name(w344) -> ("Motor Controller"=w337:refnum<class "Motor Controller.lvclass">)
            n128 = Bundle By Name(cluster=T3 {"Motor Controller Parameter"=enum."Write Speed", "value"=0} ("SetExplicitMessage API Data"), "Motor Controller Parameter"=Motor_Controller_Parameter-Set."Write Speed", "value"=w333) -> (w343:T3)
            n129 = local write "Print Speed"(w333) -> ()
            n130 = Bundle By Name(cluster=T6 {"Command"=enum."GetExplicitMessage", "Arguments"="", "Data"=variant} ("API Command Cluster"), "Command"=API_Command_Enum."SetExplicitMessage", "Data"=w343) -> (w340:T6)
            n131 = call-dynamic "GenerateAPIEvent_Motor Controller.vi"("error in (no error)"=w336, "API Command Cluster"=w340, "Motor Controller In"=w337) -> ("error out"=w332:errorcluster)  [unwired: 6 in, 2 out]
          }
          event "Jog Speed": Value Change {
            n132 = event-data() -> ()  [unwired: 1 in, 6 out]
            n133 = Unbundle By Name(w351) -> ("Motor Controller"=w350:refnum<class "Motor Controller.lvclass">)
            n134 = call "SetJogSpeed.vi"("error in (no error)"=w349, "Jog Speed"="Jog Speed", "Motor Controller in"=w350) -> ("error out"=w348:errorcluster)  [unwired: 7 in, 1 out]
          }
          event "Print Speed": Value Change {
            n135 = event-data() -> ()  [unwired: 1 in, 6 out]
            n136 = Unbundle By Name(w364) -> ("Motor Controller"=w357:refnum<class "Motor Controller.lvclass">)
            n137 = Bundle By Name(cluster=T3 {"Motor Controller Parameter"=enum."Write Speed", "value"=0} ("SetExplicitMessage API Data"), "Motor Controller Parameter"=Motor_Controller_Parameter-Set."Write Speed", "value"="Print Speed") -> (w363:T3)
            n138 = Bundle By Name(cluster=T6 {"Command"=enum."GetExplicitMessage", "Arguments"="", "Data"=variant} ("API Command Cluster"), "Command"=API_Command_Enum."SetExplicitMessage", "Data"=w363) -> (w360:T6)
            n139 = call-dynamic "GenerateAPIEvent_Motor Controller.vi"("error in (no error)"=w356, "API Command Cluster"=w360, "Motor Controller In"=w357) -> ("error out"=w355:errorcluster)  [unwired: 6 in, 2 out]
          }
          event "Jog (-)", "Jog (-) 2", "Jog (-) 3": Value Change {
            n140 = event-data() -> ("NewVal"=w367:bool)  [unwired: 1 in, 5 out]
            n141 = property on="Jog Speed" class="DigNum (strict)"(error in=w368) -> (error out=w374:errorcluster, "Value"=w373:i32)  [unwired: 1 in, 1 out]
            n142 = Unbundle By Name(w385) -> ("Motor Controller"=w371:refnum<class "Motor Controller.lvclass">)
            n143 = Select(t=4999, s=w367, f=0) -> (s? t:f=w376:i32)
            n144 = call "SetJogSpeed.vi"("Timeout (ms)"=u32 1000, "error in (no error)"=w374, "Jog Speed"=w373, "Motor Controller in"=w371) -> ("error out"=w369:errorcluster, "Motor Controller out"=w370:refnum<class "Motor Controller.lvclass">)  [unwired: 6 in]
            n145 = Bundle By Name(cluster=T3 {"Motor Controller Parameter"=enum."Write Speed", "value"=0} ("SetExplicitMessage API Data"), "Motor Controller Parameter"=Motor_Controller_Parameter-Set."Jog Speed", "value"=w376) -> (w384:T3)
            n146 = Bundle By Name(cluster=T6 {"Command"=enum."GetExplicitMessage", "Arguments"="", "Data"=variant} ("API Command Cluster"), "Command"=API_Command_Enum."SetExplicitMessage", "Data"=w384) -> (w381:T6)
            n147 = call-dynamic "GenerateAPIEvent_Motor Controller.vi"("error in (no error)"=w369, "API Command Cluster"=w381, "Motor Controller In"=w370) -> ("error out"=w375:errorcluster)  [unwired: 6 in, 2 out]
          }
          event "Print (-)": Value Change {
            n148 = event-data() -> ()  [unwired: 1 in, 6 out]
            n149 = Select(t=4999, s="Print (-)", f=0) -> (s? t:f=w390:i32)
            n150 = Unbundle By Name(w401) -> ("Motor Controller"=w394:refnum<class "Motor Controller.lvclass">)
            n151 = local write "Print Speed"(w390) -> ()
            n152 = Bundle By Name(cluster=T3 {"Motor Controller Parameter"=enum."Write Speed", "value"=0} ("SetExplicitMessage API Data"), "Motor Controller Parameter"=Motor_Controller_Parameter-Set."Write Speed", "value"=w390) -> (w400:T3)
            n153 = Bundle By Name(cluster=T6 {"Command"=enum."GetExplicitMessage", "Arguments"="", "Data"=variant} ("API Command Cluster"), "Command"=API_Command_Enum."SetExplicitMessage", "Data"=w400) -> (w397:T6)
            n154 = call-dynamic "GenerateAPIEvent_Motor Controller.vi"("error in (no error)"=w393, "API Command Cluster"=w397, "Motor Controller In"=w394) -> ("error out"=w389:errorcluster)  [unwired: 6 in, 2 out]
          }
          event "Start": Value Change {
            n155 = event-data() -> ()  [unwired: 1 in, 6 out]
            n156 = Unbundle By Name(w411) -> ("Motor Controller"=w410:refnum<class "Motor Controller.lvclass">)
            n157 = Bundle By Name(cluster=T6 {"Command"=enum."GetExplicitMessage", "Arguments"="", "Data"=variant} ("API Command Cluster"), "Command"=API_Command_Enum."Execute Stage Move Recipe", "Data"="Stage Recipe XML File Path") -> (w406:T6)
            n158 = call-dynamic "GenerateAPIEvent_Motor Controller.vi"("error in (no error)"=w408, "API Command Cluster"=w406, "Motor Controller In"=w410) -> ("error out"=w409:errorcluster)  [unwired: 6 in, 2 out]
          }
          event "Stage Recipe XML File Path": Value Change {
            n159 = event-data() -> ("NewVal"=w414:path)  [unwired: 1 in, 5 out]
            n160 = Unbundle By Name(w421) -> ("Motor Controller"=w420:refnum<class "Motor Controller.lvclass">)
            n161 = Bundle By Name(cluster=T6 {"Command"=enum."GetExplicitMessage", "Arguments"="", "Data"=variant} ("API Command Cluster"), "Command"=API_Command_Enum."Read Stage Move Recipe", "Data"=w414) -> (w416:T6)
            n162 = call-dynamic "GenerateAPIEvent_Motor Controller.vi"("error in (no error)"=w418, "API Command Cluster"=w416, "Motor Controller In"=w420) -> ("error out"=w419:errorcluster)  [unwired: 6 in, 2 out]
          }
          event "Read Status": Value Change {
            n163 = event-data() -> ()  [unwired: 1 in, 6 out]
            n164 = Unbundle By Name(w435) -> ("Motor Controller"=w439:refnum<class "Motor Controller.lvclass">)
            n165 = Bundle By Name(cluster=T6 {"Command"=enum."GetExplicitMessage", "Arguments"="", "Data"=variant} ("API Command Cluster"), "Command"=API_Command_Enum."GetExplicitMessage", "Data"=Motor_Controller_Parameter-Get."Servo Enabled?" ("Motor Controller Parameter-Get")) -> (w437:T6)
            n166 = call-dynamic "GenerateAPIEvent_Motor Controller.vi"("Timeout (ms)"=u32 3000, "Wait (F)"=TRUE, "error in (no error)"=w434, "API Command Cluster"=w437, "Motor Controller In"=w439) -> ("error out"=w429:errorcluster, "Return Value"=w431:variant)  [unwired: 4 in, 1 out]
            n167 = Variant To Data(error in=w429, type=u32 0, Variant=w431) -> (data=w427:u32, error out=w428:errorcluster)
            n168 = Equal?(x=w427, y=u32 1) -> (x = y?=w425:bool)
            n169 = local write "Enabled"(w425) -> ()
          }
          event "Enable Ink Ch-1": Value Change {
            n170 = event-data() -> ()  [unwired: 1 in, 6 out]
            n171 = Select(t=API_Command_Enum."Enable Ink Ch-1" ("API Command"), s="Enable Ink Ch-1", f=API_Command_Enum."Disable Ink Ch-1" ("API Command")) -> (s? t:f=w442:T8)
            n172 = Bundle By Name(cluster=w451, "API Command"=w442) -> (w449:T36)
            n173 = call <vilib>:"Add State(s) to Queue__JKI_lib_State_Machine.vi"("State(s) in Front (\"\")"="Ink: Send Enable Command" ("State(s) in Front (\"\")"), "State(s) in (\"\")"=w447) -> ("States Out"=w448:string)  [unwired: 13 in]
          }
          event "Enable Ink Ch-2": Value Change {
            n174 = event-data() -> ()  [unwired: 1 in, 6 out]
            n175 = Select(t=API_Command_Enum."Enable Ink Ch-2" ("API Command"), s="Enable Ink Ch-2", f=API_Command_Enum."Disable Ink Ch-2" ("API Command")) -> (s? t:f=w453:T8)
            n176 = Bundle By Name(cluster=w462, "API Command"=w453) -> (w460:T36)
            n177 = call <vilib>:"Add State(s) to Queue__JKI_lib_State_Machine.vi"("State(s) in Front (\"\")"="Ink: Send Enable Command" ("State(s) in Front (\"\")"), "State(s) in (\"\")"=w458) -> ("States Out"=w459:string)  [unwired: 13 in]
          }
          event "Enable Ink Ch-3": Value Change {
            n178 = event-data() -> ()  [unwired: 1 in, 6 out]
            n179 = Select(t=API_Command_Enum."Enable Ink Ch-3" ("API Command"), s="Enable Ink Ch-3", f=API_Command_Enum."Disable Ink Ch-3" ("API Command")) -> (s? t:f=w464:T8)
            n180 = Bundle By Name(cluster=w473, "API Command"=w464) -> (w471:T36)
            n181 = call <vilib>:"Add State(s) to Queue__JKI_lib_State_Machine.vi"("State(s) in Front (\"\")"="Ink: Send Enable Command" ("State(s) in Front (\"\")"), "State(s) in (\"\")"=w469) -> ("States Out"=w470:string)  [unwired: 13 in]
          }
          event "Enable Ink Ch-4": Value Change {
            n182 = event-data() -> ()  [unwired: 1 in, 6 out]
            n183 = Select(t=API_Command_Enum."Enable Ink Ch-4" ("API Command"), s="Enable Ink Ch-4", f=API_Command_Enum."Disable Ink Ch-4" ("API Command")) -> (s? t:f=w476:T8)
            n184 = Bundle By Name(cluster=w484, "API Command"=w476) -> (w482:T36)
            n185 = call <vilib>:"Add State(s) to Queue__JKI_lib_State_Machine.vi"("State(s) in Front (\"\")"="Ink: Send Enable Command" ("State(s) in Front (\"\")"), "State(s) in (\"\")"=w480) -> ("States Out"=w481:string)  [unwired: 13 in]
          }
          event "Enable Ink Ch-5": Value Change {
            n186 = event-data() -> ()  [unwired: 1 in, 6 out]
            n187 = Select(t=API_Command_Enum."Enable Ink Ch-5" ("API Command"), s="Enable Ink Ch-5", f=API_Command_Enum."Disable Ink Ch-5" ("API Command")) -> (s? t:f=w487:T8)
            n188 = Bundle By Name(cluster=w495, "API Command"=w487) -> (w493:T36)
            n189 = call <vilib>:"Add State(s) to Queue__JKI_lib_State_Machine.vi"("State(s) in Front (\"\")"="Ink: Send Enable Command" ("State(s) in Front (\"\")"), "State(s) in (\"\")"=w491) -> ("States Out"=w492:string)  [unwired: 13 in]
          }
          event "Enable Ink Ch-6": Value Change {
            n190 = event-data() -> ()  [unwired: 1 in, 6 out]
            n191 = Select(t=API_Command_Enum."Enable Ink Ch-6" ("API Command"), s="Enable Ink Ch-6", f=API_Command_Enum."Disable Ink Ch-6" ("API Command")) -> (s? t:f=w498:T8)
            n192 = Bundle By Name(cluster=w506, "API Command"=w498) -> (w504:T36)
            n193 = call <vilib>:"Add State(s) to Queue__JKI_lib_State_Machine.vi"("State(s) in Front (\"\")"="Ink: Send Channel Command" ("State(s) in Front (\"\")"), "State(s) in (\"\")"=w502) -> ("States Out"=w503:string)  [unwired: 13 in]
          }
          event "Spit 1": Value Change {
            n194 = event-data() -> ()  [unwired: 1 in, 6 out]
            n195 = Unbundle By Name(w513) -> ("IO"=w512:refnum<class "IO.lvclass">)
            n196 = call-dynamic "Set ICP2-DO Changed bit.vi"("error in (no error)"=w509, "Value"="Spit 1", "DO Channel"=ICP2-DO_Channel_Names."Meniscus Valve Open - R6", "IO in"=w512) -> ("error out"=w510:errorcluster)  [unwired: 6 in, 1 out]
          }
          event "Spit 2": Value Change {
            n197 = event-data() -> ()  [unwired: 1 in, 6 out]
            n198 = Unbundle By Name(w521) -> ("IO"=w520:refnum<class "IO.lvclass">)
            n199 = call-dynamic "Set ICP2-DO Changed bit.vi"("error in (no error)"=w517, "Value"="Spit 2", "DO Channel"=ICP2-DO_Channel_Names."Ink Flow Valve Open - R1", "IO in"=w520) -> ("error out"=w518:errorcluster)  [unwired: 6 in, 1 out]
          }
          event "Spit 3": Value Change {
            n200 = event-data() -> ()  [unwired: 1 in, 6 out]
            n201 = Unbundle By Name(w529) -> ("IO"=w528:refnum<class "IO.lvclass">)
            n202 = call-dynamic "Set ICP2-DO Changed bit.vi"("error in (no error)"=w525, "Value"="Spit 3", "DO Channel"=ICP2-DO_Channel_Names."Ink Flow Valve Open - R2", "IO in"=w528) -> ("error out"=w526:errorcluster)  [unwired: 6 in, 1 out]
          }
          event "Spit 4": Value Change {
            n203 = event-data() -> ()  [unwired: 1 in, 6 out]
            n204 = Unbundle By Name(w537) -> ("IO"=w536:refnum<class "IO.lvclass">)
            n205 = call-dynamic "Set ICP2-DO Changed bit.vi"("error in (no error)"=w533, "Value"="Spit 4", "DO Channel"=ICP2-DO_Channel_Names."Ink Flow Valve Open - R3", "IO in"=w536) -> ("error out"=w534:errorcluster)  [unwired: 6 in, 1 out]
          }
          event "Spit 5": Value Change {
            n206 = event-data() -> ()  [unwired: 1 in, 6 out]
            n207 = Unbundle By Name(w545) -> ("IO"=w544:refnum<class "IO.lvclass">)
            n208 = call-dynamic "Set ICP2-DO Changed bit.vi"("error in (no error)"=w541, "Value"="Spit 5", "DO Channel"=ICP2-DO_Channel_Names."Ink Flow Valve Open - R4", "IO in"=w544) -> ("error out"=w542:errorcluster)  [unwired: 6 in, 1 out]
          }
          event "Spit 6": Value Change {
            n209 = event-data() -> ()  [unwired: 1 in, 6 out]
            n210 = Unbundle By Name(w553) -> ("IO"=w552:refnum<class "IO.lvclass">)
            n211 = call-dynamic "Set ICP2-DO Changed bit.vi"("error in (no error)"=w549, "Value"="Spit 6", "DO Channel"=ICP2-DO_Channel_Names."Ink Flow Valve Open - R5", "IO in"=w552) -> ("error out"=w550:errorcluster)  [unwired: 6 in, 1 out]
          }
          event "Purge PH Ch-1": Value Change {
            n212 = event-data() -> ()  [unwired: 1 in, 6 out]
            n213 = Bundle By Name(cluster=w562, "Purge\\PrePurge Channel Name"=ICP1-D0_Channel_Names."Purge Valve Open - R1" ("Purge Channel Name")) -> (w557:T36)
            n214 = call <vilib>:"Add State(s) to Queue__JKI_lib_State_Machine.vi"("State(s) in Front (\"\")"="Purge: Send API" ("State(s) in Front (\"\")"), "State(s) in (\"\")"=w559) -> ("States Out"=w560:string)  [unwired: 13 in]
          }
          event "Purge PH Ch-2": Value Change {
            n215 = event-data() -> ()  [unwired: 1 in, 6 out]
            n216 = Bundle By Name(cluster=w570, "Purge\\PrePurge Channel Name"=ICP1-D0_Channel_Names."Purge Valve Open - R2" ("Purge Channel Name")) -> (w565:T36)
            n217 = call <vilib>:"Add State(s) to Queue__JKI_lib_State_Machine.vi"("State(s) in Front (\"\")"="Purge: Send API" ("State(s) in Front (\"\")"), "State(s) in (\"\")"=w567) -> ("States Out"=w568:string)  [unwired: 13 in]
          }
          event "Purge PH Ch-3": Value Change {
            n218 = event-data() -> ()  [unwired: 1 in, 6 out]
            n219 = Bundle By Name(cluster=w578, "Purge\\PrePurge Channel Name"=ICP1-D0_Channel_Names."Purge Valve Open - R3" ("Purge Channel Name")) -> (w573:T36)
            n220 = call <vilib>:"Add State(s) to Queue__JKI_lib_State_Machine.vi"("State(s) in Front (\"\")"="Purge: Send API" ("State(s) in Front (\"\")"), "State(s) in (\"\")"=w575) -> ("States Out"=w576:string)  [unwired: 13 in]
          }
          event "Purge PH Ch-4": Value Change {
            n221 = event-data() -> ()  [unwired: 1 in, 6 out]
            n222 = Bundle By Name(cluster=w586, "Purge\\PrePurge Channel Name"=ICP1-D0_Channel_Names."Purge Valve Open - R4" ("Purge Channel Name")) -> (w581:T36)
            n223 = call <vilib>:"Add State(s) to Queue__JKI_lib_State_Machine.vi"("State(s) in Front (\"\")"="Purge: Send API" ("State(s) in Front (\"\")"), "State(s) in (\"\")"=w583) -> ("States Out"=w584:string)  [unwired: 13 in]
          }
          event "Purge PH Ch-5": Value Change {
            n224 = event-data() -> ()  [unwired: 1 in, 6 out]
            n225 = Bundle By Name(cluster=w594, "Purge\\PrePurge Channel Name"=ICP1-D0_Channel_Names."Purge Valve Open - R5" ("Purge Channel Name")) -> (w589:T36)
            n226 = call <vilib>:"Add State(s) to Queue__JKI_lib_State_Machine.vi"("State(s) in Front (\"\")"="Purge: Send API" ("State(s) in Front (\"\")"), "State(s) in (\"\")"=w591) -> ("States Out"=w592:string)  [unwired: 13 in]
          }
          event "Purge PH Ch-6": Value Change {
            n227 = event-data() -> ()  [unwired: 1 in, 6 out]
            n228 = Bundle By Name(cluster=w602, "Purge\\PrePurge Channel Name"=ICP1-D0_Channel_Names."Purge Valve Open - R6" ("Purge Channel Name")) -> (w597:T36)
            n229 = call <vilib>:"Add State(s) to Queue__JKI_lib_State_Machine.vi"("State(s) in Front (\"\")"="Purge: Send API" ("State(s) in Front (\"\")"), "State(s) in (\"\")"=w599) -> ("States Out"=w600:string)  [unwired: 13 in]
          }
          event "Pre Purge PH Ch-1": Value Change {
            n230 = event-data() -> ()  [unwired: 1 in, 6 out]
            n231 = Bundle By Name(cluster=w612, "Purge\\PrePurge Channel Name"=ICP1-D0_Channel_Names."Purge Valve Open - R1" ("Purge\\PrePurge Channel Name"), "Pre Purge Parameters"="Pre Purge PH Ch-1 Parameters") -> (w606:T36)
            n232 = call <vilib>:"Add State(s) to Queue__JKI_lib_State_Machine.vi"("State(s) in Front (\"\")"="  Pre Purge: Send API", "State(s) in (\"\")"=w608) -> ("States Out"=w609:string)  [unwired: 13 in]
          }
          event "Pre Purge PH Ch-2": Value Change {
            n233 = event-data() -> ()  [unwired: 1 in, 6 out]
            n234 = Bundle By Name(cluster=w621, "Purge\\PrePurge Channel Name"=ICP1-D0_Channel_Names."Purge Valve Open - R2" ("Purge\\PrePurge Channel Name"), "Pre Purge Parameters"="Pre Purge PH Ch-2 Parameters") -> (w615:T36)
            n235 = call <vilib>:"Add State(s) to Queue__JKI_lib_State_Machine.vi"("State(s) in Front (\"\")"="  Pre Purge: Send API", "State(s) in (\"\")"=w617) -> ("States Out"=w618:string)  [unwired: 13 in]
          }
          event "Pre Purge PH Ch-3": Value Change {
            n236 = event-data() -> ()  [unwired: 1 in, 6 out]
            n237 = Bundle By Name(cluster=w630, "Purge\\PrePurge Channel Name"=ICP1-D0_Channel_Names."Purge Valve Open - R3" ("Purge\\PrePurge Channel Name"), "Pre Purge Parameters"="Pre Purge PH Ch-3 Parameters") -> (w624:T36)
            n238 = call <vilib>:"Add State(s) to Queue__JKI_lib_State_Machine.vi"("State(s) in Front (\"\")"="  Pre Purge: Send API", "State(s) in (\"\")"=w626) -> ("States Out"=w627:string)  [unwired: 13 in]
          }
          event "Pre Purge PH Ch-4": Value Change {
            n239 = event-data() -> ()  [unwired: 1 in, 6 out]
            n240 = Bundle By Name(cluster=w639, "Purge\\PrePurge Channel Name"=ICP1-D0_Channel_Names."Purge Valve Open - R4" ("Purge\\PrePurge Channel Name"), "Pre Purge Parameters"="Pre Purge PH Ch-4 Parameters") -> (w633:T36)
            n241 = call <vilib>:"Add State(s) to Queue__JKI_lib_State_Machine.vi"("State(s) in Front (\"\")"="  Pre Purge: Send API", "State(s) in (\"\")"=w635) -> ("States Out"=w636:string)  [unwired: 13 in]
          }
          event "Pre Purge PH Ch-5": Value Change {
            n242 = event-data() -> ()  [unwired: 1 in, 6 out]
            n243 = Bundle By Name(cluster=w648, "Purge\\PrePurge Channel Name"=ICP1-D0_Channel_Names."Purge Valve Open - R5" ("Purge\\PrePurge Channel Name"), "Pre Purge Parameters"="Pre Purge PH Ch-5 Parameters") -> (w642:T36)
            n244 = call <vilib>:"Add State(s) to Queue__JKI_lib_State_Machine.vi"("State(s) in Front (\"\")"="  Pre Purge: Send API", "State(s) in (\"\")"=w644) -> ("States Out"=w645:string)  [unwired: 13 in]
          }
          event "Pre Purge PH Ch-6": Value Change {
            n245 = event-data() -> ()  [unwired: 1 in, 6 out]
            n246 = Bundle By Name(cluster=w657, "Purge\\PrePurge Channel Name"=ICP1-D0_Channel_Names."Purge Valve Open - R6" ("Purge\\PrePurge Channel Name"), "Pre Purge Parameters"="Pre Purge PH Ch-6 Parameters") -> (w651:T36)
            n247 = call <vilib>:"Add State(s) to Queue__JKI_lib_State_Machine.vi"("State(s) in Front (\"\")"="  Pre Purge: Send API", "State(s) in (\"\")"=w653) -> ("States Out"=w654:string)  [unwired: 13 in]
          }
          event "Print": Value Change {
            n248 = event-data() -> ()  [unwired: 1 in, 6 out]
            n249 = Bundle By Name(cluster=T11 {"Command File Path"=path "", "No. of Print Repeats"=1, "HomeOnComplete"=FALSE}, "Command File Path"="Command File Path", "No. of Print Repeats"="Print Passes", "HomeOnComplete"="HomeOnComplete") -> (w662:T11)
            n250 = Bundle By Name(cluster=T12 {"Command"=enum."Execute Printer Commands", "Arguments"="", "Data"=variant} ("API Command Cluster"), "Command"=API_Command_Enum."Execute Printer Commands", "Data"=w662) -> (w666:T12)
            n251 = call-dynamic "GenerateAPIEvent_TopLevel.vi"("Wait (F)"=FALSE, "error in (no error)"=w668, "API Command Cluster"=w666, "TopLevel in"=w670) -> ("error out"=w669:errorcluster, "TopLevel out"=w671:refnum<class "TopLevel.lvclass">)  [unwired: 6 in]
          }
          event "IdlePrint": Value Change {
            n252 = event-data() -> ("NewVal"=w676:bool)  [unwired: 1 in, 5 out]
            n253 = case shown="True" w676 {
              tunnel: [API_Command_Enum."StopIdlePrintCycle" ("Command") API_Command_Enum."ExecuteIdlePrintCycle" ("Command")] -> w680
              tunnel: [w689 w697] -> w679
              tunnel: w676 -> [_ w694]
              tunnel: ["UI: SetUIControlsState>>enable" ("State(s) in Front (\"\")") "UI: SetUIControlsState>>disable" ("State(s) in Front (\"\")")] -> w673
              frame False {
                n254 = Bundle By Name(cluster=T13 {"Command File Path"=path "", "IdleMode"=FALSE, "IdleCycleInterval(s)"=0.0} ("Cluster"), "IdleMode"=FALSE) -> (w689:T13)
              }
              frame True {
                n255 = property on="Command File Path" class="Path"() -> ("Value"=w693:path)  [unwired: 2 in, 2 out]
                n256 = Bundle By Name(cluster=T13 {"Command File Path"=path "", "IdleMode"=FALSE, "IdleCycleInterval(s)"=0.0} ("Cluster"), "Command File Path"=w693, "IdleMode"=w694, "IdleCycleInterval(s)"="Idle Intervals (s)") -> (w697:T13)
              }
            }
            n257 = Bundle By Name(cluster=T12 {"Command"=enum."Execute Printer Commands", "Arguments"="", "Data"=variant} ("API Command Cluster"), "Command"=w680, "Data"=w679) -> (w681:T12)
            n258 = call-dynamic "GenerateAPIEvent_TopLevel.vi"("Wait (F)"=FALSE, "error in (no error)"=w683, "API Command Cluster"=w681, "TopLevel in"=w685) -> ("error out"=w684:errorcluster, "TopLevel out"=w686:refnum<class "TopLevel.lvclass">)  [unwired: 6 in]
            n259 = call <vilib>:"Add State(s) to Queue__JKI_lib_State_Machine.vi"("State(s) in Front (\"\")"=w673, "State(s) in (\"\")"=w674) -> ("States Out"=w675:string)  [unwired: 13 in]
          }
          event "PH1-Prime": Value Change {
            n260 = event-data() -> ()  [unwired: 1 in, 6 out]
            n261 = Unbundle By Name(w700) -> ("Methods:Accessors:Digilens Config.PrinterConfiguration.PH1-Prime Path"=w699:path)
            n262 = Bundle By Name(cluster=T11 {"Command File Path"=path "", "No. of Print Repeats"=1, "HomeOnComplete"=FALSE}, "Command File Path"=w699, "No. of Print Repeats"=1) -> (w702:T11)
            n263 = Bundle By Name(cluster=T12 {"Command"=enum."Execute Printer Commands", "Arguments"="", "Data"=variant} ("API Command Cluster"), "Command"=API_Command_Enum."Execute Printer Commands", "Data"=w702) -> (w705:T12)
            n264 = call-dynamic "GenerateAPIEvent_TopLevel.vi"("error in (no error)"=w707, "API Command Cluster"=w705, "TopLevel in"=w709) -> ("error out"=w708:errorcluster, "TopLevel out"=w710:refnum<class "TopLevel.lvclass">)  [unwired: 7 in]
          }
          event "Enable PH1 Heat": Value Change {
            n265 = event-data() -> ("NewVal"=w715:bool)  [unwired: 1 in, 5 out]
            n266 = Unbundle By Name(w716) -> ("Methods:Accessors:Digilens Config.PrinterConfiguration.PH1-HeatOn Path"=w713:path, "Methods:Accessors:Digilens Config.PrinterConfiguration.PH1-HeatOff Path"=w714:path)
            n267 = Select(t=w713, s=w715, f=w714) -> (s? t:f=w712:path)
            n268 = Bundle By Name(cluster=T11 {"Command File Path"=path "", "No. of Print Repeats"=1, "HomeOnComplete"=FALSE}, "Command File Path"=w712, "No. of Print Repeats"=1) -> (w718:T11)
            n269 = Bundle By Name(cluster=T12 {"Command"=enum."Execute Printer Commands", "Arguments"="", "Data"=variant} ("API Command Cluster"), "Command"=API_Command_Enum."Execute Printer Commands", "Data"=w718) -> (w721:T12)
            n270 = call-dynamic "GenerateAPIEvent_TopLevel.vi"("error in (no error)"=w723, "API Command Cluster"=w721, "TopLevel in"=w725) -> ("error out"=w724:errorcluster, "TopLevel out"=w726:refnum<class "TopLevel.lvclass">)  [unwired: 7 in]
          }
          event "Enable PH2 Heat": Value Change {
            n271 = event-data() -> ("NewVal"=w731:bool)  [unwired: 1 in, 5 out]
            n272 = Unbundle By Name(w732) -> ("Methods:Accessors:Digilens Config.PrinterConfiguration.PH2-HeatOn Path"=w729:path, "Methods:Accessors:Digilens Config.PrinterConfiguration.PH2-HeatOff Path"=w730:path)
            n273 = Select(t=w729, s=w731, f=w730) -> (s? t:f=w728:path)
            n274 = Bundle By Name(cluster=T11 {"Command File Path"=path "", "No. of Print Repeats"=1, "HomeOnComplete"=FALSE}, "Command File Path"=w728, "No. of Print Repeats"=1) -> (w734:T11)
            n275 = Bundle By Name(cluster=T12 {"Command"=enum."Execute Printer Commands", "Arguments"="", "Data"=variant} ("API Command Cluster"), "Command"=API_Command_Enum."Execute Printer Commands", "Data"=w734) -> (w737:T12)
            n276 = call-dynamic "GenerateAPIEvent_TopLevel.vi"("error in (no error)"=w739, "API Command Cluster"=w737, "TopLevel in"=w741) -> ("error out"=w740:errorcluster, "TopLevel out"=w742:refnum<class "TopLevel.lvclass">)  [unwired: 7 in]
          }
          event "Enable PH3 Heat": Value Change {
            n277 = event-data() -> ("NewVal"=w747:bool)  [unwired: 1 in, 5 out]
            n278 = Unbundle By Name(w748) -> ("Methods:Accessors:Digilens Config.PrinterConfiguration.PH3-HeatOn Path"=w745:path, "Methods:Accessors:Digilens Config.PrinterConfiguration.PH3-HeatOff Path"=w746:path)
            n279 = Select(t=w745, s=w747, f=w746) -> (s? t:f=w744:path)
            n280 = Bundle By Name(cluster=T11 {"Command File Path"=path "", "No. of Print Repeats"=1, "HomeOnComplete"=FALSE}, "Command File Path"=w744, "No. of Print Repeats"=1) -> (w750:T11)
            n281 = Bundle By Name(cluster=T12 {"Command"=enum."Execute Printer Commands", "Arguments"="", "Data"=variant} ("API Command Cluster"), "Command"=API_Command_Enum."Execute Printer Commands", "Data"=w750) -> (w753:T12)
            n282 = call-dynamic "GenerateAPIEvent_TopLevel.vi"("error in (no error)"=w755, "API Command Cluster"=w753, "TopLevel in"=w757) -> ("error out"=w756:errorcluster, "TopLevel out"=w758:refnum<class "TopLevel.lvclass">)  [unwired: 7 in]
          }
          event "Enable PH4 Heat": Value Change {
            n283 = event-data() -> ("NewVal"=w763:bool)  [unwired: 1 in, 5 out]
            n284 = Unbundle By Name(w764) -> ("Methods:Accessors:Digilens Config.PrinterConfiguration.PH4-HeatOn Path"=w761:path, "Methods:Accessors:Digilens Config.PrinterConfiguration.PH4-HeatOff Path"=w762:path)
            n285 = Select(t=w761, s=w763, f=w762) -> (s? t:f=w760:path)
            n286 = Bundle By Name(cluster=T11 {"Command File Path"=path "", "No. of Print Repeats"=1, "HomeOnComplete"=FALSE}, "Command File Path"=w760, "No. of Print Repeats"=1) -> (w766:T11)
            n287 = Bundle By Name(cluster=T12 {"Command"=enum."Execute Printer Commands", "Arguments"="", "Data"=variant} ("API Command Cluster"), "Command"=API_Command_Enum."Execute Printer Commands", "Data"=w766) -> (w769:T12)
            n288 = call-dynamic "GenerateAPIEvent_TopLevel.vi"("error in (no error)"=w771, "API Command Cluster"=w769, "TopLevel in"=w773) -> ("error out"=w772:errorcluster, "TopLevel out"=w774:refnum<class "TopLevel.lvclass">)  [unwired: 7 in]
          }
          event "Enable PH5 Heat": Value Change {
            n289 = event-data() -> ("NewVal"=w779:bool)  [unwired: 1 in, 5 out]
            n290 = Unbundle By Name(w780) -> ("Methods:Accessors:Digilens Config.PrinterConfiguration.PH5-HeatOn Path"=w777:path, "Methods:Accessors:Digilens Config.PrinterConfiguration.PH5-HeatOff Path"=w778:path)
            n291 = Select(t=w777, s=w779, f=w778) -> (s? t:f=w776:path)
            n292 = Bundle By Name(cluster=T11 {"Command File Path"=path "", "No. of Print Repeats"=1, "HomeOnComplete"=FALSE}, "Command File Path"=w776, "No. of Print Repeats"=1) -> (w782:T11)
            n293 = Bundle By Name(cluster=T12 {"Command"=enum."Execute Printer Commands", "Arguments"="", "Data"=variant} ("API Command Cluster"), "Command"=API_Command_Enum."Execute Printer Commands", "Data"=w782) -> (w785:T12)
            n294 = call-dynamic "GenerateAPIEvent_TopLevel.vi"("error in (no error)"=w787, "API Command Cluster"=w785, "TopLevel in"=w789) -> ("error out"=w788:errorcluster, "TopLevel out"=w790:refnum<class "TopLevel.lvclass">)  [unwired: 7 in]
          }
          event "Enable PH6 Heat": Value Change {
            n295 = event-data() -> ("NewVal"=w795:bool)  [unwired: 1 in, 5 out]
            n296 = Unbundle By Name(w796) -> ("Methods:Accessors:Digilens Config.PrinterConfiguration.PH6-HeatOn Path"=w793:path, "Methods:Accessors:Digilens Config.PrinterConfiguration.PH6-HeatOff Path"=w794:path)
            n297 = Select(t=w793, s=w795, f=w794) -> (s? t:f=w792:path)
            n298 = Bundle By Name(cluster=T11 {"Command File Path"=path "", "No. of Print Repeats"=1, "HomeOnComplete"=FALSE}, "Command File Path"=w792, "No. of Print Repeats"=1) -> (w798:T11)
            n299 = Bundle By Name(cluster=T12 {"Command"=enum."Execute Printer Commands", "Arguments"="", "Data"=variant} ("API Command Cluster"), "Command"=API_Command_Enum."Execute Printer Commands", "Data"=w798) -> (w801:T12)
            n300 = call-dynamic "GenerateAPIEvent_TopLevel.vi"("error in (no error)"=w803, "API Command Cluster"=w801, "TopLevel in"=w805) -> ("error out"=w804:errorcluster, "TopLevel out"=w806:refnum<class "TopLevel.lvclass">)  [unwired: 7 in]
          }
          event "PH2-Prime": Value Change {
            n301 = event-data() -> ()  [unwired: 1 in, 6 out]
            n302 = Unbundle By Name(w809) -> ("Methods:Accessors:Digilens Config.PrinterConfiguration.PH2-Prime Path"=w808:path)
            n303 = Bundle By Name(cluster=T11 {"Command File Path"=path "", "No. of Print Repeats"=1, "HomeOnComplete"=FALSE}, "Command File Path"=w808, "No. of Print Repeats"=1) -> (w811:T11)
            n304 = Bundle By Name(cluster=T12 {"Command"=enum."Execute Printer Commands", "Arguments"="", "Data"=variant} ("API Command Cluster"), "Command"=API_Command_Enum."Execute Printer Commands", "Data"=w811) -> (w814:T12)
            n305 = call-dynamic "GenerateAPIEvent_TopLevel.vi"("error in (no error)"=w816, "API Command Cluster"=w814, "TopLevel in"=w818) -> ("error out"=w817:errorcluster, "TopLevel out"=w819:refnum<class "TopLevel.lvclass">)  [unwired: 7 in]
          }
          event "PH3-Prime": Value Change {
            n306 = event-data() -> ()  [unwired: 1 in, 6 out]
            n307 = Unbundle By Name(w822) -> ("Methods:Accessors:Digilens Config.PrinterConfiguration.PH3-Prime Path"=w821:path)
            n308 = Bundle By Name(cluster=T11 {"Command File Path"=path "", "No. of Print Repeats"=1, "HomeOnComplete"=FALSE}, "Command File Path"=w821, "No. of Print Repeats"=1) -> (w824:T11)
            n309 = Bundle By Name(cluster=T12 {"Command"=enum."Execute Printer Commands", "Arguments"="", "Data"=variant} ("API Command Cluster"), "Command"=API_Command_Enum."Execute Printer Commands", "Data"=w824) -> (w827:T12)
            n310 = call-dynamic "GenerateAPIEvent_TopLevel.vi"("error in (no error)"=w829, "API Command Cluster"=w827, "TopLevel in"=w831) -> ("error out"=w830:errorcluster, "TopLevel out"=w832:refnum<class "TopLevel.lvclass">)  [unwired: 7 in]
          }
          event "PH4-Prime": Value Change {
            n311 = event-data() -> ()  [unwired: 1 in, 6 out]
            n312 = Unbundle By Name(w835) -> ("Methods:Accessors:Digilens Config.PrinterConfiguration.PH4-Prime Path"=w834:path)
            n313 = Bundle By Name(cluster=T11 {"Command File Path"=path "", "No. of Print Repeats"=1, "HomeOnComplete"=FALSE}, "Command File Path"=w834, "No. of Print Repeats"=1) -> (w837:T11)
            n314 = Bundle By Name(cluster=T12 {"Command"=enum."Execute Printer Commands", "Arguments"="", "Data"=variant} ("API Command Cluster"), "Command"=API_Command_Enum."Execute Printer Commands", "Data"=w837) -> (w840:T12)
            n315 = call-dynamic "GenerateAPIEvent_TopLevel.vi"("error in (no error)"=w842, "API Command Cluster"=w840, "TopLevel in"=w844) -> ("error out"=w843:errorcluster, "TopLevel out"=w845:refnum<class "TopLevel.lvclass">)  [unwired: 7 in]
          }
          event "PH5-Prime": Value Change {
            n316 = event-data() -> ()  [unwired: 1 in, 6 out]
            n317 = Unbundle By Name(w848) -> ("Methods:Accessors:Digilens Config.PrinterConfiguration.PH5-Prime Path"=w847:path)
            n318 = Bundle By Name(cluster=T11 {"Command File Path"=path "", "No. of Print Repeats"=1, "HomeOnComplete"=FALSE}, "Command File Path"=w847, "No. of Print Repeats"=1) -> (w850:T11)
            n319 = Bundle By Name(cluster=T12 {"Command"=enum."Execute Printer Commands", "Arguments"="", "Data"=variant} ("API Command Cluster"), "Command"=API_Command_Enum."Execute Printer Commands", "Data"=w850) -> (w853:T12)
            n320 = call-dynamic "GenerateAPIEvent_TopLevel.vi"("error in (no error)"=w855, "API Command Cluster"=w853, "TopLevel in"=w857) -> ("error out"=w856:errorcluster, "TopLevel out"=w858:refnum<class "TopLevel.lvclass">)  [unwired: 7 in]
          }
          event "PH6-Prime": Value Change {
            n321 = event-data() -> ()  [unwired: 1 in, 6 out]
            n322 = Unbundle By Name(w861) -> ("Methods:Accessors:Digilens Config.PrinterConfiguration.PH6-Prime Path"=w860:path)
            n323 = Bundle By Name(cluster=T11 {"Command File Path"=path "", "No. of Print Repeats"=1, "HomeOnComplete"=FALSE}, "Command File Path"=w860, "No. of Print Repeats"=1) -> (w863:T11)
            n324 = Bundle By Name(cluster=T12 {"Command"=enum."Execute Printer Commands", "Arguments"="", "Data"=variant} ("API Command Cluster"), "Command"=API_Command_Enum."Execute Printer Commands", "Data"=w863) -> (w866:T12)
            n325 = call-dynamic "GenerateAPIEvent_TopLevel.vi"("error in (no error)"=w868, "API Command Cluster"=w866, "TopLevel in"=w870) -> ("error out"=w869:errorcluster, "TopLevel out"=w871:refnum<class "TopLevel.lvclass">)  [unwired: 7 in]
          }
          event User Event {
            n326 = event-data() -> ()  [unwired: 1 in, 6 out]
            n327 = Unbundle By Name(w880) -> ("GIS Printer"=w879:refnum<class "GIS Printer.lvclass">)
            n328 = call-dynamic "GetTCPCommandsResponses_GIS Printer.vi"("error in (no error)"=w877, "gis in"=w879) -> ("error out"=w878:errorcluster, "TCP Commands & Responses"=w876:string[][])  [unwired: 7 in, 1 out]
            n329 = property on="TCP Commands & Responses" class="MCListbox (strict)"("ItemNames"=w876) -> ()  [unwired: 2 in, 2 out]
            n330 = call <vilib>:"Add State(s) to Queue__JKI_lib_State_Machine.vi"("State(s) in Front (\"\")"="UI: Update Stage Busy", "State(s) in (\"\")"=w874) -> ("States Out"=w875:string)  [unwired: 13 in]
          }
          event "Meniscus Valve Open - R1": Value Change {
            n331 = event-data() -> ()  [unwired: 1 in, 6 out]
            n332 = Unbundle By Name(w886) -> ("IO"=w885:refnum<class "IO.lvclass">)
            n333 = call-dynamic "Set ICP2-DO Changed bit.vi"("error in (no error)"=w882, "Value"="Meniscus Valve Open - R1", "DO Channel"=ICP2-DO_Channel_Names."Meniscus Valve Open - R1", "IO in"=w885) -> ("error out"=w883:errorcluster)  [unwired: 6 in, 1 out]
          }
          event "Meniscus Valve Open - R2": Value Change {
            n334 = event-data() -> ()  [unwired: 1 in, 6 out]
            n335 = Unbundle By Name(w894) -> ("IO"=w893:refnum<class "IO.lvclass">)
            n336 = call-dynamic "Set ICP2-DO Changed bit.vi"("error in (no error)"=w891, "Value"="Meniscus Valve Open - R2", "DO Channel"=ICP2-DO_Channel_Names."Meniscus Valve Open - R2", "IO in"=w893) -> ("error out"=w892:errorcluster)  [unwired: 6 in, 1 out]
          }
          event "Meniscus Valve Open - R3": Value Change {
            n337 = event-data() -> ()  [unwired: 1 in, 6 out]
            n338 = Unbundle By Name(w902) -> ("IO"=w901:refnum<class "IO.lvclass">)
            n339 = call-dynamic "Set ICP2-DO Changed bit.vi"("error in (no error)"=w899, "Value"="Meniscus Valve Open - R3", "DO Channel"=ICP2-DO_Channel_Names."Meniscus Valve Open - R3", "IO in"=w901) -> ("error out"=w900:errorcluster)  [unwired: 6 in, 1 out]
          }
          event "Meniscus Valve Open - R4": Value Change {
            n340 = event-data() -> ()  [unwired: 1 in, 6 out]
            n341 = Unbundle By Name(w910) -> ("IO"=w909:refnum<class "IO.lvclass">)
            n342 = call-dynamic "Set ICP2-DO Changed bit.vi"("error in (no error)"=w907, "Value"="Meniscus Valve Open - R4", "DO Channel"=ICP2-DO_Channel_Names."Meniscus Valve Open - R4", "IO in"=w909) -> ("error out"=w908:errorcluster)  [unwired: 6 in, 1 out]
          }
          event "Meniscus Valve Open - R5": Value Change {
            n343 = event-data() -> ()  [unwired: 1 in, 6 out]
            n344 = Unbundle By Name(w918) -> ("IO"=w917:refnum<class "IO.lvclass">)
            n345 = call-dynamic "Set ICP2-DO Changed bit.vi"("error in (no error)"=w915, "Value"="Meniscus Valve Open - R5", "DO Channel"=ICP2-DO_Channel_Names."Meniscus Valve Open - R5", "IO in"=w917) -> ("error out"=w916:errorcluster)  [unwired: 6 in, 1 out]
          }
          event "Meniscus Valve Open - R6": Value Change {
            n346 = event-data() -> ()  [unwired: 1 in, 6 out]
            n347 = Unbundle By Name(w926) -> ("IO"=w925:refnum<class "IO.lvclass">)
            n348 = call-dynamic "Set ICP2-DO Changed bit.vi"("error in (no error)"=w923, "Value"="Meniscus Valve Open - R6", "DO Channel"=ICP2-DO_Channel_Names."Meniscus Valve Open - R6", "IO in"=w925) -> ("error out"=w924:errorcluster)  [unwired: 6 in, 1 out]
          }
          event "Ink Flow Valve Open - R1": Value Change {
            n349 = event-data() -> ()  [unwired: 1 in, 6 out]
            n350 = Unbundle By Name(w934) -> ("IO"=w933:refnum<class "IO.lvclass">)
            n351 = call-dynamic "Set ICP2-DO Changed bit.vi"("error in (no error)"=w931, "Value"="Ink Flow Valve Open - R1", "DO Channel"=ICP2-DO_Channel_Names."Ink Flow Valve Open - R1", "IO in"=w933) -> ("error out"=w932:errorcluster)  [unwired: 6 in, 1 out]
          }
          event "Ink Flow Valve Open - R2": Value Change {
            n352 = event-data() -> ()  [unwired: 1 in, 6 out]
            n353 = Unbundle By Name(w942) -> ("IO"=w941:refnum<class "IO.lvclass">)
            n354 = call-dynamic "Set ICP2-DO Changed bit.vi"("error in (no error)"=w939, "Value"="Ink Flow Valve Open - R2", "DO Channel"=ICP2-DO_Channel_Names."Ink Flow Valve Open - R2", "IO in"=w941) -> ("error out"=w940:errorcluster)  [unwired: 6 in, 1 out]
          }
          event "Ink Flow Valve Open - R3": Value Change {
            n355 = event-data() -> ()  [unwired: 1 in, 6 out]
            n356 = Unbundle By Name(w950) -> ("IO"=w949:refnum<class "IO.lvclass">)
            n357 = call-dynamic "Set ICP2-DO Changed bit.vi"("error in (no error)"=w947, "Value"="Ink Flow Valve Open - R3", "DO Channel"=ICP2-DO_Channel_Names."Ink Flow Valve Open - R3", "IO in"=w949) -> ("error out"=w948:errorcluster)  [unwired: 6 in, 1 out]
          }
          event "Ink Flow Valve Open - R4": Value Change {
            n358 = event-data() -> ()  [unwired: 1 in, 6 out]
            n359 = Unbundle By Name(w958) -> ("IO"=w957:refnum<class "IO.lvclass">)
            n360 = call-dynamic "Set ICP2-DO Changed bit.vi"("error in (no error)"=w955, "Value"="Ink Flow Valve Open - R4", "DO Channel"=ICP2-DO_Channel_Names."Ink Flow Valve Open - R4", "IO in"=w957) -> ("error out"=w956:errorcluster)  [unwired: 6 in, 1 out]
          }
          event "Ink Flow Valve Open - R5": Value Change {
            n361 = event-data() -> ()  [unwired: 1 in, 6 out]
            n362 = Unbundle By Name(w966) -> ("IO"=w965:refnum<class "IO.lvclass">)
            n363 = call-dynamic "Set ICP2-DO Changed bit.vi"("error in (no error)"=w963, "Value"="Ink Flow Valve Open - R5", "DO Channel"=ICP2-DO_Channel_Names."Ink Flow Valve Open - R5", "IO in"=w965) -> ("error out"=w964:errorcluster)  [unwired: 6 in, 1 out]
          }
          event "Ink Flow Valve Open - R6": Value Change {
            n364 = event-data() -> ()  [unwired: 1 in, 6 out]
            n365 = Unbundle By Name(w974) -> ("IO"=w973:refnum<class "IO.lvclass">)
            n366 = call-dynamic "Set ICP2-DO Changed bit.vi"("error in (no error)"=w971, "Value"="Ink Flow Valve Open - R6", "DO Channel"=ICP2-DO_Channel_Names."Ink Flow Valve Open - R6", "IO in"=w973) -> ("error out"=w972:errorcluster)  [unwired: 6 in, 1 out]
          }
          event "SW_LED - Ink Valve - R1": Value Change {
            n367 = event-data() -> ()  [unwired: 1 in, 6 out]
            n368 = Unbundle By Name(w982) -> ("IO"=w981:refnum<class "IO.lvclass">)
            n369 = call-dynamic "Set ICP2-DO Changed bit.vi"("error in (no error)"=w979, "Value"="SW_LED - Ink Valve - R1", "DO Channel"=ICP2-DO_Channel_Names."SW_LED - Ink Valve - R1", "IO in"=w981) -> ("error out"=w980:errorcluster)  [unwired: 6 in, 1 out]
          }
          event "SW_LED - Ink Valve - R2": Value Change {
            n370 = event-data() -> ()  [unwired: 1 in, 6 out]
            n371 = Unbundle By Name(w990) -> ("IO"=w989:refnum<class "IO.lvclass">)
            n372 = call-dynamic "Set ICP2-DO Changed bit.vi"("error in (no error)"=w987, "Value"="SW_LED - Ink Valve - R2", "DO Channel"=ICP2-DO_Channel_Names."SW_LED - Ink Valve - R2", "IO in"=w989) -> ("error out"=w988:errorcluster)  [unwired: 6 in, 1 out]
          }
          event "SW_LED - Ink Valve - R3": Value Change {
            n373 = event-data() -> ()  [unwired: 1 in, 6 out]
            n374 = Unbundle By Name(w998) -> ("IO"=w997:refnum<class "IO.lvclass">)
            n375 = call-dynamic "Set ICP2-DO Changed bit.vi"("error in (no error)"=w995, "Value"="SW_LED - Ink Valve - R3", "DO Channel"=ICP2-DO_Channel_Names."SW_LED - Ink Valve - R3", "IO in"=w997) -> ("error out"=w996:errorcluster)  [unwired: 6 in, 1 out]
          }
          event "SW_LED - Ink Valve - R4": Value Change {
            n376 = event-data() -> ()  [unwired: 1 in, 6 out]
            n377 = Unbundle By Name(w1006) -> ("IO"=w1005:refnum<class "IO.lvclass">)
            n378 = call-dynamic "Set ICP2-DO Changed bit.vi"("error in (no error)"=w1003, "Value"="SW_LED - Ink Valve - R4", "DO Channel"=ICP2-DO_Channel_Names."SW_LED - Ink Valve - R4", "IO in"=w1005) -> ("error out"=w1004:errorcluster)  [unwired: 6 in, 1 out]
          }
          event "SW_LED - Ink Valve - R5": Value Change {
            n379 = event-data() -> ()  [unwired: 1 in, 6 out]
            n380 = Unbundle By Name(w1014) -> ("IO"=w1013:refnum<class "IO.lvclass">)
            n381 = call-dynamic "Set ICP2-DO Changed bit.vi"("error in (no error)"=w1011, "Value"="SW_LED - Ink Valve - R5", "DO Channel"=ICP2-DO_Channel_Names."SW_LED - Ink Valve - R5", "IO in"=w1013) -> ("error out"=w1012:errorcluster)  [unwired: 6 in, 1 out]
          }
          event "SW_LED - Ink Valve - R6": Value Change {
            n382 = event-data() -> ()  [unwired: 1 in, 6 out]
            n383 = Unbundle By Name(w1022) -> ("IO"=w1021:refnum<class "IO.lvclass">)
            n384 = call-dynamic "Set ICP2-DO Changed bit.vi"("error in (no error)"=w1019, "Value"="SW_LED - Ink Valve - R6", "DO Channel"=ICP2-DO_Channel_Names."SW_LED - Ink Valve - R6", "IO in"=w1021) -> ("error out"=w1020:errorcluster)  [unwired: 6 in, 1 out]
          }
          event "Recirc Pump On - R1": Value Change {
            n385 = event-data() -> ()  [unwired: 1 in, 6 out]
            n386 = Unbundle By Name(w1030) -> ("IO"=w1029:refnum<class "IO.lvclass">)
            n387 = call-dynamic "Set ICP2-DO Changed bit.vi"("error in (no error)"=w1027, "Value"="Recirc Pump On - R1", "DO Channel"=ICP2-DO_Channel_Names."Recirc Pump On - R1", "IO in"=w1029) -> ("error out"=w1028:errorcluster)  [unwired: 6 in, 1 out]
          }
          event "Recirc Pump On - R2": Value Change {
            n388 = event-data() -> ()  [unwired: 1 in, 6 out]
            n389 = Unbundle By Name(w1038) -> ("IO"=w1037:refnum<class "IO.lvclass">)
            n390 = call-dynamic "Set ICP2-DO Changed bit.vi"("error in (no error)"=w1035, "Value"="Recirc Pump On - R2", "DO Channel"=ICP2-DO_Channel_Names."Recirc Pump On - R2", "IO in"=w1037) -> ("error out"=w1036:errorcluster)  [unwired: 6 in, 1 out]
          }
          event "Recirc Pump On - R3": Value Change {
            n391 = event-data() -> ()  [unwired: 1 in, 6 out]
            n392 = Unbundle By Name(w1046) -> ("IO"=w1045:refnum<class "IO.lvclass">)
            n393 = call-dynamic "Set ICP2-DO Changed bit.vi"("error in (no error)"=w1043, "Value"="Recirc Pump On - R3", "DO Channel"=ICP2-DO_Channel_Names."Recirc Pump On - R3", "IO in"=w1045) -> ("error out"=w1044:errorcluster)  [unwired: 6 in, 1 out]
          }
          event "Recirc Pump On - R4": Value Change {
            n394 = event-data() -> ()  [unwired: 1 in, 6 out]
            n395 = Unbundle By Name(w1054) -> ("IO"=w1053:refnum<class "IO.lvclass">)
            n396 = call-dynamic "Set ICP2-DO Changed bit.vi"("error in (no error)"=w1051, "Value"="Recirc Pump On - R4", "DO Channel"=ICP2-DO_Channel_Names."Recirc Pump On - R4", "IO in"=w1053) -> ("error out"=w1052:errorcluster)  [unwired: 6 in, 1 out]
          }
          event "Recirc Pump On - R5": Value Change {
            n397 = event-data() -> ()  [unwired: 1 in, 6 out]
            n398 = Unbundle By Name(w1062) -> ("IO"=w1061:refnum<class "IO.lvclass">)
            n399 = call-dynamic "Set ICP2-DO Changed bit.vi"("error in (no error)"=w1059, "Value"="Recirc Pump On - R5", "DO Channel"=ICP2-DO_Channel_Names."Recirc Pump On - R5", "IO in"=w1061) -> ("error out"=w1060:errorcluster)  [unwired: 6 in, 1 out]
          }
          event "Recirc Pump On - R6": Value Change {
            n400 = event-data() -> ()  [unwired: 1 in, 6 out]
            n401 = Unbundle By Name(w1070) -> ("IO"=w1069:refnum<class "IO.lvclass">)
            n402 = call-dynamic "Set ICP2-DO Changed bit.vi"("error in (no error)"=w1067, "Value"="Recirc Pump On - R6", "DO Channel"=ICP2-DO_Channel_Names."Recirc Pump On - R6", "IO in"=w1069) -> ("error out"=w1068:errorcluster)  [unwired: 6 in, 1 out]
          }
          event "Meniscus Pressure Reg PWR - R1": Value Change {
            n403 = event-data() -> ()  [unwired: 1 in, 6 out]
            n404 = Unbundle By Name(w1078) -> ("IO"=w1077:refnum<class "IO.lvclass">)
            n405 = call-dynamic "Set ICP1-DO Changed bit.vi"("error in (no error)"=w1075, "Value"="Meniscus Pressure Reg PWR - R1", "DO Channel"=ICP1-D0_Channel_Names."Meniscus Pressure Reg PWR - R1", "IO in"=w1077) -> ("error out"=w1076:errorcluster)  [unwired: 6 in, 1 out]
          }
          event "Meniscus Pressure Reg PWR - R2": Value Change {
            n406 = event-data() -> ()  [unwired: 1 in, 6 out]
            n407 = Unbundle By Name(w1086) -> ("IO"=w1085:refnum<class "IO.lvclass">)
            n408 = call-dynamic "Set ICP1-DO Changed bit.vi"("error in (no error)"=w1083, "Value"="Meniscus Pressure Reg PWR - R2", "DO Channel"=ICP1-D0_Channel_Names."Meniscus Pressure Reg PWR - R2", "IO in"=w1085) -> ("error out"=w1084:errorcluster)  [unwired: 6 in, 1 out]
          }
          event "Meniscus Pressure Reg PWR - R3": Value Change {
            n409 = event-data() -> ()  [unwired: 1 in, 6 out]
            n410 = Unbundle By Name(w1094) -> ("IO"=w1093:refnum<class "IO.lvclass">)
            n411 = call-dynamic "Set ICP1-DO Changed bit.vi"("error in (no error)"=w1091, "Value"="Meniscus Pressure Reg PWR - R3", "DO Channel"=ICP1-D0_Channel_Names."Meniscus Pressure Reg PWR - R3", "IO in"=w1093) -> ("error out"=w1092:errorcluster)  [unwired: 6 in, 1 out]
          }
          event "Meniscus Pressure Reg PWR - R4": Value Change {
            n412 = event-data() -> ()  [unwired: 1 in, 6 out]
            n413 = Unbundle By Name(w1102) -> ("IO"=w1101:refnum<class "IO.lvclass">)
            n414 = call-dynamic "Set ICP1-DO Changed bit.vi"("error in (no error)"=w1099, "Value"="Meniscus Pressure Reg PWR - R4", "DO Channel"=ICP1-D0_Channel_Names."Meniscus Pressure Reg PWR - R4", "IO in"=w1101) -> ("error out"=w1100:errorcluster)  [unwired: 6 in, 1 out]
          }
          event "Meniscus Pressure Reg PWR - R5": Value Change {
            n415 = event-data() -> ()  [unwired: 1 in, 6 out]
            n416 = Unbundle By Name(w1110) -> ("IO"=w1109:refnum<class "IO.lvclass">)
            n417 = call-dynamic "Set ICP1-DO Changed bit.vi"("error in (no error)"=w1107, "Value"="Meniscus Pressure Reg PWR - R5", "DO Channel"=ICP1-D0_Channel_Names."Meniscus Pressure Reg PWR - R5", "IO in"=w1109) -> ("error out"=w1108:errorcluster)  [unwired: 6 in, 1 out]
          }
          event "Meniscus Pressure Reg PWR - R6": Value Change {
            n418 = event-data() -> ()  [unwired: 1 in, 6 out]
            n419 = Unbundle By Name(w1118) -> ("IO"=w1117:refnum<class "IO.lvclass">)
            n420 = call-dynamic "Set ICP1-DO Changed bit.vi"("error in (no error)"=w1115, "Value"="Meniscus Pressure Reg PWR - R6", "DO Channel"=ICP1-D0_Channel_Names."Meniscus Pressure Reg PWR - R6", "IO in"=w1117) -> ("error out"=w1116:errorcluster)  [unwired: 6 in, 1 out]
          }
          event "ClearStageAlarm": Value Change {
            n421 = event-data() -> ()  [unwired: 1 in, 6 out]
            n422 = Unbundle By Name(w1146) -> ("Motor Controller"=w1124:refnum<class "Motor Controller.lvclass">, "IO"=w1137:refnum<class "IO.lvclass">)
            n423 = call "API_AbortStage.vi"("Wait (F)"=FALSE, "error in (no error)"=w1123, "Task ID"="AbortMotor", "Motor Controller in"=w1124) -> ("error out"=w1122:errorcluster)  [unwired: 5 in, 2 out]
            n424 = disable-structure shown="Enabled" {
              disable-tunnel: w1137 -> [w1159 w1163]
              disable-tunnel: [w1158 w1163] -> w1136
              disable-tunnel: [w1157 w1162] -> w1132
              disable-tunnel: w1122 -> [w1156 w1162]
              frame Enabled {
                n425 = call-dynamic "Set ICP1-DO Changed bit.vi"("error in (no error)"=w1156, "Value"=FALSE, "DO Channel"=ICP1-D0_Channel_Names."Servo ON", "IO in"=w1159) -> ("error out"=w1157:errorcluster, "IO out"=w1158:refnum<class "IO.lvclass">)  [unwired: 6 in]
              }
              frame Disabled {
              }
            }
            n426 = call <userlib>:"Wait (ms)__ogtk.vi"("error in (no error)"=w1132, "milliseconds to wait"=u32 100) -> ("error out"=w1130:errorcluster)  [unwired: 8 in, 1 out]
            n427 = local write "ClearStageAlarm"(FALSE ("ClearStageAlarm")) -> ()
            n428 = call-dynamic "Set ICP1-DO Changed bit.vi"("Wait (F)"=TRUE, "error in (no error)"=w1130, "Value"=TRUE, "DO Channel"=ICP1-D0_Channel_Names."Clear Stage Alarm", "IO in"=w1136) -> ("error out"=w1139:errorcluster, "IO out"=w1142:refnum<class "IO.lvclass">)  [unwired: 5 in]
            n429 = call <userlib>:"Wait (ms)__ogtk.vi"("error in (no error)"=w1139, "milliseconds to wait"=u32 300) -> ("error out"=w1141:errorcluster)  [unwired: 8 in, 1 out]
            n430 = call-dynamic "Set ICP1-DO Changed bit.vi"("error in (no error)"=w1141, "Value"=FALSE, "DO Channel"=ICP1-D0_Channel_Names."Clear Stage Alarm", "IO in"=w1142) -> ("error out"=w1134:errorcluster, "IO out"=w1135:refnum<class "IO.lvclass">)  [unwired: 6 in]
            n431 = call <userlib>:"Wait (ms)__ogtk.vi"("error in (no error)"=w1134, "milliseconds to wait"=u32 100) -> ("error out"=w1128:errorcluster)  [unwired: 8 in, 1 out]
            n432 = disable-structure shown="Enabled" {
              disable-tunnel: w1135 -> [w1152 _]
              disable-tunnel: w1128 -> [w1151 w1155]
              disable-tunnel: [w1150 w1155] -> w1133
              frame Enabled {
                n433 = call-dynamic "Set ICP1-DO Changed bit.vi"("error in (no error)"=w1151, "Value"=TRUE, "DO Channel"=ICP1-D0_Channel_Names."Servo ON", "IO in"=w1152) -> ("error out"=w1150:errorcluster)  [unwired: 6 in, 1 out]
              }
              frame Disabled {
              }
            }
          }
          event "Enable Disable With DO": Value Change {
            n434 = event-data() -> ("NewVal"=w1164:bool)  [unwired: 1 in, 5 out]
            n435 = Unbundle By Name(w1169) -> ("IO"=w1167:refnum<class "IO.lvclass">)
            n436 = call-dynamic "Set ICP1-DO Changed bit.vi"("error in (no error)"=w1165, "Value"=w1164, "DO Channel"=ICP1-D0_Channel_Names."Servo ON", "IO in"=w1167) -> ("error out"=w1166:errorcluster)  [unwired: 6 in, 1 out]
          }
          event "Purge Valve Open - R1": Value Change {
            n437 = event-data() -> ()  [unwired: 1 in, 6 out]
            n438 = Unbundle By Name(w1176) -> ("IO"=w1175:refnum<class "IO.lvclass">)
            n439 = call-dynamic "Set ICP1-DO Changed bit.vi"("error in (no error)"=w1173, "Value"="Purge Valve Open - R1", "DO Channel"=ICP1-D0_Channel_Names."Purge Valve Open - R1", "IO in"=w1175) -> ("error out"=w1174:errorcluster)  [unwired: 6 in, 1 out]
          }
          event "Purge Valve Open - R2": Value Change {
            n440 = event-data() -> ()  [unwired: 1 in, 6 out]
            n441 = Unbundle By Name(w1184) -> ("IO"=w1183:refnum<class "IO.lvclass">)
            n442 = call-dynamic "Set ICP1-DO Changed bit.vi"("error in (no error)"=w1181, "Value"="Purge Valve Open - R2", "DO Channel"=ICP1-D0_Channel_Names."Purge Valve Open - R2", "IO in"=w1183) -> ("error out"=w1182:errorcluster)  [unwired: 6 in, 1 out]
          }
          event "Purge Valve Open - R3": Value Change {
            n443 = event-data() -> ()  [unwired: 1 in, 6 out]
            n444 = Unbundle By Name(w1192) -> ("IO"=w1191:refnum<class "IO.lvclass">)
            n445 = call-dynamic "Set ICP1-DO Changed bit.vi"("error in (no error)"=w1189, "Value"="Purge Valve Open - R3", "DO Channel"=ICP1-D0_Channel_Names."Purge Valve Open - R3", "IO in"=w1191) -> ("error out"=w1190:errorcluster)  [unwired: 6 in, 1 out]
          }
          event "Purge Valve Open - R4": Value Change {
            n446 = event-data() -> ()  [unwired: 1 in, 6 out]
            n447 = Unbundle By Name(w1200) -> ("IO"=w1199:refnum<class "IO.lvclass">)
            n448 = call-dynamic "Set ICP1-DO Changed bit.vi"("error in (no error)"=w1197, "Value"="Purge Valve Open - R4", "DO Channel"=ICP1-D0_Channel_Names."Purge Valve Open - R4", "IO in"=w1199) -> ("error out"=w1198:errorcluster)  [unwired: 6 in, 1 out]
          }
          event "Purge Valve Open - R5": Value Change {
            n449 = event-data() -> ()  [unwired: 1 in, 6 out]
            n450 = Unbundle By Name(w1208) -> ("IO"=w1207:refnum<class "IO.lvclass">)
            n451 = call-dynamic "Set ICP1-DO Changed bit.vi"("error in (no error)"=w1205, "Value"="Purge Valve Open - R5", "DO Channel"=ICP1-D0_Channel_Names."Purge Valve Open - R5", "IO in"=w1207) -> ("error out"=w1206:errorcluster)  [unwired: 6 in, 1 out]
          }
          event "Purge Valve Open - R6": Value Change {
            n452 = event-data() -> ()  [unwired: 1 in, 6 out]
            n453 = Unbundle By Name(w1216) -> ("IO"=w1215:refnum<class "IO.lvclass">)
            n454 = call-dynamic "Set ICP1-DO Changed bit.vi"("error in (no error)"=w1213, "Value"="Purge Valve Open - R6", "DO Channel"=ICP1-D0_Channel_Names."Purge Valve Open - R6", "IO in"=w1215) -> ("error out"=w1214:errorcluster)  [unwired: 6 in, 1 out]
          }
          event "Meniscus Pressure Set - R1-Set": Value Change {
            n455 = event-data() -> ()  [unwired: 1 in, 6 out]
            n456 = Unbundle By Name(w1225) -> ("IO"=w1224:refnum<class "IO.lvclass">)
            n457 = call-dynamic "Set ICP1-AO Changed Value.vi"("error in (no error)"=w1222, "Value"="Meniscus Pressure Set - R1", "AO Channel"=ICP1-AO_Channel_Names."Meniscus Pressure Set - R1", "IO in"=w1224) -> ("error out"=w1223:errorcluster)  [unwired: 6 in, 1 out]
          }
          event "Meniscus Pressure Set - R2-Set": Value Change {
            n458 = event-data() -> ()  [unwired: 1 in, 6 out]
            n459 = Unbundle By Name(w1233) -> ("IO"=w1232:refnum<class "IO.lvclass">)
            n460 = call-dynamic "Set ICP1-AO Changed Value.vi"("error in (no error)"=w1230, "Value"="Meniscus Pressure Set - R2", "AO Channel"=ICP1-AO_Channel_Names."Meniscus Pressure Set - R2", "IO in"=w1232) -> ("error out"=w1231:errorcluster)  [unwired: 6 in, 1 out]
          }
          event "Meniscus Pressure Set - R3-Set": Value Change {
            n461 = event-data() -> ()  [unwired: 1 in, 6 out]
            n462 = Unbundle By Name(w1241) -> ("IO"=w1240:refnum<class "IO.lvclass">)
            n463 = call-dynamic "Set ICP1-AO Changed Value.vi"("error in (no error)"=w1238, "Value"="Meniscus Pressure Set - R3", "AO Channel"=ICP1-AO_Channel_Names."Meniscus Pressure Set - R3", "IO in"=w1240) -> ("error out"=w1239:errorcluster)  [unwired: 6 in, 1 out]
          }
          event "Meniscus Pressure Set - R4-Set": Value Change {
            n464 = event-data() -> ()  [unwired: 1 in, 6 out]
            n465 = Unbundle By Name(w1249) -> ("IO"=w1248:refnum<class "IO.lvclass">)
            n466 = call-dynamic "Set ICP1-AO Changed Value.vi"("error in (no error)"=w1246, "Value"="Meniscus Pressure Set - R4", "AO Channel"=ICP1-AO_Channel_Names."Meniscus Pressure Set - R4", "IO in"=w1248) -> ("error out"=w1247:errorcluster)  [unwired: 6 in, 1 out]
          }
          event "Meniscus Pressure Set - R5-Set": Value Change {
            n467 = event-data() -> ()  [unwired: 1 in, 6 out]
            n468 = Unbundle By Name(w1257) -> ("IO"=w1256:refnum<class "IO.lvclass">)
            n469 = call-dynamic "Set ICP1-AO Changed Value.vi"("error in (no error)"=w1254, "Value"="Meniscus Pressure Set - R5", "AO Channel"=ICP1-AO_Channel_Names."Meniscus Pressure Set - R5", "IO in"=w1256) -> ("error out"=w1255:errorcluster)  [unwired: 6 in, 1 out]
          }
          event "Meniscus Pressure Set - R6-Set": Value Change {
            n470 = event-data() -> ()  [unwired: 1 in, 6 out]
            n471 = Unbundle By Name(w1265) -> ("IO"=w1264:refnum<class "IO.lvclass">)
            n472 = call-dynamic "Set ICP1-AO Changed Value.vi"("error in (no error)"=w1262, "Value"="Meniscus Pressure Set - R6", "AO Channel"=ICP1-AO_Channel_Names."Meniscus Pressure Set - R6", "IO in"=w1264) -> ("error out"=w1263:errorcluster)  [unwired: 6 in, 1 out]
          }
          event "Recirc Pump Flow Set - R1 Set": Value Change {
            n473 = event-data() -> ()  [unwired: 1 in, 6 out]
            n474 = Unbundle By Name(w1273) -> ("IO"=w1272:refnum<class "IO.lvclass">)
            n475 = call-dynamic "Set ICP2-AO Changed Value.vi"("error in (no error)"=w1270, "Value"="Recirc Pump Flow Set - R1", "AO Channel"=ICP2-AO_Channel_Names."Recirc Pump Flow Set - R1", "IO in"=w1272) -> ("error out"=w1271:errorcluster)  [unwired: 6 in, 1 out]
          }
          event "Recirc Pump Flow Set - R2 Set": Value Change {
            n476 = event-data() -> ()  [unwired: 1 in, 6 out]
            n477 = Unbundle By Name(w1281) -> ("IO"=w1280:refnum<class "IO.lvclass">)
            n478 = call-dynamic "Set ICP2-AO Changed Value.vi"("error in (no error)"=w1278, "Value"="Recirc Pump Flow Set - R2", "AO Channel"=ICP2-AO_Channel_Names."Recirc Pump Flow Set - R2", "IO in"=w1280) -> ("error out"=w1279:errorcluster)  [unwired: 6 in, 1 out]
          }
          event "Recirc Pump Flow Set - R3 Set": Value Change {
            n479 = event-data() -> ()  [unwired: 1 in, 6 out]
            n480 = Unbundle By Name(w1289) -> ("IO"=w1288:refnum<class "IO.lvclass">)
            n481 = call-dynamic "Set ICP2-AO Changed Value.vi"("error in (no error)"=w1286, "Value"="Recirc Pump Flow Set - R3", "AO Channel"=ICP2-AO_Channel_Names."Recirc Pump Flow Set - R3", "IO in"=w1288) -> ("error out"=w1287:errorcluster)  [unwired: 6 in, 1 out]
          }
          event "Recirc Pump Flow Set - R4 Set": Value Change {
            n482 = event-data() -> ()  [unwired: 1 in, 6 out]
            n483 = Unbundle By Name(w1297) -> ("IO"=w1296:refnum<class "IO.lvclass">)
            n484 = call-dynamic "Set ICP2-AO Changed Value.vi"("error in (no error)"=w1294, "Value"="Recirc Pump Flow Set - R4", "AO Channel"=ICP2-AO_Channel_Names."Recirc Pump Flow Set - R4", "IO in"=w1296) -> ("error out"=w1295:errorcluster)  [unwired: 6 in, 1 out]
          }
          event "Recirc Pump Flow Set - R5 Set": Value Change {
            n485 = event-data() -> ()  [unwired: 1 in, 6 out]
            n486 = Unbundle By Name(w1305) -> ("IO"=w1304:refnum<class "IO.lvclass">)
            n487 = call-dynamic "Set ICP2-AO Changed Value.vi"("error in (no error)"=w1302, "Value"="Recirc Pump Flow Set - R5", "AO Channel"=ICP2-AO_Channel_Names."Recirc Pump Flow Set - R5", "IO in"=w1304) -> ("error out"=w1303:errorcluster)  [unwired: 6 in, 1 out]
          }
          event "Recirc Pump Flow Set - R6 Set": Value Change {
            n488 = event-data() -> ()  [unwired: 1 in, 6 out]
            n489 = Unbundle By Name(w1313) -> ("IO"=w1312:refnum<class "IO.lvclass">)
            n490 = call-dynamic "Set ICP2-AO Changed Value.vi"("error in (no error)"=w1310, "Value"="Recirc Pump Flow Set - R6", "AO Channel"=ICP2-AO_Channel_Names."Recirc Pump Flow Set - R6", "IO in"=w1312) -> ("error out"=w1311:errorcluster)  [unwired: 6 in, 1 out]
          }
        }
      }
      frame "---------- Core ----------" {
        # "Do not put any code in this frame.\n(it is a separator no-op)"
        n491 = call <vilib>:"Add State(s) to Queue__JKI_lib_State_Machine.vi"("State(s) in (\"\")"=w1321) -> ("States Out"=w1320:string)  [unwired: 14 in]
      }
      frame Default {
        w1333 = 42 items=["No error", "Argument error", "Memory is full", "Out of zone", "End of file", "File already open", "Generic file I/O error", "File not found", "File permission error", "Disk is full", "Duplicate path", "Too many files open", "System feature not enabled", "Resource file not found", "Cannot add resource", "Resource not found", "Image not found", "Image memory error", "Pen does not exist", "Config type invalid", "Config token not found", "Config parse error", "Config memory error", "Bad external code format", "Bad external code offset", "External code not present", "Null window", "Destroy window error", "Null menu", "Print aborted", "Bad print record", "Print driver error", "Windows error during printing", "Memory error during printing", "Print dialog error", "Generic print error", "Invalid device refnum", "Device not found", "Device parameter error", "Device unit error", "Cannot open device", "Device call aborted", "Generic error", "Cancelled by user", "Object ID too low", "Object ID too high", "Object not in heap", "Unknown heap", "Unknown object (invalid DefProc)", "Unknown object (DefProc not in table)", "Message out of range", "Invalid (null) method", "Unknown message", "Manager call not supported", "Bad address", "Network operation in progress", "Network operation timed out", "Connection is busy", "Network attribute not supported", "Network error", "Address in use", "System out of memory", "Connection aborted", "Connection refused", "Not connected", "Already connected", "Connection closed", "Initialization error (interapplication manager)", "Bad occurrence", "Wait on unbound occurrence handler", "Occurrence queue overflow", "Datalog type conflict", "Unused", "Unrecognized type (interapplication manager)", "Memory corrupt", "Failed to make temporary DLL", "Old CIN version", "Drag socket not found", "Failed to load drop-object", "Failed to register OLE object", "Failed to release OLE object", "Format specifier type mismatch", "Unknown format specifier", "Too few format specifiers", "Too many format specifiers", "Scan failed", "Newer CIN version", "Error converting to variant", "Runtime menu error", "Password tampered", "Variant attribute not found", "Incompatible variant data type", "Event data is not available", "Event Store is not present", "Occurrence is not found", "Event Queue is not created", "Event info is not available", "Refnum passed is NULL", "Error retrieving Class GUID", "Error retrieving CoClass GUID", "Error retrieving TypeLib GUID.", "Bad built application magic bytes.", "Specific driver is different from the specific driver associated with the Logical Name.", "There is no session opened to the class driver.", "Max Error", "MAX - Error with config objects", "MAX - Error loading configuration", "MAX - Group not supported"]
        # "Current State"
        # "Do not delete, rename, or modify this frame.\n(this is used to capture unhandled states and typos)"
        # "Handle mistyped state name (developer tool)"
        n492 = Format Into String(format string="Software Exception: Unhandled State \"%s\"." ("message"), error in=w1329, w1324) -> (resulting string=w1332:string, error out=w1331:errorcluster)  [unwired: 1 in]
        n493 = call <vilib>:"Error Cluster From Error Code.vi"("show call chain? (False)"=TRUE, "error in (no error)"=w1331, "error message (\"\")"=w1332, "error code (0)"=w1333) -> ("error out"=w1330:errorcluster)  [unwired: 5 in]
        n494 = call <vilib>:"Add State(s) to Queue__JKI_lib_State_Machine.vi"("State(s) in (\"\")"=w1328) -> ("States Out"=w1327:string)  [unwired: 14 in]
      }
      frame "Initialize Core Data" {
        # "Do not delete, rename, or modify this frame.\n(this is used to determine panel behavior on exit)"
        # "originally closed?"
        # "exe?"
        # "If panel starts closed or is an EXE, then close it when we exit"
        n495 = property class="VI"() -> ("Front Panel.Open"=w1344:bool)  [unwired: 2 in, 2 out]
        n496 = property class="App"() -> ("App.Kind"=w1343:T16)  [unwired: 2 in, 2 out]
        n497 = control-ref of="Current VI Reference"() -> (w1337:refnum<vi>)
        n498 = Not(x=w1344) -> (.not. x?=w1341:bool)
        n499 = Equal?(x=w1343, y=T16."Run Time System" ("Application:Kind")) -> (x = y?=w1340:bool)
        n500 = Or(x=w1341, y=w1340) -> (x .or. y?=w1338:bool)
        n501 = Bundle By Name(cluster=w1339, "Core.Current VI Reference"=w1337, "Core.Close Panel on Exit?"=w1338) -> (w1346:T36)
        n502 = call <vilib>:"Add State(s) to Queue__JKI_lib_State_Machine.vi"("State(s) in (\"\")"=w1348) -> ("States Out"=w1347:string)  [unwired: 14 in]
      }
      frame "Error Handler" {
        # "Unhandled Error -- Display it"
        # "Handle any errors here.\nYou can also output any states to clean-up after errors occur"
        # "Clear error"
        n503 = call <vilib>:"General Error Handler.vi"("error in (no error)"=w1352) -> ()  [unwired: 10 in, 5 out]
        n504 = call <vilib>:"Add State(s) to Queue__JKI_lib_State_Machine.vi"("State(s) in Front (\"\")"="/* Post Error States", "State(s) in (\"\")"=w1356) -> ("States Out"=w1355:string)  [unwired: 13 in]
      }
      frame "Exit" {
        # "Do not put any code in this frame.\n(No errors that occur here will be handled.)"
        n505 = call <vilib>:"Add State(s) to Queue__JKI_lib_State_Machine.vi"("State(s) in (\"\")"=w1363) -> ("States Out"=w1362:string)  [unwired: 14 in]
      }
      frame "---------- Data ----------" {
        # "Do not put any code in this frame.\n(It is a separator no-op. You can make a copy of this frame to create a new Data frame)"
        n506 = call <vilib>:"Add State(s) to Queue__JKI_lib_State_Machine.vi"("State(s) in (\"\")"=w1369) -> ("States Out"=w1368:string)  [unwired: 14 in]
      }
      frame "Data: Initialize" {
        (unwired) T26 {"Motion Controller"={"Motor IP Addresss"="", "Current Position"=0, "Pulse_Per_mm"=0, "PrePrint"=[], "Load Position_mm"=0, "Laminate Position_mm"=0}, "IO Config"={"DAQDevices"=[], "DI Channels"=[], "DO Channels"=[], "Material Names"=[], "AI Channels"=[], "AO Channels"=[]}, "PrinterConfiguration"={"IPAddress"="", "Move Stage on RTP Command?"=FALSE, "Stage Move Position"="", "PH1-Prime Path"=path "", "PH2-Prime Path"=path "", "PH3-Prime Path"=path "", "PH4-Prime Path"=path "", "PH5-Prime Path"=path "", "PH6-Prime Path"=path "", "PrintScriptsFolder"=path "", "PurgeScriptsFolder"=path "", "StageScriptsFolder"=path "", "PH1-HeatOn Path"=path "", "PH2-HeatOn Path"=path "", "PH3-HeatOn Path"=path "", "PH4-HeatOn Path"=path "", "PH5-HeatOn Path"=path "", "PH6-HeatOn Path"=path "", "PH1-HeatOff Path"=path "", "PH2-HeatOff Path"=path "", "PH3-HeatOff Path"=path "", "PH4-HeatOff Path"=path "", "PH5-HeatOff Path"=path "", "PH6-HeatOff Path"=path ""}, "DAQ Settings"={"Simulate DAQ"=FALSE, "DI Settings"=[], "AI Settings"=[], "Relay IONames"=[], "AO IONames"=[], "AO NChan SingleTask"=FALSE}} ("Digilens Config")
        w1371 = API_Command_Enum."Execute Printer Commands"  # API Command
        w1372 = T2 {"GIS File Path"=path "", "Duration (s)"=0.1, "No. of Repeats"=1}  # Pre Purge Parameters
        w1373 = ICP1-D0_Channel_Names."None"  # Purge\PrePurge Channel Name
        w1382 = refnum<class "Motor Controller.lvclass"> refnum  # Motor Controller
        w1385 = refnum<class "GIS Printer.lvclass"> refnum  # GIS Printer
        w1387 = refnum<class "IO.lvclass"> refnum  # IO
        w1392 = T37 {"Current VI Reference"=refnum, "Close Panel on Exit?"=FALSE}  # Core
        n507 = property class="TopLevel.lvclass"(reference=w1391) -> (reference out=w1379:refnum<class "TopLevel.lvclass">, "Methods:Accessors:IO"=w1389:refnum<class "IO.lvclass">, "Methods:Accessors:GIS Printer"=w1390:refnum<class "GIS Printer.lvclass">, "Methods:Accessors:Motor Controller"=w1384:refnum<class "Motor Controller.lvclass">, "Methods:Accessors:Digilens Config"=w1374:T26)  [unwired: 1 in, 1 out]
        n508 = call-dynamic "GetEvents_TopLevel.vi"("error in (no error)"=w1376, "TopLevel in"=w1379) -> ("error out"=w1377:errorcluster, "UserEvents"=w1378:T38, "TopLevel out"=w1370:refnum<class "TopLevel.lvclass">)  [unwired: 7 in]
        n509 = Unbundle By Name(w1378) -> ("Exit Event"=w1375:refnum<user-event>)
        n510 = Coerce To Type(0:w1389, 1:w1387) -> (2:w1388:refnum<class "IO.lvclass">)
        n511 = Coerce To Type(0:w1390, 1:w1385) -> (2:w1386:refnum<class "GIS Printer.lvclass">)
        n512 = Coerce To Type(0:w1384, 1:w1382) -> (2:w1383:refnum<class "Motor Controller.lvclass">)
        n513 = Bundle("Core"=w1392, "IO"=w1388, "GIS Printer"=w1386, "Motor Controller"=w1383, "Methods:Accessors:Digilens Config"=w1374, "Status"=T17 {"Motor Controller Config Data"={"Motor IP Addresss"="", "Current Position"=0, "Pulse_Per_mm"=0, "PrePrint"=[], "Load Position_mm"=0, "Laminate Position_mm"=0}, "Motor Controller Data"={"Enabled?"=FALSE}, "Stage Move"={"Current Step"="", "Move Data"=[]}, "Stage Busy?"=FALSE}, "Exit Event"=w1375, "Purge\\PrePurge Channel Name"=w1373, "Pre Purge Parameters"=w1372, "API Command"=w1371, "TopLevel out"=w1370) -> (w1393:T36)  [unwired: 1 in]
        n514 = call <vilib>:"Add State(s) to Queue__JKI_lib_State_Machine.vi"("State(s) in (\"\")"=w1395) -> ("States Out"=w1394:string)  [unwired: 14 in]
      }
      frame "Data: Cleanup" {
        # "Cleanup any data and references, here.\n(this is called automatically, by the Macro: Exit)"
        n515 = Unbundle By Name(w1398) -> ("Core.Current VI Reference"=w1401:refnum<vi>)
        n516 = Close Reference(reference=w1401, error in (no error)=w1400) -> (error out=w1399:errorcluster)
        n517 = call <vilib>:"Add State(s) to Queue__JKI_lib_State_Machine.vi"("State(s) in (\"\")"=w1403) -> ("States Out"=w1402:string)  [unwired: 14 in]
      }
      frame "---------- UI ----------" {
        n518 = call <vilib>:"Add State(s) to Queue__JKI_lib_State_Machine.vi"("State(s) in (\"\")"=w1409) -> ("States Out"=w1408:string)  [unwired: 14 in]
      }
      frame "UI: SetUIControlsState" {
        n519 = Unbundle By Name(w1426) -> ()  [unwired: 1 out]
        n520 = control-ref of="This VI"() -> (w1425:refnum<vi>)
        n521 = To Lower Case(string=w1423) -> (all lower case string=w1421:string)
        n522 = property class="VI"(reference=w1425) -> ("Panel"=w1424:refnum<vi>)  [unwired: 1 in, 2 out]
        n523 = Equal?(x=w1421, y="enable") -> (x = y?=w1420:bool)
        n524 = property class="Pnl"(reference=w1424) -> ("Controls[]"=w1411:refnum<vi>[])  [unwired: 1 in, 2 out]
        n525 = Index Array(array=w1411) -> (element=w1415:refnum<vi>)  [unwired: 1 in]
        n526 = Select(t=T22."Enabled" ("Disabled"), s=w1420, f=T22."Disabled and Grayed Out" ("Disabled")) -> (s? t:f=w1417:T22)
        n527 = Type Cast(type=refnum<vi> refnum ("element"), x=w1415) -> (*(type *) &x=w1413:refnum<vi>)
        n528 = property class="TabCtl"(reference=w1413) -> ("Pages"=w1412:refnum<vi>[])  [unwired: 1 in, 2 out]
        n529 = for {
          tunnel: w1412 -> [w1433] mode=indexing
          tunnel: [w1432] -> w1410 mode=concatenating
          n530 = property class="Page"(reference=w1433) -> ("Z-Order:Controls[]"=w1432:refnum<vi>[])  [unwired: 1 in, 2 out]
        }
        n531 = for {
          tunnel: w1410 -> [w1444] mode=indexing
          tunnel: w1417 -> [w1439]
          tunnel: [w1435] -> w1416 mode=indexing
          n532 = property class="Ctl"(reference=w1444) -> (reference out=w1442:refnum<vi>, "Label.Text"=w1435:string)  [unwired: 1 in, 1 out]
          n533 = Equal?(x=w1435, y="IdlePrint") -> (x = y?=w1436:bool)
          n534 = Equal?(x=w1435, y="Abort") -> (x = y?=w1437:bool)
          n535 = Or(x=w1436, y=w1437) -> (x .or. y?=w1434:bool)
          n536 = Select(t=T22."Enabled" ("Disabled"), s=w1434, f=w1439) -> (s? t:f=w1440:T22)
          n537 = property class="Ctl"(reference=w1442, "DisabledEnum"=w1440) -> ()  [unwired: 1 in, 2 out]
        }
        n538 = flat-sequence {
          tunnel: w1416 -> [_]
          frame #0 {
          }
        }
        n539 = call <vilib>:"Add State(s) to Queue__JKI_lib_State_Machine.vi"("State(s) in (\"\")"=w1431) -> ("States Out"=w1430:string)  [unwired: 14 in]
      }
      frame "UI: Initialize" {
        n540 = Unbundle By Name(w1448) -> ("Methods:Accessors:Digilens Config.IO Config.Material Names"=w1449:string[], "Core.Current VI Reference"=w1454:refnum<vi>)
        n541 = Unbundle By Name(w1448) -> ("Methods:Accessors:Digilens Config.PrinterConfiguration.PrintScriptsFolder"=w1447:path, "Methods:Accessors:Digilens Config.PrinterConfiguration.StageScriptsFolder"=w1446:path, "Methods:Accessors:Digilens Config.PrinterConfiguration.PurgeScriptsFolder"=w1445:path)
        n542 = property on="Head 1 Material" class="Ring (strict)"("Strings []"=w1449) -> ()  [unwired: 2 in, 2 out]
        n543 = property on="Head 2 Material" class="Ring (strict)"("Strings []"=w1449) -> ()  [unwired: 2 in, 2 out]
        n544 = property on="Head 3 Material" class="Ring (strict)"("Strings []"=w1449) -> ()  [unwired: 2 in, 2 out]
        n545 = property on="Head 4 Material" class="Ring (strict)"("Strings []"=w1449) -> ()  [unwired: 2 in, 2 out]
        n546 = property on="Head 5 Material" class="Ring (strict)"("Strings []"=w1449) -> ()  [unwired: 2 in, 2 out]
        n547 = property on="Head 6 Material" class="Ring (strict)"("Strings []"=w1449) -> ()  [unwired: 2 in, 2 out]
        n548 = call <userlib>:"Fit VI window to Largest Dec__ogtk.vi"("error in (no error)"=w1452, "VI Ref (calling VI)"=w1454) -> ("error out"=w1453:errorcluster)  [unwired: 4 in, 1 out]
        n549 = property on="Command File Path" class="Path"("StartPath"=w1447) -> ()  [unwired: 2 in, 2 out]
        n550 = property on="Stage Recipe XML File Path" class="Path"("StartPath"=w1446) -> ()  [unwired: 2 in, 2 out]
        n551 = property on="GIS File Path" class="Path"("StartPath"=w1445) -> ()  [unwired: 2 in, 2 out]
        n552 = property on="GIS File Path" class="Path"("StartPath"=w1445) -> ()  [unwired: 2 in, 2 out]
        n553 = property on="GIS File Path" class="Path"("StartPath"=w1445) -> ()  [unwired: 2 in, 2 out]
        n554 = property on="GIS File Path" class="Path"("StartPath"=w1445) -> ()  [unwired: 2 in, 2 out]
        n555 = property on="GIS File Path" class="Path"("StartPath"=w1445) -> ()  [unwired: 2 in, 2 out]
        n556 = property on="GIS File Path" class="Path"("StartPath"=w1445) -> ()  [unwired: 2 in, 2 out]
        n557 = local write "Stage Recipe XML File Path"(path "" ("Recipe XML File Path")) -> ()
        n558 = property on="TCP Commands & Responses" class="MCListbox (strict)"("ItemNames"=string[][] [] ("Item Names")) -> ()  [unwired: 2 in, 2 out]
      }
      frame "UI: Cursor Set" {
        # "Argument"
        # "Set and Unset Cursor Busy.\n(Usage: \"UI: Cursor Set >> Busy|Idle\")"
        n559 = case shown="\"Idle\", Default" w1460 {
          tunnel: w1462 -> [w1467 w1469]
          tunnel: [w1466 w1468] -> w1461
          frame "Idle", Default {
            n560 = call <vilib>:"Unset Busy.vi"("error in (no error)"=w1467) -> ("error out"=w1466:errorcluster)  [unwired: 10 in]
          }
          frame "Busy" {
            n561 = call <vilib>:"Set Busy.vi"("error in (no error)"=w1469) -> ("error out"=w1468:errorcluster)  [unwired: 9 in, 1 out]
          }
        }
        n562 = call <vilib>:"Add State(s) to Queue__JKI_lib_State_Machine.vi"("State(s) in (\"\")"=w1465) -> ("States Out"=w1464:string)  [unwired: 14 in]
      }
      frame "UI: Front Panel State" {
        # "Argument"
        # "Set Front Panel Open or Closed\n(Usage: \"UI: Front Panel State >> Open|Close\")"
        n563 = Unbundle By Name(w1474) -> ("Core.Current VI Reference"=w1473:refnum<vi>)
        n564 = case shown="\"Open\", Default" w1472 {
          tunnel: w1476 -> [w1482 w1495]
          tunnel: [w1484 w1496] -> w1475
          tunnel: w1473 -> [w1483 w1493]
          frame "Open", Default {
            n565 = property class="VI"(reference=w1483, error in=w1482) -> (reference out=w1480:refnum<vi>, error out=w1481:errorcluster, "Front Panel.Open"=w1479:bool)
            n566 = case shown="False" w1479 {
              tunnel: [w1487 w1490] -> w1484
              tunnel: w1481 -> [w1486 w1490]
              tunnel: w1480 -> [w1485 _]
              frame False {
                n567 = invoke class="VI" method="FP.Open"(reference=w1485, error in=w1486, "Activate"=TRUE, "State"=T23."Standard") -> (error out=w1487:errorcluster)  [unwired: 1 in, 4 out]
              }
              frame True {
              }
            }
          }
          frame "Close" {
            n568 = property class="VI"(reference=w1493, error in=w1495) -> (reference out=w1492:refnum<vi>, error out=w1494:errorcluster, "Front Panel.Open"=w1491:bool)
            n569 = case shown="True" w1491 {
              tunnel: [w1497 w1500] -> w1496
              tunnel: w1494 -> [w1497 w1499]
              tunnel: w1492 -> [_ w1498]
              frame False {
              }
              frame True {
                n570 = invoke class="VI" method="FP.Close"(reference=w1498, error in=w1499) -> (error out=w1500:errorcluster)  [unwired: 1 in, 2 out]
              }
            }
          }
        }
        n571 = call <vilib>:"Add State(s) to Queue__JKI_lib_State_Machine.vi"("State(s) in (\"\")"=w1478) -> ("States Out"=w1477:string)  [unwired: 14 in]
      }
      frame "UI: Update Stage Busy" {
        n572 = Unbundle By Name(w1512) -> ("GIS Printer"=w1511:refnum<class "GIS Printer.lvclass">, "Motor Controller"=w1510:refnum<class "Motor Controller.lvclass">, "TopLevel out"=w1504:refnum<class "TopLevel.lvclass">)
        n573 = call-dynamic "GetStatus_TopLevel_Busy.vi"("error in (no error)"=w1502, "TopLevel in"=w1504) -> ("error out"=w1503:errorcluster, "Busy"=w1501:bool)  [unwired: 7 in, 1 out]
        n574 = call-dynamic "GetPrinterBusy_Status_GIS Printer.vi"("error in (no error)"=w1503, "TopLevel in"=w1511) -> ("error out"=w1509:errorcluster, "Printer Busy?"=w1507:bool)  [unwired: 7 in, 1 out]
        n575 = call "GetStageBusy_Status_MotorController.vi"("error in (no error)"=w1509, "Motor Controller in"=w1510) -> ("error out"=w1508:errorcluster, "Stage Busy?"=w1506:bool)  [unwired: 7 in, 1 out]
        n576 = Compound Arithmetic op=OR(w1507, w1506, w1501) -> (→"Stage Busy Printer" →"Stage Busy (Stage)" →"Stage Busy (Moves)":bool)
      }
      frame "---------- Macro ----------" {
        # "Do not put any code in this frame.\n(It is a separator no-op. You can make a copy of this frame to create a new Macro frame)"
        n577 = call <vilib>:"Add State(s) to Queue__JKI_lib_State_Machine.vi"("State(s) in (\"\")"=w1521) -> ("States Out"=w1520:string)  [unwired: 14 in]
      }
      frame "Macro: Initialize" {
        # "Initialization Macro\n(This is called once, when the VI starts)"
        n578 = call <vilib>:"Add State(s) to Queue__JKI_lib_State_Machine.vi"("State(s) in Front (\"\")"="Data: Initialize\nInitialize Core Data\nInit: Set Jog Speed\nUI: Initialize\nUI: SetUIControlsState>>enable\nEvents: Register Events\nUI: Update Stage Busy\nInit: Read ICP1-DO\nInit: Read ICP2-DO\nInit: Read ICP1-AO\nInit: Read ICP2-AO\n/*DI: Get ICP2 DI Status\n/*DO: Set ICP1-DO Status in UI\n/*DO: Set ICP2-DO Status in UI\n/*AI: Get ICP1 AI Status\n/*AO: Set ICP1-AO Status in UI\n/*AO: Set ICP2-AO Status in UI\nInitialize DO Devices\nUI: Front Panel State >> Open", "State(s) in (\"\")"=w1528) -> ("States Out"=w1527:string)  [unwired: 13 in]
      }
      frame "Macro: Exit" {
        # "Exit Macro\n(This is called once, when the VI exits)"
        n579 = Unbundle By Name(w1532) -> ("Core.Close Panel on Exit?"=w1542:bool)  [unwired: 1 out]
        n580 = call <vilib>:"Clear Errors.vi"("error in (no error)"=w1530) -> ("error out"=w1529:errorcluster)  [unwired: 5 in, 1 out]
        n581 = Unbundle By Name(w1532) -> ("Exit Event"=w1534:refnum<user-event>)
        n582 = Generate User Event(user event=w1534, event data cluster="Exit" ("event data"), error in=w1529) -> (error out=w1531:errorcluster)  [unwired: 1 in, 1 out]
        n583 = Select(t="UI: Front Panel State >> Close", s=w1542, f="") -> (s? t:f=w1539:string)
        n584 = call <vilib>:"Add State(s) to Queue__JKI_lib_State_Machine.vi"("State(s) in (\"\")"=w1539, "State(s) at Back (\"\")"="UI: SetUIControlsState>>enable\nData: Cleanup\nEvents: Unregister Events\nExit") -> ("States Out"=w1537:string)  [unwired: 13 in]
        n585 = call <vilib>:"Add State(s) to Queue__JKI_lib_State_Machine.vi"("State(s) in Front (\"\")"=w1537, "State(s) in (\"\")"=w1544) -> ("States Out"=w1543:string)  [unwired: 13 in]
      }
      frame "----------Events ----------" {
        # "Template Separator\n(You can make a copy of, or modify, this frame)"
      }
      frame "Events: Register Events" {
        w1551 = refnum<user-event> refnum  # TopLevel StatusChanged Event
        w1561 = refnum<user-event> refnum  # IO Status Changed Event
        w1557 = refnum<user-event> refnum  # Motor Status Changed Event
        n586 = Unbundle By Name(w1572) -> ("Motor Controller"=w1574:refnum<class "Motor Controller.lvclass">, "IO"=w1568:refnum<class "IO.lvclass">, "GIS Printer"=w1566:refnum<class "GIS Printer.lvclass">, "TopLevel out"=w1556:refnum<class "TopLevel.lvclass">)
        n587 = call-dynamic "GetEvents_Motor Controller.vi"("error in (no error)"=w1571, "TopLevel in"=w1574) -> ("error out"=w1567:errorcluster, "UserEvents"=w1573:T39)  [unwired: 7 in, 1 out]
        n588 = call-dynamic "GetEvents_IO.vi"("error in (no error)"=w1567, "TopLevel in"=w1568) -> ("error out"=w1565:errorcluster, "UserEvents"=w1569:T40)  [unwired: 7 in, 1 out]
        n589 = Unbundle By Name(w1573) -> ("Status Changed Event"=w1558:refnum<user-event>)
        n590 = Unbundle By Name(w1569) -> ("Status Changed Event"=w1560:refnum<user-event>)
        n591 = call-dynamic "GetEvents_GIS Printer.vi"("error in (no error)"=w1565, "TopLevel in"=w1566) -> ("error out"=w1555:errorcluster, "UserEvents"=w1564:T41)  [unwired: 7 in, 1 out]
        n592 = Unbundle By Name(w1564) -> ("Status Changed Event"=w1563:refnum<user-event>)
        n593 = Coerce To Type(0:w1558, 1:w1557) -> (2:w1562:refnum<user-event>)
        n594 = call-dynamic "GetEvents_TopLevel.vi"("error in (no error)"=w1555, "TopLevel in"=w1556) -> ("error out"=w1554:errorcluster, "UserEvents"=w1553:T38)  [unwired: 7 in, 1 out]
        n595 = Coerce To Type(0:w1560, 1:w1561) -> (2:w1559:refnum<user-event>)
        n596 = Unbundle By Name(w1553) -> ("StatusChanged"=w1552:refnum<user-event>)
        n597 = Coerce To Type(0:w1552, 1:w1551) -> (2:w1550:refnum<user-event>)
        n598 = register-events(w1562, w1559, w1563, w1550) -> (reference out=w1570:refnum<event-registration>)  [unwired: 2 in, 1 out]
      }
      frame "Events: Unregister Events" {
        n599 = Unregister For Events(event registration refnum=w1579, error in=w1577) -> (error out=w1578:errorcluster)
      }
      frame "---------Init------------" {
      }
      frame "Init: Set Jog Speed" {
        n600 = Unbundle By Name(w1589) -> ("Motor Controller"=w1593:refnum<class "Motor Controller.lvclass">)
        n601 = Bundle By Name(cluster=T3 {"Motor Controller Parameter"=enum."Write Speed", "value"=0} ("SetExplicitMessage API Data"), "Motor Controller Parameter"=Motor_Controller_Parameter-Set."Jog Speed", "value"=0) -> (w1599:T3)
        n602 = Bundle By Name(cluster=T6 {"Command"=enum."GetExplicitMessage", "Arguments"="", "Data"=variant} ("API Command Cluster"), "Command"=API_Command_Enum."SetExplicitMessage", "Data"=w1599) -> (w1596:T6)
        n603 = call-dynamic "GenerateAPIEvent_Motor Controller.vi"("error in (no error)"=w1591, "API Command Cluster"=w1596, "Motor Controller In"=w1593) -> ("error out"=w1588:errorcluster)  [unwired: 6 in, 2 out]
        n604 = flat-sequence {
          tunnel: w1588 -> [_]
          frame #0 {
            w1602 = FALSE ("Jog (+)")
            n605 = local write "Jog (+)"(w1602) -> ()
            n606 = local write "Jog (-)"(w1602) -> ()
          }
        }
      }
      frame "----------DIO------------" {
      }
      frame "Initialize DO Devices" {
        n607 = Unbundle By Name(w1612) -> ("IO"=w1611:refnum<class "IO.lvclass">)
        n608 = call-dynamic "Set ICP1-DO Changed bit.vi"("error in (no error)"=w1608, "Value"=TRUE, "DO Channel"=ICP1-D0_Channel_Names."Servo ON", "IO in"=w1611) -> ("error out"=w1610:errorcluster, "IO out"=w1617:refnum<class "IO.lvclass">)  [unwired: 6 in]
        n609 = call-dynamic "Set ICP1-DO Changed bit.vi"("error in (no error)"=w1610, "Value"=FALSE, "DO Channel"=ICP1-D0_Channel_Names."Clear Stage Alarm", "IO in"=w1617) -> ("error out"=w1609:errorcluster)  [unwired: 6 in, 1 out]
      }
      frame "DO: Set ICP1-DO Status in UI" {
        n610 = Unbundle By Name(w1632) -> ("IO"=w1627:refnum<class "IO.lvclass">)
        n611 = call "DCON Action Engine.vi"("Action"=DCON_Action_Engine-States."Get Data" ("t"), "error in (no error)"=w1624, "Device Name"=Device_Names."ICP1-DO", "IO In"=w1627) -> ("error out"=w1623:errorcluster, "Status Out"=w1629:T42, "IO Out"=w1626:refnum<class "IO.lvclass">)  [unwired: 4 in, 1 out]
        n612 = Unbundle By Name(w1629) -> ("Digital Bits Value"=w1628:bool[])
        n613 = call-dynamic "Get Ordered Channels_Digital_Status_IO.vi"("error in (no error)"=w1623, "IO in"=w1626) -> ("error out"=w1631:errorcluster, "Ordered ICP1-DO Channels"=w1622:T10[])  [unwired: 5 in, 3 out]
        n614 = for {
          tunnel: w1628 -> [w1636] mode=indexing
          tunnel: w1622 -> [w1635] mode=indexing
          n615 = case shown="\"Purge Valve Open - R1\"" w1635 {
            tunnel: w1636 -> [_ w1637 w1638 w1639 w1640 w1641 w1642 w1643 w1644 w1645 w1646 w1647 w1648]
            frame "None", Default {
            }
            frame "Meniscus Pressure Reg PWR - R1" {
              "Meniscus Pressure Reg PWR - R1 Status" <- w1637
            }
            frame "Meniscus Pressure Reg PWR - R2" {
              "Meniscus Pressure Reg PWR - R2 Status" <- w1638
            }
            frame "Meniscus Pressure Reg PWR - R3" {
              "Meniscus Pressure Reg PWR - R3 Status" <- w1639
            }
            frame "Meniscus Pressure Reg PWR - R4" {
              "Meniscus Pressure Reg PWR - R4 Status" <- w1640
            }
            frame "Meniscus Pressure Reg PWR - R5" {
              "Meniscus Pressure Reg PWR - R5 Status" <- w1641
            }
            frame "Meniscus Pressure Reg PWR - R6" {
              "Meniscus Pressure Reg PWR - R6 Status" <- w1642
            }
            frame "Purge Valve Open - R1" {
              "Purge Valve Open - R1 Status" <- w1643
            }
            frame "Purge Valve Open - R2" {
              "Purge Valve Open - R2 Status" <- w1644
            }
            frame "Purge Valve Open - R3" {
              "Purge Valve Open - R3 Status" <- w1645
            }
            frame "Purge Valve Open - R4" {
              "Purge Valve Open - R4 Status" <- w1646
            }
            frame "Purge Valve Open - R5" {
              "Purge Valve Open - R5 Status" <- w1647
            }
            frame "Purge Valve Open - R6" {
              "Purge Valve Open - R6 Status" <- w1648
            }
          }
        }
      }
      frame "DI: Get ICP2 DI Status" {
        n616 = Unbundle By Name(w1660) -> ("IO"=w1657:refnum<class "IO.lvclass">)
        n617 = call "DCON Action Engine.vi"("Action"=DCON_Action_Engine-States."Get Data" ("t"), "error in (no error)"=w1655, "Device Name"=Device_Names."ICP2-DI", "IO In"=w1657) -> ("error out"=w1654:errorcluster, "Status Out"=w1652:T42, "IO Out"=w1653:refnum<class "IO.lvclass">)  [unwired: 4 in, 1 out]
        n618 = Unbundle By Name(w1652) -> ("Digital Bits Value"=w1651:bool[])
        n619 = call-dynamic "Get Ordered Channels_Digital_Status_IO.vi"("error in (no error)"=w1654, "IO in"=w1653) -> ("error out"=w1659:errorcluster, "Ordered ICP2-DI Channels"=w1650:T43[])  [unwired: 5 in, 3 out]
        n620 = for {
          tunnel: w1650 -> [w1664] mode=indexing
          tunnel: w1651 -> [w1663] mode=indexing
          n621 = case shown="\"SW - Ink Valve - R1\"" w1664 {
            tunnel: w1663 -> [_ w1665 w1666 w1667 w1668 w1669 w1670 w1671 w1672 w1673 w1674 w1675 w1676 w1677 w1678]
            frame "None", Default {
            }
            frame "SW - Ink Valve - R1" {
              "SW - Ink Valve - R1" <- w1665
            }
            frame "SW - Ink Valve - R2" {
              "SW - Ink Valve - R2" <- w1666
            }
            frame "SW - Ink Valve - R3" {
              "SW - Ink Valve - R3" <- w1667
            }
            frame "SW - Ink Valve - R4" {
              "SW - Ink Valve - R4" <- w1668
            }
            frame "SW - Ink Valve - R5" {
              "SW - Ink Valve - R5" <- w1669
            }
            frame "SW - Ink Valve - R6" {
              "SW - Ink Valve - R6" <- w1670
            }
            frame "SW - COVER INPUT SIDE" {
              "SW - COVER INPUT SIDE" <- w1671
              "SW - COVER INPUT SIDE (M)" <- w1671
            }
            frame "SW - COVER OUTPUT SIDE" {
              "SW - COVER OUTPUT SIDE" <- w1672
              "SW - COVER OUTPUT SIDE (M)" <- w1672
            }
            frame "SW - Purge - R1" {
              "SW - Purge - R1" <- w1673
            }
            frame "SW - Purge - R2" {
              "SW - Purge - R2" <- w1674
            }
            frame "SW - Purge - R3" {
              "SW - Purge - R3" <- w1675
            }
            frame "SW - Purge - R4" {
              "SW - Purge - R4" <- w1676
            }
            frame "SW - Purge - R5" {
              "SW - Purge - R5" <- w1677
            }
            frame "SW - Purge - R6" {
              "SW - Purge - R6" <- w1678
            }
          }
        }
      }
      frame "DO: Set ICP2-DO Status in UI" {
        n622 = Unbundle By Name(w1690) -> ("IO"=w1684:refnum<class "IO.lvclass">)
        n623 = call "DCON Action Engine.vi"("Action"=DCON_Action_Engine-States."Get Data" ("t"), "error in (no error)"=w1681, "Device Name"=Device_Names."ICP2-DO", "IO In"=w1684) -> ("error out"=w1680:errorcluster, "Status Out"=w1686:T42, "IO Out"=w1683:refnum<class "IO.lvclass">)  [unwired: 4 in, 1 out]
        n624 = Unbundle By Name(w1686) -> ("Digital Bits Value"=w1685:bool[])
        n625 = call-dynamic "Get Ordered Channels_Digital_Status_IO.vi"("error in (no error)"=w1680, "IO in"=w1683) -> ("error out"=w1689:errorcluster, "Ordered ICP2-DO Channels"=w1688:T9[])  [unwired: 5 in, 3 out]
        n626 = for {
          tunnel: w1688 -> [w1694] mode=indexing
          tunnel: w1685 -> [w1693] mode=indexing
          n627 = case shown="\"Meniscus Valve Open - R1\"" w1694 {
            tunnel: w1693 -> [_ w1695 w1696 w1697 w1698 w1699 w1700 w1701 w1702 w1703 w1704 w1705 w1706 w1707 w1708 w1709 w1710 w1711 w1712 w1713 w1714 w1715 w1716 w1717 w1718]
            frame "None", Default {
            }
            frame "Meniscus Valve Open - R1" {
              "Meniscus Valve Open - R1 Status" <- w1695
            }
            frame "Meniscus Valve Open - R2" {
              "Meniscus Valve Open - R2 Status" <- w1696
            }
            frame "Meniscus Valve Open - R3" {
              "Meniscus Valve Open - R3 Status" <- w1697
            }
            frame "Meniscus Valve Open - R4" {
              "Meniscus Valve Open - R4 Status" <- w1698
            }
            frame "Meniscus Valve Open - R5" {
              "Meniscus Valve Open - R5 Status" <- w1699
            }
            frame "Meniscus Valve Open - R6" {
              "Meniscus Valve Open - R6 Status" <- w1700
            }
            frame "Ink Flow Valve Open - R1" {
              "Ink Flow Valve Open - R1 Status" <- w1701
            }
            frame "Ink Flow Valve Open - R2" {
              "Ink Flow Valve Open - R2 Status" <- w1702
            }
            frame "Ink Flow Valve Open - R3" {
              "Ink Flow Valve Open - R3 Status" <- w1703
            }
            frame "Ink Flow Valve Open - R4" {
              "Ink Flow Valve Open - R4 Status" <- w1704
            }
            frame "Ink Flow Valve Open - R5" {
              "Ink Flow Valve Open - R5 Status" <- w1705
            }
            frame "Ink Flow Valve Open - R6" {
              "Ink Flow Valve Open - R6 Status" <- w1706
            }
            frame "SW_LED - Ink Valve - R1" {
              "SW_LED - Ink Valve - R1 Status" <- w1707
            }
            frame "SW_LED - Ink Valve - R2" {
              "SW_LED - Ink Valve - R2 Status" <- w1708
            }
            frame "SW_LED - Ink Valve - R3" {
              "SW_LED - Ink Valve - R3 Status" <- w1709
            }
            frame "SW_LED - Ink Valve - R4" {
              "SW_LED - Ink Valve - R4 Status" <- w1710
            }
            frame "SW_LED - Ink Valve - R5" {
              "SW_LED - Ink Valve - R5 Status" <- w1711
            }
            frame "SW_LED - Ink Valve - R6" {
              "SW_LED - Ink Valve - R6 Status" <- w1712
            }
            frame "Recirc Pump On - R1" {
              "Recirc Pump On - R1 Status" <- w1713
            }
            frame "Recirc Pump On - R2" {
              "Recirc Pump On - R2 Status" <- w1714
            }
            frame "Recirc Pump On - R3" {
              "Recirc Pump On - R3 Status" <- w1715
            }
            frame "Recirc Pump On - R4" {
              "Recirc Pump On - R4 Status" <- w1716
            }
            frame "Recirc Pump On - R5" {
              "Recirc Pump On - R5 Status" <- w1717
            }
            frame "Recirc Pump On - R6" {
              "Recirc Pump On - R6 Status" <- w1718
            }
          }
        }
      }
      frame "----------AIO-----------" {
      }
      frame "AI: Get ICP1 AI Status" {
        n628 = Unbundle By Name(w1735) -> ("IO"=w1732:refnum<class "IO.lvclass">)
        n629 = call "DCON Action Engine.vi"("Action"=DCON_Action_Engine-States."Get Data" ("t"), "error in (no error)"=w1730, "Device Name"=Device_Names."ICP1-AI", "IO In"=w1732) -> ("error out"=w1729:errorcluster, "Status Out"=w1727:T42, "IO Out"=w1728:refnum<class "IO.lvclass">)  [unwired: 4 in, 1 out]
        n630 = Unbundle By Name(w1727) -> ("Analog Values"=w1726:dbl[])
        n631 = call-dynamic "Get Ordered Channels_Analog_Status_IO.vi"("error in (no error)"=w1729, "IO in"=w1728) -> ("error out"=w1734:errorcluster, "Ordered ICP1-AO Channels"=w1725:T14[])  [unwired: 5 in, 3 out]
        n632 = for {
          tunnel: w1725 -> [w1739] mode=indexing
          tunnel: w1726 -> [w1738] mode=indexing
          n633 = case shown="\"Meniscus Pressure Set - R6\"" w1739 {
            tunnel: w1738 -> [_ w1740 w1741 w1742 w1743 w1744 w1745]
            frame "None", Default {
            }
            frame "Meniscus Pressure Set - R1" {
              "Meniscus Pressure Read - R1" <- w1740
            }
            frame "Meniscus Pressure Set - R2" {
              "Meniscus Pressure Read - R2" <- w1741
            }
            frame "Meniscus Pressure Set - R3" {
              "Meniscus Pressure Read - R3" <- w1742
            }
            frame "Meniscus Pressure Set - R4" {
              "Meniscus Pressure Read - R4" <- w1743
            }
            frame "Meniscus Pressure Set - R5" {
              "Meniscus Pressure Read - R5" <- w1744
            }
            frame "Meniscus Pressure Set - R6" {
              "Meniscus Pressure Read - R6" <- w1745
            }
          }
        }
      }
      frame "AO: Set ICP1-AO Status in UI" {
        n634 = Unbundle By Name(w1757) -> ("IO"=w1752:refnum<class "IO.lvclass">)
        n635 = call "DCON Action Engine.vi"("Action"=DCON_Action_Engine-States."Get Data" ("t"), "error in (no error)"=w1749, "Device Name"=Device_Names."ICP1-AO", "IO In"=w1752) -> ("error out"=w1748:errorcluster, "Status Out"=w1754:T42, "IO Out"=w1751:refnum<class "IO.lvclass">)  [unwired: 4 in, 1 out]
        n636 = Unbundle By Name(w1754) -> ("Analog Values"=w1753:dbl[])
        n637 = call-dynamic "Get Ordered Channels_Analog_Status_IO.vi"("error in (no error)"=w1748, "IO in"=w1751) -> ("error out"=w1756:errorcluster, "Ordered ICP1-AO Channels"=w1747:T14[])  [unwired: 5 in, 3 out]
        n638 = for {
          tunnel: w1753 -> [w1760] mode=indexing
          tunnel: w1747 -> [w1761] mode=indexing
          n639 = case shown="\"None\", Default" w1761 {
            tunnel: w1760 -> [_ w1762 w1763 w1764 w1765 w1766 w1767]
            frame "None", Default {
            }
            frame "Meniscus Pressure Set - R1" {
              "Meniscus Pressure Set - R1 Status" <- w1762
            }
            frame "Meniscus Pressure Set - R2" {
              "Meniscus Pressure Set - R2 Status" <- w1763
            }
            frame "Meniscus Pressure Set - R3" {
              "Meniscus Pressure Set - R3 Status" <- w1764
            }
            frame "Meniscus Pressure Set - R4" {
              "Meniscus Pressure Set - R4 Status" <- w1765
            }
            frame "Meniscus Pressure Set - R5" {
              "Meniscus Pressure Set - R5 Status" <- w1766
            }
            frame "Meniscus Pressure Set - R6" {
              "Meniscus Pressure Set - R6 Status" <- w1767
            }
          }
        }
      }
      frame "AO: Set ICP2-AO Status in UI" {
        n640 = Unbundle By Name(w1779) -> ("IO"=w1774:refnum<class "IO.lvclass">)
        n641 = call "DCON Action Engine.vi"("Action"=DCON_Action_Engine-States."Get Data" ("t"), "error in (no error)"=w1771, "Device Name"=Device_Names."ICP2-AO", "IO In"=w1774) -> ("error out"=w1770:errorcluster, "Status Out"=w1776:T42, "IO Out"=w1773:refnum<class "IO.lvclass">)  [unwired: 4 in, 1 out]
        n642 = Unbundle By Name(w1776) -> ("Analog Values"=w1775:dbl[])
        n643 = call-dynamic "Get Ordered Channels_Analog_Status_IO.vi"("error in (no error)"=w1770, "IO in"=w1773) -> ("error out"=w1778:errorcluster, "Ordered ICP2-AO Channels"=w1769:T15[])  [unwired: 5 in, 3 out]
        n644 = for {
          tunnel: w1775 -> [w1782] mode=indexing
          tunnel: w1769 -> [w1783] mode=indexing
          n645 = case shown="\"Recirc Pump Flow Set - R1\"" w1783 {
            tunnel: w1782 -> [_ w1784 w1785 w1786 w1787 w1788 w1789]
            frame "None", Default {
            }
            frame "Recirc Pump Flow Set - R1" {
              "Recirc Pump Flow Set - R1 Status" <- w1784
            }
            frame "Recirc Pump Flow Set - R2" {
              "Recirc Pump Flow Set - R2 Status" <- w1785
            }
            frame "Recirc Pump Flow Set - R3" {
              "Recirc Pump Flow Set - R3 Status" <- w1786
            }
            frame "Recirc Pump Flow Set - R4" {
              "Recirc Pump Flow Set - R4 Status" <- w1787
            }
            frame "Recirc Pump Flow Set - R5" {
              "Recirc Pump Flow Set - R5 Status" <- w1788
            }
            frame "Recirc Pump Flow Set - R6" {
              "Recirc Pump Flow Set - R6 Status" <- w1789
            }
          }
        }
      }
      frame "-----------Init-------------" {
      }
      frame "Init: Read ICP1-DO" {
        n646 = Unbundle By Name(w1806) -> ("IO"=w1802:refnum<class "IO.lvclass">)
        n647 = call "DCON Action Engine.vi"("Action"=DCON_Action_Engine-States."Get Digital Status" ("t"), "error in (no error)"=w1799, "Device Name"=Device_Names."ICP1-DO", "IO In"=w1802) -> ("error out"=w1798:errorcluster, "Status Out"=w1803:T42, "IO Out"=w1801:refnum<class "IO.lvclass">)  [unwired: 4 in, 1 out]
        n648 = Unbundle By Name(w1803) -> ("Digital Bits Value"=w1796:bool[])
        n649 = call-dynamic "Get Ordered Channels_Digital_Status_IO.vi"("error in (no error)"=w1798, "IO in"=w1801) -> ("error out"=w1805:errorcluster, "Ordered ICP1-DO Channels"=w1795:T10[])  [unwired: 5 in, 3 out]
        n650 = for {
          tunnel: w1796 -> [w1810] mode=indexing
          tunnel: w1795 -> [w1809] mode=indexing
          n651 = case shown="\"Purge Valve Open - R1\"" w1809 {
            tunnel: w1810 -> [_ w1811 w1812 w1813 w1814 w1815 w1816 w1817 w1818 w1819 w1820 w1821 w1822]
            frame "None", Default {
            }
            frame "Meniscus Pressure Reg PWR - R1" {
              n652 = local write "Meniscus Pressure Reg PWR - R1"(w1811) -> ()
            }
            frame "Meniscus Pressure Reg PWR - R2" {
              n653 = local write "Meniscus Pressure Reg PWR - R2"(w1812) -> ()
            }
            frame "Meniscus Pressure Reg PWR - R3" {
              n654 = local write "Meniscus Pressure Reg PWR - R3"(w1813) -> ()
            }
            frame "Meniscus Pressure Reg PWR - R4" {
              n655 = local write "Meniscus Pressure Reg PWR - R4"(w1814) -> ()
            }
            frame "Meniscus Pressure Reg PWR - R5" {
              n656 = local write "Meniscus Pressure Reg PWR - R5"(w1815) -> ()
            }
            frame "Meniscus Pressure Reg PWR - R6" {
              n657 = local write "Meniscus Pressure Reg PWR - R6"(w1816) -> ()
            }
            frame "Purge Valve Open - R1" {
              n658 = local write "Purge Valve Open - R1"(w1817) -> ()
            }
            frame "Purge Valve Open - R2" {
              n659 = local write "Purge Valve Open - R2"(w1818) -> ()
            }
            frame "Purge Valve Open - R3" {
              n660 = local write "Purge Valve Open - R3"(w1819) -> ()
            }
            frame "Purge Valve Open - R4" {
              n661 = local write "Purge Valve Open - R4"(w1820) -> ()
            }
            frame "Purge Valve Open - R5" {
              n662 = local write "Purge Valve Open - R5"(w1821) -> ()
            }
            frame "Purge Valve Open - R6" {
              n663 = local write "Purge Valve Open - R6"(w1822) -> ()
            }
          }
        }
      }
      frame "Init: Read ICP2-DO" {
        n664 = Unbundle By Name(w1834) -> ("IO"=w1830:refnum<class "IO.lvclass">)
        n665 = call "DCON Action Engine.vi"("Action"=DCON_Action_Engine-States."Get Digital Status" ("t"), "error in (no error)"=w1827, "Device Name"=Device_Names."ICP2-DO", "IO In"=w1830) -> ("error out"=w1826:errorcluster, "Status Out"=w1831:T42, "IO Out"=w1829:refnum<class "IO.lvclass">)  [unwired: 4 in, 1 out]
        n666 = Unbundle By Name(w1831) -> ("Digital Bits Value"=w1824:bool[])
        n667 = call-dynamic "Get Ordered Channels_Digital_Status_IO.vi"("error in (no error)"=w1826, "IO in"=w1829) -> ("error out"=w1833:errorcluster, "Ordered ICP2-DO Channels"=w1823:T9[])  [unwired: 5 in, 3 out]
        n668 = for {
          tunnel: w1823 -> [w1838] mode=indexing
          tunnel: w1824 -> [w1837] mode=indexing
          n669 = case shown="\"Meniscus Valve Open - R2\"" w1838 {
            tunnel: w1837 -> [_ w1839 w1840 w1841 w1842 w1843 w1844 w1845 w1846 w1847 w1848 w1849 w1850 w1851 w1852 w1853 w1854 w1855 w1856 w1857 w1858 w1859 w1860 w1861 w1862]
            frame "None", Default {
            }
            frame "Meniscus Valve Open - R1" {
              n670 = local write "Meniscus Valve Open - R1"(w1839) -> ()
            }
            frame "Meniscus Valve Open - R2" {
              n671 = local write "Meniscus Valve Open - R2"(w1840) -> ()
            }
            frame "Meniscus Valve Open - R3" {
              n672 = local write "Meniscus Valve Open - R3"(w1841) -> ()
            }
            frame "Meniscus Valve Open - R4" {
              n673 = local write "Meniscus Valve Open - R4"(w1842) -> ()
            }
            frame "Meniscus Valve Open - R5" {
              n674 = local write "Meniscus Valve Open - R5"(w1843) -> ()
            }
            frame "Meniscus Valve Open - R6" {
              n675 = local write "Meniscus Valve Open - R6"(w1844) -> ()
            }
            frame "Ink Flow Valve Open - R1" {
              n676 = local write "Ink Flow Valve Open - R1"(w1845) -> ()
            }
            frame "Ink Flow Valve Open - R2" {
              n677 = local write "Ink Flow Valve Open - R2"(w1846) -> ()
            }
            frame "Ink Flow Valve Open - R3" {
              n678 = local write "Ink Flow Valve Open - R3"(w1847) -> ()
            }
            frame "Ink Flow Valve Open - R4" {
              n679 = local write "Ink Flow Valve Open - R4"(w1848) -> ()
            }
            frame "Ink Flow Valve Open - R5" {
              n680 = local write "Ink Flow Valve Open - R5"(w1849) -> ()
            }
            frame "Ink Flow Valve Open - R6" {
              n681 = local write "Ink Flow Valve Open - R6"(w1850) -> ()
            }
            frame "SW_LED - Ink Valve - R1" {
              n682 = local write "SW_LED - Ink Valve - R1"(w1851) -> ()
            }
            frame "SW_LED - Ink Valve - R2" {
              n683 = local write "SW_LED - Ink Valve - R2"(w1852) -> ()
            }
            frame "SW_LED - Ink Valve - R3" {
              n684 = local write "SW_LED - Ink Valve - R3"(w1853) -> ()
            }
            frame "SW_LED - Ink Valve - R4" {
              n685 = local write "SW_LED - Ink Valve - R4"(w1854) -> ()
            }
            frame "SW_LED - Ink Valve - R5" {
              n686 = local write "SW_LED - Ink Valve - R5"(w1855) -> ()
            }
            frame "SW_LED - Ink Valve - R6" {
              n687 = local write "SW_LED - Ink Valve - R6"(w1856) -> ()
            }
            frame "Recirc Pump On - R1" {
              n688 = local write "Recirc Pump On - R1"(w1857) -> ()
            }
            frame "Recirc Pump On - R2" {
              n689 = local write "Recirc Pump On - R2"(w1858) -> ()
            }
            frame "Recirc Pump On - R3" {
              n690 = local write "Recirc Pump On - R3"(w1859) -> ()
            }
            frame "Recirc Pump On - R4" {
              n691 = local write "Recirc Pump On - R4"(w1860) -> ()
            }
            frame "Recirc Pump On - R5" {
              n692 = local write "Recirc Pump On - R5"(w1861) -> ()
            }
            frame "Recirc Pump On - R6" {
              n693 = local write "Recirc Pump On - R6"(w1862) -> ()
            }
          }
        }
      }
      frame "Init: Read ICP1-AO" {
        n694 = Unbundle By Name(w1874) -> ("IO"=w1870:refnum<class "IO.lvclass">)
        n695 = call "DCON Action Engine.vi"("Action"=DCON_Action_Engine-States."Get AO Status" ("t"), "error in (no error)"=w1867, "Device Name"=Device_Names."ICP1-AO", "IO In"=w1870) -> ("error out"=w1866:errorcluster, "Status Out"=w1871:T42, "IO Out"=w1869:refnum<class "IO.lvclass">)  [unwired: 4 in, 1 out]
        n696 = Unbundle By Name(w1871) -> ("Analog Values"=w1864:dbl[])
        n697 = call-dynamic "Get Ordered Channels_Analog_Status_IO.vi"("error in (no error)"=w1866, "IO in"=w1869) -> ("error out"=w1873:errorcluster, "Ordered ICP1-AO Channels"=w1863:T14[])  [unwired: 5 in, 3 out]
        n698 = for {
          tunnel: w1864 -> [w1877] mode=indexing
          tunnel: w1863 -> [w1878] mode=indexing
          n699 = case shown="\"Meniscus Pressure Set - R6\"" w1878 {
            tunnel: w1877 -> [_ w1879 w1880 w1881 w1882 w1883 w1884]
            frame "None", Default {
            }
            frame "Meniscus Pressure Set - R1" {
              n700 = local write "Meniscus Pressure Set - R1"(w1879) -> ()
            }
            frame "Meniscus Pressure Set - R2" {
              n701 = local write "Meniscus Pressure Set - R2"(w1880) -> ()
            }
            frame "Meniscus Pressure Set - R3" {
              n702 = local write "Meniscus Pressure Set - R3"(w1881) -> ()
            }
            frame "Meniscus Pressure Set - R4" {
              n703 = local write "Meniscus Pressure Set - R4"(w1882) -> ()
            }
            frame "Meniscus Pressure Set - R5" {
              n704 = local write "Meniscus Pressure Set - R5"(w1883) -> ()
            }
            frame "Meniscus Pressure Set - R6" {
              n705 = local write "Meniscus Pressure Set - R6"(w1884) -> ()
            }
          }
        }
      }
      frame "Init: Read ICP2-AO" {
        n706 = Unbundle By Name(w1896) -> ("IO"=w1892:refnum<class "IO.lvclass">)
        n707 = call "DCON Action Engine.vi"("Action"=DCON_Action_Engine-States."Get Data" ("t"), "error in (no error)"=w1889, "Device Name"=Device_Names."ICP2-AO", "IO In"=w1892) -> ("error out"=w1888:errorcluster, "Status Out"=w1893:T42, "IO Out"=w1891:refnum<class "IO.lvclass">)  [unwired: 4 in, 1 out]
        n708 = Unbundle By Name(w1893) -> ("Analog Values"=w1886:dbl[])
        n709 = call-dynamic "Get Ordered Channels_Analog_Status_IO.vi"("error in (no error)"=w1888, "IO in"=w1891) -> ("error out"=w1895:errorcluster, "Ordered ICP2-AO Channels"=w1885:T15[])  [unwired: 5 in, 3 out]
        n710 = for {
          tunnel: w1886 -> [w1899] mode=indexing
          tunnel: w1885 -> [w1900] mode=indexing
          n711 = case shown="\"Recirc Pump Flow Set - R6\"" w1900 {
            tunnel: w1899 -> [_ w1901 w1902 w1903 w1904 w1905 w1906]
            frame "None", Default {
            }
            frame "Recirc Pump Flow Set - R1" {
              n712 = local write "Recirc Pump Flow Set - R1"(w1901) -> ()
            }
            frame "Recirc Pump Flow Set - R2" {
              n713 = local write "Recirc Pump Flow Set - R2"(w1902) -> ()
            }
            frame "Recirc Pump Flow Set - R3" {
              n714 = local write "Recirc Pump Flow Set - R3"(w1903) -> ()
            }
            frame "Recirc Pump Flow Set - R4" {
              n715 = local write "Recirc Pump Flow Set - R4"(w1904) -> ()
            }
            frame "Recirc Pump Flow Set - R5" {
              n716 = local write "Recirc Pump Flow Set - R5"(w1905) -> ()
            }
            frame "Recirc Pump Flow Set - R6" {
              n717 = local write "Recirc Pump Flow Set - R6"(w1906) -> ()
            }
          }
        }
      }
      frame "--------Purge---------" {
      }
      frame "Purge: Send API" {
        n718 = Unbundle By Name(w1918) -> ("IO"=w1917:refnum<class "IO.lvclass">, "Purge\\PrePurge Channel Name"=w1914:T10)
        n719 = call-dynamic "Purge PH - API.vi"("Wait (F)"=FALSE, "error in (no error)"=w1915, "Duration (s)"="Duration (s)", "ICP1-DO Channel Name"=w1914, "IO in"=w1917) -> ("error out"=w1916:errorcluster)  [unwired: 5 in, 1 out]
      }
      frame "------Pre Purge-----" {
      }
      frame "Pre Purge: Send API" {
        n720 = Unbundle By Name(w1936) -> ("Pre Purge Parameters.No. of Repeats"=w1928:i32, "Pre Purge Parameters.GIS File Path"=w1931:path, "Pre Purge Parameters.Duration (s)"=w1930:dbl, "Purge\\PrePurge Channel Name"=w1929:T10)
        n721 = call-dynamic "Pre Purge API.vi"("Repeats"=w1928, "ICP1-DO Channel Names"=w1929, "PurgeDuration (s)"="PPDuration (s)", "error in (no error)"=w1932, "Duration (s)"=w1930, "GIS File Path"=w1931, "TopLevel in"=w1934) -> ("error out"=w1933:errorcluster, "TopLevel out"=w1935:refnum<class "TopLevel.lvclass">)  [unwired: 3 in]
      }
      frame "---------Ink Channel-------" {
      }
      frame "Ink: Send Channel Command" {
        n722 = Unbundle By Name(w1945) -> ("API Command"=w1944:T8)
        n723 = Bundle By Name(cluster=T12 {"Command"=enum."Execute Printer Commands", "Arguments"="", "Data"=variant} ("API Command Cluster"), "Command"=w1944) -> (w1946:T12)
        n724 = call-dynamic "GenerateAPIEvent_TopLevel.vi"("error in (no error)"=w1948, "API Command Cluster"=w1946, "TopLevel in"=w1950) -> ("error out"=w1949:errorcluster, "TopLevel out"=w1951:refnum<class "TopLevel.lvclass">)  [unwired: 7 in]
      }
    }
  }
  "TopLevel Out" <- w1
